vi "TrackingRedDot.vi"() -> ()   [LabVIEW 2024]
uses:
  <userlib>/ImageProcessing/IdentifyBlob_Square_Image.vi
panel:
  out "Array":cluster{"Numeric":dbl, "Numeric 2":dbl}[](array[cluster])=[{"Numeric"=343.3711790393013, "Numeric 2"=267.07423580786025}, {"Numeric"=337.0897435897436, "Numeric 2"=269.14102564102564}, {"Numeric"=335.8137651821862, "Numeric 2"=268.5991902834008}, {"Numeric"=343.1166666666667, "Numeric 2"=267.30833333333334}, {"Numeric"=348.0122448979592, "Numeric 2"=265.46530612244896}, {"Numeric"=344.37130801687766, "Numeric 2"=265.1898734177215}, {"Numeric"=338.55274261603375, "Numeric 2"=267.34599156118145}, {"Numeric"=337.68879668049794, "Numeric 2"=268.78008298755185}, {"Numeric"=340.15744680851066, "Numeric 2"=268.4382978723404}, {"Numeric"=345.2207792207792, "Numeric 2"=267.05627705627705}, {"Numeric"=343.76190476190476, "Numeric 2"=265.09090909090907}, {"Numeric"=340.12345679012344, "Numeric 2"=265.4074074074074}, {"Numeric"=340.2276422764228, "Numeric 2"=267.4349593495935}, {"Numeric"=341.6163793103448, "Numeric 2"=269.10775862068965}, {"Numeric"=341.60084033613447, "Numeric 2"=268.327731092437}, {"Numeric"=340.8185654008439, "Numeric 2"=266.56540084388183}, {"Numeric"=340.336170212766, "Numeric 2"=265.2893617021277}, {"Numeric"=341.6900826446281, "Numeric 2"=265.8636363636364}, {"Numeric"=342.0576131687243, "Numeric 2"=267.6296296296296}, {"Numeric"=340.67932489451476, "Numeric 2"=268.8270042194093}, {"Numeric"=339.1673640167364, "Numeric 2"=267.55648535564853}, {"Numeric"=339.72294372294374, "Numeric 2"=266.15584415584414}, {"Numeric"=341.9240506329114, "Numeric 2"=265.2742616033755}, {"Numeric"=343.8050847457627, "Numeric 2"=266.9364406779661}, {"Numeric"=342.1652892561983, "Numeric 2"=268.5}, {"Numeric"=338.8601694915254, "Numeric 2"=268.23728813559325}, {"Numeric"=338.6923076923077, "Numeric 2"=267.15811965811963}, {"Numeric"=343.2983870967742, "Numeric 2"=265.68951612903226}, {"Numeric"=345.4567901234568, "Numeric 2"=265.86831275720164}, {"Numeric"=343.94142259414224, "Numeric 2"=267.3305439330544}, {"Numeric"=338.93004115226336, "Numeric 2"=268.4320987654321}, {"Numeric"=337.390243902439, "Numeric 2"=267.7032520325203}, {"Numeric"=340.9665271966527, "Numeric 2"=266.7615062761506}, {"Numeric"=345.13675213675214, "Numeric 2"=266.15384615384613}, {"Numeric"=346.1016260162602, "Numeric 2"=265.7967479674797}, {"Numeric"=345.79918032786884, "Numeric 2"=266.2663934426229}, {"Numeric"=342.5042016806723, "Numeric 2"=267.06722689075633}, {"Numeric"=340.68595041322317, "Numeric 2"=267.4297520661157}, {"Numeric"=339.0365853658537, "Numeric 2"=267.760162601626}, {"Numeric"=338.1623931623932, "Numeric 2"=268.1025641025641}, {"Numeric"=338.4458333333333, "Numeric 2"=267.9625}, {"Numeric"=338.8691983122363, "Numeric 2"=267.9831223628692}, {"Numeric"=339.4268292682927, "Numeric 2"=267.5853658536585}, {"Numeric"=340.4530612244898, "Numeric 2"=267.52244897959184}, {"Numeric"=341.6302521008403, "Numeric 2"=267.33193277310926}, {"Numeric"=342.9958158995816, "Numeric 2"=266.74058577405856}, {"Numeric"=342.9958158995816, "Numeric 2"=266.74058577405856}, {"Numeric"=344.2236286919831, "Numeric 2"=266.55274261603375}, {"Numeric"=344.7909836065574, "Numeric 2"=266.4303278688525}, {"Numeric"=345.0468085106383, "Numeric 2"=266.2340425531915}, {"Numeric"=345.1603375527426, "Numeric 2"=266.0337552742616}, {"Numeric"=345.48319327731093, "Numeric 2"=265.99159663865544}, {"Numeric"=345.68200836820085, "Numeric 2"=265.9916317991632}, {"Numeric"=345.50416666666666, "Numeric 2"=266.0708333333333}, {"Numeric"=345.43388429752065, "Numeric 2"=265.91735537190084}, {"Numeric"=345.2307692307692, "Numeric 2"=265.83805668016197}, {"Numeric"=344.9428571428571, "Numeric 2"=265.869387755102}, {"Numeric"=344.5420168067227, "Numeric 2"=266.01680672268907}, {"Numeric"=344.4579831932773, "Numeric 2"=266.07142857142856}, {"Numeric"=344.26808510638296, "Numeric 2"=266.20851063829787}, {"Numeric"=343.61965811965814, "Numeric 2"=266.1880341880342}, {"Numeric"=343.0420168067227, "Numeric 2"=266.2352941176471}, {"Numeric"=342.40677966101697, "Numeric 2"=266.29661016949154}, {"Numeric"=342.1991701244813, "Numeric 2"=266.45228215767634}, {"Numeric"=341.6846473029046, "Numeric 2"=266.5435684647303}, {"Numeric"=341.12133891213387, "Numeric 2"=266.78661087866107}, {"Numeric"=340.73390557939916, "Numeric 2"=266.9785407725322}, {"Numeric"=339.8933333333333, "Numeric 2"=267.05333333333334}, {"Numeric"=339.8933333333333, "Numeric 2"=267.05333333333334}, {"Numeric"=339.60084033613447, "Numeric 2"=267.3067226890756}, {"Numeric"=339.5611814345992, "Numeric 2"=267.295358649789}, {"Numeric"=339.508064516129, "Numeric 2"=267.59274193548384}, {"Numeric"=339.4475806451613, "Numeric 2"=267.5443548387097}, {"Numeric"=339.4475806451613, "Numeric 2"=267.5443548387097}, {"Numeric"=339.16806722689074, "Numeric 2"=267.8151260504202}, {"Numeric"=339.3703703703704, "Numeric 2"=267.9835390946502}, {"Numeric"=339.45147679324896, "Numeric 2"=268.1940928270042}, {"Numeric"=339.63713080168776, "Numeric 2"=268.25738396624473}, {"Numeric"=340.12133891213387, "Numeric 2"=268.10460251046027}, {"Numeric"=339.9324894514768, "Numeric 2"=268.0590717299578}, {"Numeric"=340.11297071129707, "Numeric 2"=267.9623430962343}, {"Numeric"=341.198347107438, "Numeric 2"=268.004132231405}, {"Numeric"=341.6170212765957, "Numeric 2"=267.9404255319149}, {"Numeric"=342.01659751037346, "Numeric 2"=267.76348547717845}, {"Numeric"=342.0082304526749, "Numeric 2"=267.6872427983539}, {"Numeric"=342.5162601626016, "Numeric 2"=267.5609756097561}, {"Numeric"=342.5162601626016, "Numeric 2"=267.5609756097561}, {"Numeric"=342.8512396694215, "Numeric 2"=267.3801652892562}, {"Numeric"=342.8512396694215, "Numeric 2"=267.3801652892562}, {"Numeric"=343.22222222222223, "Numeric 2"=267.2478632478632}, {"Numeric"=343.10526315789474, "Numeric 2"=267.0043859649123}, {"Numeric"=343.0295358649789, "Numeric 2"=266.75949367088606}, {"Numeric"=343.5163934426229, "Numeric 2"=266.5983606557377}, {"Numeric"=343.64406779661016, "Numeric 2"=266.53389830508473}, {"Numeric"=343.6846473029046, "Numeric 2"=266.448132780083}, {"Numeric"=343.40677966101697, "Numeric 2"=266.33474576271186}, {"Numeric"=343.51724137931035, "Numeric 2"=266.2155172413793}, {"Numeric"=343.2436974789916, "Numeric 2"=265.93277310924367}, {"Numeric"=343.23770491803276, "Numeric 2"=265.8032786885246}, {"Numeric"=343.0082304526749, "Numeric 2"=265.8395061728395}, {"Numeric"=342.83613445378154, "Numeric 2"=265.80252100840335}, {"Numeric"=342.38429752066116, "Numeric 2"=265.72314049586777}, {"Numeric"=342.38429752066116, "Numeric 2"=265.72314049586777}, {"Numeric"=341.76050420168065, "Numeric 2"=265.6932773109244}, {"Numeric"=341.9, "Numeric 2"=265.8}, {"Numeric"=341.6848739495798, "Numeric 2"=265.94117647058823}, {"Numeric"=341.0219298245614, "Numeric 2"=266.1798245614035}, {"Numeric"=340.9957081545064, "Numeric 2"=266.2961373390558}, {"Numeric"=340.6864406779661, "Numeric 2"=266.385593220339}, {"Numeric"=340.2340425531915, "Numeric 2"=266.45106382978724}, {"Numeric"=340.4978902953587, "Numeric 2"=266.55274261603375}, {"Numeric"=340.24050632911394, "Numeric 2"=266.8565400843882}, {"Numeric"=340.54741379310343, "Numeric 2"=267.0689655172414}, {"Numeric"=340.53711790393015, "Numeric 2"=267.1528384279476}, {"Numeric"=340.49568965517244, "Numeric 2"=267.25}, {"Numeric"=340.49568965517244, "Numeric 2"=267.25}, {"Numeric"=340.61728395061726, "Numeric 2"=267.4650205761317}, {"Numeric"=340.5983606557377, "Numeric 2"=267.577868852459}, {"Numeric"=340.5983606557377, "Numeric 2"=267.577868852459}, {"Numeric"=341.33613445378154, "Numeric 2"=267.76050420168065}, {"Numeric"=341.44166666666666, "Numeric 2"=267.84166666666664}, {"Numeric"=341.6652719665272, "Numeric 2"=267.8619246861925}, {"Numeric"=341.6313559322034, "Numeric 2"=267.978813559322}, {"Numeric"=341.77292576419217, "Numeric 2"=268.2139737991266}, {"Numeric"=341.965367965368, "Numeric 2"=268.2294372294372}, {"Numeric"=341.93886462882097, "Numeric 2"=268.1877729257642}, {"Numeric"=342.1025641025641, "Numeric 2"=268.0726495726496}, {"Numeric"=342.3151260504202, "Numeric 2"=267.9621848739496}, {"Numeric"=342.0258620689655, "Numeric 2"=267.9439655172414}, {"Numeric"=342.3801652892562, "Numeric 2"=267.8388429752066}, {"Numeric"=342.3801652892562, "Numeric 2"=267.8388429752066}, {"Numeric"=342.2716049382716, "Numeric 2"=267.59670781893004}, {"Numeric"=342.4074074074074, "Numeric 2"=267.4156378600823}, {"Numeric"=342.4074074074074, "Numeric 2"=267.4156378600823}, {"Numeric"=342.10775862068965, "Numeric 2"=267.23706896551727}, {"Numeric"=342.2920353982301, "Numeric 2"=267.1061946902655}, {"Numeric"=342.2324561403509, "Numeric 2"=267.00877192982455}, {"Numeric"=342.14285714285717, "Numeric 2"=266.6344537815126}, {"Numeric"=341.89121338912133, "Numeric 2"=266.4728033472803}, {"Numeric"=341.864406779661, "Numeric 2"=266.34322033898303}, {"Numeric"=341.75536480686696, "Numeric 2"=266.2575107296137}, {"Numeric"=341.8663793103448, "Numeric 2"=266.2198275862069}, {"Numeric"=341.6523605150215, "Numeric 2"=266.15450643776825}, {"Numeric"=341.1965065502183, "Numeric 2"=266.07860262008734}, {"Numeric"=341.24896265560164, "Numeric 2"=265.8381742738589}, {"Numeric"=341.24896265560164, "Numeric 2"=265.8381742738589}, {"Numeric"=341.16170212765957, "Numeric 2"=265.88510638297873}, {"Numeric"=341.1673640167364, "Numeric 2"=265.93305439330544}, {"Numeric"=341.1673640167364, "Numeric 2"=265.93305439330544}, {"Numeric"=341.29957805907173, "Numeric 2"=266.084388185654}, {"Numeric"=341.46610169491527, "Numeric 2"=265.96610169491527}, {"Numeric"=341.4051724137931, "Numeric 2"=266.12931034482756}, {"Numeric"=341.3974358974359, "Numeric 2"=266.2393162393162}, {"Numeric"=341.50847457627117, "Numeric 2"=266.364406779661}, {"Numeric"=341.50622406639, "Numeric 2"=266.50622406639}, {"Numeric"=341.4813278008299, "Numeric 2"=266.53941908713693}, {"Numeric"=341.7375, "Numeric 2"=266.6333333333333}, {"Numeric"=341.7543859649123, "Numeric 2"=266.890350877193}, {"Numeric"=341.93886462882097, "Numeric 2"=267.117903930131}, {"Numeric"=342.10743801652893, "Numeric 2"=267.3223140495868}, {"Numeric"=342.22314049586777, "Numeric 2"=267.41735537190084}, {"Numeric"=342.27755102040817, "Numeric 2"=267.50204081632654}, {"Numeric"=342.27755102040817, "Numeric 2"=267.50204081632654}, {"Numeric"=342.30204081632655, "Numeric 2"=267.60816326530613}, {"Numeric"=342.15833333333336, "Numeric 2"=267.7875}, {"Numeric"=342.15833333333336, "Numeric 2"=267.7875}, {"Numeric"=342.2382978723404, "Numeric 2"=267.86382978723407}, {"Numeric"=342.0625, "Numeric 2"=267.9791666666667}, {"Numeric"=342.1125, "Numeric 2"=267.99583333333334}, {"Numeric"=341.9353448275862, "Numeric 2"=267.96120689655174}, {"Numeric"=341.9353448275862, "Numeric 2"=267.96120689655174}, {"Numeric"=341.78508771929825, "Numeric 2"=267.9342105263158}, {"Numeric"=341.9446808510638, "Numeric 2"=267.8553191489362}, {"Numeric"=341.5762711864407, "Numeric 2"=267.7542372881356}, {"Numeric"=341.422131147541, "Numeric 2"=267.655737704918}, {"Numeric"=341.1885245901639, "Numeric 2"=267.59016393442624}, {"Numeric"=341.3927125506073, "Numeric 2"=267.5344129554656}, {"Numeric"=341.4186991869919, "Numeric 2"=267.4227642276423}, {"Numeric"=341.07053941908714, "Numeric 2"=267.36099585062243}, {"Numeric"=341.07053941908714, "Numeric 2"=267.36099585062243}, {"Numeric"=340.7467248908297, "Numeric 2"=267.12663755458516}, {"Numeric"=340.48908296943233, "Numeric 2"=267.09170305676855}, {"Numeric"=340.85, "Numeric 2"=266.7916666666667}, {"Numeric"=340.98333333333335, "Numeric 2"=266.6}, {"Numeric"=340.8559670781893, "Numeric 2"=266.4691358024691}, {"Numeric"=340.74789915966386, "Numeric 2"=266.3487394957983}, {"Numeric"=341.390756302521, "Numeric 2"=266.23949579831935}, {"Numeric"=341.46351931330474, "Numeric 2"=266.137339055794}, {"Numeric"=341.7038626609442, "Numeric 2"=266.12875536480686}, {"Numeric"=341.868085106383, "Numeric 2"=266.16170212765957}, {"Numeric"=341.9008620689655, "Numeric 2"=265.9784482758621}, {"Numeric"=342.0882352941176, "Numeric 2"=265.8655462184874}, {"Numeric"=342.1589958158996, "Numeric 2"=265.89121338912133}, {"Numeric"=342.1589958158996, "Numeric 2"=265.89121338912133}, {"Numeric"=342.4848484848485, "Numeric 2"=266.13419913419915}, {"Numeric"=342.4848484848485, "Numeric 2"=266.13419913419915}, {"Numeric"=342.5875, "Numeric 2"=266.35833333333335}, {"Numeric"=342.9016393442623, "Numeric 2"=266.4139344262295}, {"Numeric"=343.172131147541, "Numeric 2"=266.4139344262295}, {"Numeric"=343.17083333333335, "Numeric 2"=266.525}, {"Numeric"=343.0548523206751, "Numeric 2"=266.6244725738397}, {"Numeric"=343.0940170940171, "Numeric 2"=266.9017094017094}, {"Numeric"=343.3404255319149, "Numeric 2"=266.92340425531916}, {"Numeric"=343.15384615384613, "Numeric 2"=267.1111111111111}, {"Numeric"=342.6666666666667, "Numeric 2"=267.22222222222223}, {"Numeric"=342.5708333333333, "Numeric 2"=267.3333333333333}, {"Numeric"=342.6138211382114, "Numeric 2"=267.479674796748}, {"Numeric"=342.4669421487603, "Numeric 2"=267.4876033057851}, {"Numeric"=342.16326530612247, "Numeric 2"=267.5795918367347}, {"Numeric"=342.16326530612247, "Numeric 2"=267.5795918367347}, {"Numeric"=341.7570850202429, "Numeric 2"=267.7004048582996}, {"Numeric"=341.4552845528455, "Numeric 2"=267.780487804878}, {"Numeric"=341.0532786885246, "Numeric 2"=267.89344262295083}, {"Numeric"=340.8481012658228, "Numeric 2"=267.9240506329114}, {"Numeric"=340.9504132231405, "Numeric 2"=267.88429752066116}, {"Numeric"=340.28979591836736, "Numeric 2"=267.85714285714283}, {"Numeric"=339.8125, "Numeric 2"=267.81666666666666}, {"Numeric"=339.9311740890688, "Numeric 2"=267.8137651821862}, {"Numeric"=339.796812749004, "Numeric 2"=267.75298804780874}, {"Numeric"=339.84313725490193, "Numeric 2"=267.7294117647059}, {"Numeric"=339.758064516129, "Numeric 2"=267.56048387096774}, {"Numeric"=339.77016129032256, "Numeric 2"=267.4556451612903}, {"Numeric"=339.38683127572017, "Numeric 2"=267.41975308641975}, {"Numeric"=339.6502057613169, "Numeric 2"=267.34567901234567}, {"Numeric"=339.6502057613169, "Numeric 2"=267.34567901234567}, {"Numeric"=340.1991341991342, "Numeric 2"=267.16450216450215}, {"Numeric"=340.0901287553648, "Numeric 2"=266.9442060085837}, {"Numeric"=340.3029045643153, "Numeric 2"=266.7842323651452}, {"Numeric"=340.7745901639344, "Numeric 2"=266.71311475409834}, {"Numeric"=341.4, "Numeric 2"=266.628}, {"Numeric"=341.74380165289256, "Numeric 2"=266.4710743801653}, {"Numeric"=342.14112903225805, "Numeric 2"=266.491935483871}, {"Numeric"=342.3469387755102, "Numeric 2"=266.42448979591836}, {"Numeric"=342.68879668049794, "Numeric 2"=266.3153526970954}, {"Numeric"=342.87916666666666, "Numeric 2"=266.3041666666667}, {"Numeric"=343.3375, "Numeric 2"=266.2416666666667}, {"Numeric"=343.8284518828452, "Numeric 2"=266.2887029288703}, {"Numeric"=344.1518987341772, "Numeric 2"=266.2320675105485}, {"Numeric"=344.1518987341772, "Numeric 2"=266.2320675105485}, {"Numeric"=344.37759336099583, "Numeric 2"=266.26970954356847}, {"Numeric"=344.2716049382716, "Numeric 2"=266.358024691358}, {"Numeric"=344.2716049382716, "Numeric 2"=266.358024691358}, {"Numeric"=344.3374485596708, "Numeric 2"=266.5102880658436}, {"Numeric"=344.55918367346936, "Numeric 2"=266.5265306122449}, {"Numeric"=344.35887096774195, "Numeric 2"=266.625}, {"Numeric"=343.9469387755102, "Numeric 2"=266.68979591836734}, {"Numeric"=343.62857142857143, "Numeric 2"=266.8122448979592}, {"Numeric"=343.8489795918367, "Numeric 2"=266.9673469387755}, {"Numeric"=343.13675213675214, "Numeric 2"=267.13675213675214}, {"Numeric"=342.55918367346936, "Numeric 2"=267.3265306122449}, {"Numeric"=342.37551020408165, "Numeric 2"=267.39591836734695}, {"Numeric"=342.0806451612903, "Numeric 2"=267.4032258064516}, {"Numeric"=341.7217741935484, "Numeric 2"=267.4193548387097}, {"Numeric"=341.7217741935484, "Numeric 2"=267.4193548387097}, {"Numeric"=340.9717741935484, "Numeric 2"=267.5806451612903}, {"Numeric"=340.9717741935484, "Numeric 2"=267.5806451612903}, {"Numeric"=340.09274193548384, "Numeric 2"=267.5766129032258}, {"Numeric"=339.6761133603239, "Numeric 2"=267.6356275303644}, {"Numeric"=339.5748987854251, "Numeric 2"=267.64777327935224}, {"Numeric"=339.28163265306125, "Numeric 2"=267.64897959183673}, {"Numeric"=339.356, "Numeric 2"=267.684}, {"Numeric"=339.352, "Numeric 2"=267.664}, {"Numeric"=339.3690476190476, "Numeric 2"=267.6746031746032}, {"Numeric"=339.425702811245, "Numeric 2"=267.5863453815261}, {"Numeric"=339.4096385542169, "Numeric 2"=267.56224899598396}, {"Numeric"=339.5381526104418, "Numeric 2"=267.52208835341366}, {"Numeric"=339.4837398373984, "Numeric 2"=267.4756097560976}, {"Numeric"=339.49794238683126, "Numeric 2"=267.40329218106996}, {"Numeric"=340.2510288065844, "Numeric 2"=267.3127572016461}, {"Numeric"=340.2510288065844, "Numeric 2"=267.3127572016461}, {"Numeric"=340.2832618025751, "Numeric 2"=267.20600858369096}, {"Numeric"=340.2832618025751, "Numeric 2"=267.20600858369096}, {"Numeric"=341.6163793103448, "Numeric 2"=267.0215517241379}, {"Numeric"=341.9460580912863, "Numeric 2"=266.8713692946058}, {"Numeric"=342.40408163265306, "Numeric 2"=266.7061224489796}, {"Numeric"=342.4238683127572, "Numeric 2"=266.60493827160496}, {"Numeric"=342.9268292682927, "Numeric 2"=266.5487804878049}, {"Numeric"=343.3636363636364, "Numeric 2"=266.4710743801653}, {"Numeric"=343.74074074074076, "Numeric 2"=266.4650205761317}, {"Numeric"=344.07851239669424, "Numeric 2"=266.3636363636364}, {"Numeric"=344.44897959183675, "Numeric 2"=266.3673469387755}, {"Numeric"=344.275, "Numeric 2"=266.32916666666665}, {"Numeric"=344.5514403292181, "Numeric 2"=266.3374485596708}, {"Numeric"=344.7975708502024, "Numeric 2"=266.33603238866397}, {"Numeric"=345.0161943319838, "Numeric 2"=266.4008097165992}, {"Numeric"=345.0161943319838, "Numeric 2"=266.4008097165992}, {"Numeric"=344.5162601626016, "Numeric 2"=266.4268292682927}, {"Numeric"=344.5162601626016, "Numeric 2"=266.4268292682927}, {"Numeric"=343.90909090909093, "Numeric 2"=266.5206611570248}, {"Numeric"=343.71311475409834, "Numeric 2"=266.59016393442624}, {"Numeric"=343.3780487804878, "Numeric 2"=266.6666666666667}, {"Numeric"=343.1166666666667, "Numeric 2"=266.7583333333333}, {"Numeric"=342.61087866108784, "Numeric 2"=266.7949790794979}, {"Numeric"=342.58264462809916, "Numeric 2"=267.0123966942149}, {"Numeric"=341.9230769230769, "Numeric 2"=267.12393162393164}, {"Numeric"=341.5208333333333, "Numeric 2"=267.2625}, {"Numeric"=341.18930041152265, "Numeric 2"=267.3168724279835}, {"Numeric"=340.9105691056911, "Numeric 2"=267.3983739837398}, {"Numeric"=340.4549180327869, "Numeric 2"=267.422131147541}, {"Numeric"=339.96311475409834, "Numeric 2"=267.46311475409834}, {"Numeric"=339.9236947791165, "Numeric 2"=267.4899598393574}, {"Numeric"=339.9236947791165, "Numeric 2"=267.4899598393574}, {"Numeric"=339.39676113360326, "Numeric 2"=267.58704453441294}, {"Numeric"=339.39676113360326, "Numeric 2"=267.58704453441294}, {"Numeric"=339.49402390438246, "Numeric 2"=267.62549800796813}, {"Numeric"=339.42971887550203, "Numeric 2"=267.6265060240964}, {"Numeric"=339.31474103585657, "Numeric 2"=267.6772908366534}, {"Numeric"=339.4016064257028, "Numeric 2"=267.6144578313253}, {"Numeric"=339.72332015810275, "Numeric 2"=267.57707509881425}, {"Numeric"=339.93975903614455, "Numeric 2"=267.5301204819277}, {"Numeric"=340.11290322580646, "Numeric 2"=267.508064516129}, {"Numeric"=340.2741935483871, "Numeric 2"=267.47983870967744}, {"Numeric"=340.72289156626505, "Numeric 2"=267.4497991967871}, {"Numeric"=340.8041666666667, "Numeric 2"=267.3666666666667}, {"Numeric"=341.1470588235294, "Numeric 2"=267.3781512605042}, {"Numeric"=341.60169491525426, "Numeric 2"=267.2542372881356}, {"Numeric"=341.60169491525426, "Numeric 2"=267.2542372881356}, {"Numeric"=342.235807860262, "Numeric 2"=267.08733624454146}, {"Numeric"=342.4173913043478, "Numeric 2"=266.9826086956522}, {"Numeric"=342.85470085470087, "Numeric 2"=266.85042735042737}, {"Numeric"=343.1908713692946, "Numeric 2"=266.76763485477176}, {"Numeric"=343.53909465020575, "Numeric 2"=266.63374485596705}, {"Numeric"=343.53688524590166, "Numeric 2"=266.5655737704918}, {"Numeric"=343.7357723577236, "Numeric 2"=266.4837398373984}, {"Numeric"=344.0569105691057, "Numeric 2"=266.4349593495935}, {"Numeric"=344.1633466135458, "Numeric 2"=266.47011952191235}, {"Numeric"=343.8024691358025, "Numeric 2"=266.46090534979425}, {"Numeric"=344.03688524590166, "Numeric 2"=266.405737704918}, {"Numeric"=343.3430962343096, "Numeric 2"=266.3682008368201}, {"Numeric"=343.5163934426229, "Numeric 2"=266.3688524590164}, {"Numeric"=343.5163934426229, "Numeric 2"=266.3688524590164}, {"Numeric"=343.07053941908714, "Numeric 2"=266.38589211618256}, {"Numeric"=342.7692307692308, "Numeric 2"=266.4412955465587}, {"Numeric"=342.7692307692308, "Numeric 2"=266.4412955465587}, {"Numeric"=342.0663900414938, "Numeric 2"=266.5103734439834}, {"Numeric"=342.0165289256198, "Numeric 2"=266.55371900826447}, {"Numeric"=342.0617283950617, "Numeric 2"=266.56378600823047}, {"Numeric"=341.80497925311204, "Numeric 2"=266.71784232365144}, {"Numeric"=341.56722689075633, "Numeric 2"=266.9159663865546}, {"Numeric"=341.0762711864407, "Numeric 2"=267.02542372881356}, {"Numeric"=341.0769230769231, "Numeric 2"=267.12393162393164}, {"Numeric"=340.864406779661, "Numeric 2"=267.18220338983053}, {"Numeric"=340.7154811715481, "Numeric 2"=267.2426778242678}, {"Numeric"=340.45454545454544, "Numeric 2"=267.3223140495868}, {"Numeric"=340.59591836734694, "Numeric 2"=267.4}, {"Numeric"=340.2107438016529, "Numeric 2"=267.4669421487603}, {"Numeric"=340.2107438016529, "Numeric 2"=267.4669421487603}, {"Numeric"=339.849593495935, "Numeric 2"=267.5487804878049}, {"Numeric"=340.2289156626506, "Numeric 2"=267.5421686746988}, {"Numeric"=340.2289156626506, "Numeric 2"=267.5421686746988}, {"Numeric"=340.544, "Numeric 2"=267.62}, {"Numeric"=340.96078431372547, "Numeric 2"=267.61176470588236}, {"Numeric"=340.788, "Numeric 2"=267.632}, {"Numeric"=341.06299212598424, "Numeric 2"=267.6102362204724}, {"Numeric"=341.4032258064516, "Numeric 2"=267.6209677419355}, {"Numeric"=341.5265306122449, "Numeric 2"=267.59183673469386}, {"Numeric"=341.753036437247, "Numeric 2"=267.55465587044534}, {"Numeric"=342.0688259109312, "Numeric 2"=267.5182186234818}, {"Numeric"=342.1061224489796, "Numeric 2"=267.43265306122447}, {"Numeric"=342.344262295082, "Numeric 2"=267.3811475409836}, {"Numeric"=342.4297520661157, "Numeric 2"=267.3388429752066}, {"Numeric"=342.4297520661157, "Numeric 2"=267.3388429752066}, {"Numeric"=342.53679653679654, "Numeric 2"=267.13852813852816}, {"Numeric"=342.53679653679654, "Numeric 2"=267.13852813852816}, {"Numeric"=342.67248908296943, "Numeric 2"=267.07423580786025}, {"Numeric"=343.0, "Numeric 2"=266.798353909465}, {"Numeric"=342.6487603305785, "Numeric 2"=266.70661157024796}, {"Numeric"=342.8979591836735, "Numeric 2"=266.69795918367345}, {"Numeric"=342.4590163934426, "Numeric 2"=266.6516393442623}, {"Numeric"=342.50205761316874, "Numeric 2"=266.49794238683126}, {"Numeric"=342.39256198347107, "Numeric 2"=266.4504132231405}, {"Numeric"=342.3305785123967, "Numeric 2"=266.4669421487603}, {"Numeric"=342.27385892116183, "Numeric 2"=266.43153526970957}, {"Numeric"=342.4375, "Numeric 2"=266.32916666666665}, {"Numeric"=342.2278481012658, "Numeric 2"=266.27848101265823}, {"Numeric"=342.02928870292885, "Numeric 2"=266.3305439330544}, {"Numeric"=341.70762711864404, "Numeric 2"=266.3050847457627}, {"Numeric"=341.70762711864404, "Numeric 2"=266.3050847457627}, {"Numeric"=341.5546218487395, "Numeric 2"=266.39915966386553}, {"Numeric"=341.5546218487395, "Numeric 2"=266.39915966386553}, {"Numeric"=341.4897119341564, "Numeric 2"=266.52263374485597}, {"Numeric"=341.33870967741933, "Numeric 2"=266.6008064516129}, {"Numeric"=341.2282157676349, "Numeric 2"=266.5850622406639}, {"Numeric"=341.1218487394958, "Numeric 2"=266.7268907563025}, {"Numeric"=341.125, "Numeric 2"=266.89166666666665}, {"Numeric"=340.8484848484849, "Numeric 2"=267.0865800865801}, {"Numeric"=341.0382978723404, "Numeric 2"=267.16170212765957}, {"Numeric"=341.1308016877637, "Numeric 2"=267.17721518987344}, {"Numeric"=340.9382716049383, "Numeric 2"=267.38271604938274}, {"Numeric"=340.9588477366255, "Numeric 2"=267.40329218106996}, {"Numeric"=341.4650205761317, "Numeric 2"=267.4238683127572}, {"Numeric"=341.1769547325103, "Numeric 2"=267.4691358024691}, {"Numeric"=341.1769547325103, "Numeric 2"=267.4691358024691}, {"Numeric"=341.7125506072874, "Numeric 2"=267.6072874493927}, {"Numeric"=341.7125506072874, "Numeric 2"=267.6072874493927}, {"Numeric"=341.8577235772358, "Numeric 2"=267.609756097561}, {"Numeric"=342.00409836065575, "Numeric 2"=267.6106557377049}, {"Numeric"=342.10699588477365, "Numeric 2"=267.6008230452675}, {"Numeric"=342.06611570247935, "Numeric 2"=267.6528925619835}, {"Numeric"=342.2408163265306, "Numeric 2"=267.56326530612245}, {"Numeric"=342.2439024390244, "Numeric 2"=267.6016260162602}, {"Numeric"=342.2995951417004, "Numeric 2"=267.6194331983806}, {"Numeric"=342.5524193548387, "Numeric 2"=267.5524193548387}, {"Numeric"=342.556, "Numeric 2"=267.456}, {"Numeric"=342.2581967213115, "Numeric 2"=267.39344262295083}, {"Numeric"=342.3402489626556, "Numeric 2"=267.344398340249}, {"Numeric"=342.40909090909093, "Numeric 2"=267.3305785123967}, {"Numeric"=342.3539094650206, "Numeric 2"=267.320987654321}, {"Numeric"=342.3539094650206, "Numeric 2"=267.320987654321}, {"Numeric"=342.45922746781116, "Numeric 2"=267.12017167381975}, {"Numeric"=342.45922746781116, "Numeric 2"=267.12017167381975}, {"Numeric"=342.15744680851066, "Numeric 2"=266.86382978723407}, {"Numeric"=342.15744680851066, "Numeric 2"=266.86382978723407}, {"Numeric"=342.15767634854774, "Numeric 2"=266.63900414937757}, {"Numeric"=342.0165289256198, "Numeric 2"=266.55371900826447}, {"Numeric"=341.8897959183673, "Numeric 2"=266.53877551020406}, {"Numeric"=341.82572614107886, "Numeric 2"=266.4190871369295}, {"Numeric"=341.7531380753138, "Numeric 2"=266.4142259414226}, {"Numeric"=341.5966386554622, "Numeric 2"=266.3697478991597}, {"Numeric"=341.6502057613169, "Numeric 2"=266.36625514403295}, {"Numeric"=341.71604938271605, "Numeric 2"=266.3539094650206}, {"Numeric"=341.89669421487605, "Numeric 2"=266.38429752066116}, {"Numeric"=341.8196721311475, "Numeric 2"=266.344262295082}, {"Numeric"=341.6188524590164, "Numeric 2"=266.422131147541}, {"Numeric"=341.760162601626, "Numeric 2"=266.4105691056911}, {"Numeric"=341.760162601626, "Numeric 2"=266.4105691056911}, {"Numeric"=341.72469635627533, "Numeric 2"=266.52226720647775}, {"Numeric"=341.5983606557377, "Numeric 2"=266.5614754098361}, {"Numeric"=342.0, "Numeric 2"=266.6}, {"Numeric"=341.8535564853556, "Numeric 2"=266.69456066945605}, {"Numeric"=341.93333333333334, "Numeric 2"=266.69166666666666}, {"Numeric"=341.97457627118644, "Numeric 2"=267.02542372881356}, {"Numeric"=342.1914893617021, "Numeric 2"=267.1489361702128}, {"Numeric"=342.29957805907173, "Numeric 2"=267.2067510548523}, {"Numeric"=342.12133891213387, "Numeric 2"=267.25941422594144}, {"Numeric"=341.905737704918, "Numeric 2"=267.3483606557377}, {"Numeric"=342.43145161290323, "Numeric 2"=267.43145161290323}, {"Numeric"=342.40725806451616, "Numeric 2"=267.4556451612903}, {"Numeric"=342.4837398373984, "Numeric 2"=267.4715447154472}, {"Numeric"=341.88284518828453, "Numeric 2"=268.4560669456067}, {"Numeric"=340.4, "Numeric 2"=270.60434782608695}, {"Numeric"=338.64761904761906, "Numeric 2"=274.95238095238096}, {"Numeric"=338.64761904761906, "Numeric 2"=274.95238095238096}, {"Numeric"=343.78966789667896, "Numeric 2"=287.4981549815498}, {"Numeric"=348.3813813813814, "Numeric 2"=293.1351351351351}, {"Numeric"=351.86053412462905, "Numeric 2"=297.7566765578635}, {"Numeric"=353.73926380368096, "Numeric 2"=300.70552147239266}, {"Numeric"=354.815625, "Numeric 2"=302.790625}, {"Numeric"=355.31888544891643, "Numeric 2"=304.55108359133123}, {"Numeric"=355.64119601328906, "Numeric 2"=306.3388704318937}, {"Numeric"=357.1266233766234, "Numeric 2"=307.3896103896104}, {"Numeric"=357.73926380368096, "Numeric 2"=307.59202453987734}, {"Numeric"=356.9971098265896, "Numeric 2"=306.21098265895955}, {"Numeric"=354.77971014492755, "Numeric 2"=303.76521739130436}, {"Numeric"=354.77971014492755, "Numeric 2"=303.76521739130436}, {"Numeric"=351.437125748503, "Numeric 2"=296.7365269461078}, {"Numeric"=351.437125748503, "Numeric 2"=296.7365269461078}, {"Numeric"=347.89020771513356, "Numeric 2"=288.85756676557867}, {"Numeric"=346.21965317919074, "Numeric 2"=284.0202312138728}, {"Numeric"=344.2122905027933, "Numeric 2"=278.41340782122904}, {"Numeric"=341.88338192419826, "Numeric 2"=272.20991253644314}, {"Numeric"=340.0221518987342, "Numeric 2"=266.0126582278481}, {"Numeric"=338.58245614035087, "Numeric 2"=260.40701754385964}, {"Numeric"=337.4981549815498, "Numeric 2"=255.31365313653134}, {"Numeric"=336.72243346007605, "Numeric 2"=250.35361216730035}, {"Numeric"=336.53333333333336, "Numeric 2"=245.47843137254904}, {"Numeric"=336.27710843373495, "Numeric 2"=240.75100401606426}, {"Numeric"=336.5022026431718, "Numeric 2"=236.36563876651985}, {"Numeric"=336.180412371134, "Numeric 2"=233.01546391752578}, {"Numeric"=336.180412371134, "Numeric 2"=233.01546391752578}, {"Numeric"=335.7631578947368, "Numeric 2"=229.4736842105263}, {"Numeric"=335.7631578947368, "Numeric 2"=229.4736842105263}, {"Numeric"=336.79411764705884, "Numeric 2"=228.79411764705884}, {"Numeric"=336.98148148148147, "Numeric 2"=229.32098765432102}, {"Numeric"=336.37142857142857, "Numeric 2"=230.6742857142857}, {"Numeric"=335.31176470588235, "Numeric 2"=232.86470588235295}, {"Numeric"=334.5257142857143, "Numeric 2"=236.16000000000003}, {"Numeric"=335.4752475247525, "Numeric 2"=240.09405940594058}, {"Numeric"=336.0219298245614, "Numeric 2"=244.32456140350877}, {"Numeric"=336.4364406779661, "Numeric 2"=248.864406779661}, {"Numeric"=336.6111111111111, "Numeric 2"=253.49603174603175}, {"Numeric"=337.07251908396944, "Numeric 2"=258.60687022900765}, {"Numeric"=338.09285714285716, "Numeric 2"=263.975}, {"Numeric"=340.07142857142856, "Numeric 2"=269.45}, {"Numeric"=341.6666666666667, "Numeric 2"=274.81666666666666}, {"Numeric"=341.6666666666667, "Numeric 2"=274.81666666666666}, {"Numeric"=344.4506578947368, "Numeric 2"=284.06907894736844}, {"Numeric"=344.4506578947368, "Numeric 2"=284.06907894736844}, {"Numeric"=347.9202657807309, "Numeric 2"=291.7707641196013}, {"Numeric"=349.29794520547944, "Numeric 2"=295.11301369863014}, {"Numeric"=350.8211920529801, "Numeric 2"=297.6622516556291}, {"Numeric"=351.8277027027027, "Numeric 2"=299.56418918918916}, {"Numeric"=352.6324503311258, "Numeric 2"=300.6092715231788}, {"Numeric"=352.7573770491803, "Numeric 2"=301.0393442622951}, {"Numeric"=352.9093851132686, "Numeric 2"=300.6472491909385}, {"Numeric"=352.1704918032787, "Numeric 2"=299.7344262295082}, {"Numeric"=351.6026058631922, "Numeric 2"=298.36156351791533}, {"Numeric"=350.7258566978193, "Numeric 2"=295.8753894080997}, {"Numeric"=348.73186119873816, "Numeric 2"=293.0914826498423}, {"Numeric"=347.996875, "Numeric 2"=289.521875}, {"Numeric"=346.4143302180685, "Numeric 2"=285.5669781931464}, {"Numeric"=346.4143302180685, "Numeric 2"=285.5669781931464}, {"Numeric"=343.59554140127386, "Numeric 2"=276.8343949044586}, {"Numeric"=343.59554140127386, "Numeric 2"=276.8343949044586}, {"Numeric"=340.8990228013029, "Numeric 2"=267.12703583061887}, {"Numeric"=339.8020833333333, "Numeric 2"=262.4270833333333}, {"Numeric"=339.0388692579505, "Numeric 2"=257.6219081272085}, {"Numeric"=338.71102661596956, "Numeric 2"=253.1634980988593}, {"Numeric"=338.0, "Numeric 2"=249.01999999999998}, {"Numeric"=337.90909090909093, "Numeric 2"=245.26859504132233}, {"Numeric"=337.58447488584477, "Numeric 2"=241.89497716894977}, {"Numeric"=337.8605769230769, "Numeric 2"=239.125}, {"Numeric"=337.87373737373736, "Numeric 2"=237.02020202020202}, {"Numeric"=337.8729281767956, "Numeric 2"=235.70718232044197}, {"Numeric"=338.2044198895028, "Numeric 2"=234.7292817679558}, {"Numeric"=337.7305389221557, "Numeric 2"=234.5329341317365}, {"Numeric"=337.5906432748538, "Numeric 2"=235.02923976608184}, {"Numeric"=337.6918604651163, "Numeric 2"=235.02325581395348}, {"Numeric"=336.87368421052633, "Numeric 2"=238.2578947368421}, {"Numeric"=336.88613861386136, "Numeric 2"=240.77227722772278}, {"Numeric"=336.8095238095238, "Numeric 2"=243.75714285714287}, {"Numeric"=336.76190476190476, "Numeric 2"=247.31904761904764}, {"Numeric"=336.9, "Numeric 2"=250.9391304347826}, {"Numeric"=337.2317073170732, "Numeric 2"=255.0609756097561}, {"Numeric"=337.90625, "Numeric 2"=259.3671875}, {"Numeric"=338.8703703703704, "Numeric 2"=263.75555555555553}, {"Numeric"=340.45, "Numeric 2"=268.26785714285717}, {"Numeric"=340.97872340425533, "Numeric 2"=272.5425531914894}, {"Numeric"=342.1896551724138, "Numeric 2"=276.6551724137931}, {"Numeric"=343.28373702422147, "Numeric 2"=280.4948096885813}, {"Numeric"=344.27027027027026, "Numeric 2"=284.2972972972973}, {"Numeric"=344.27027027027026, "Numeric 2"=284.2972972972973}, {"Numeric"=347.45733788395904, "Numeric 2"=290.17064846416383}, {"Numeric"=347.45733788395904, "Numeric 2"=290.17064846416383}, {"Numeric"=348.79505300353355, "Numeric 2"=294.0459363957597}, {"Numeric"=349.29655172413794, "Numeric 2"=295.0896551724138}, {"Numeric"=349.92957746478874, "Numeric 2"=295.5281690140845}, {"Numeric"=350.55743243243245, "Numeric 2"=295.46621621621625}, {"Numeric"=349.7337883959044, "Numeric 2"=295.0}, {"Numeric"=348.7630662020906, "Numeric 2"=293.7665505226481}, {"Numeric"=348.28327645051195, "Numeric 2"=291.84982935153585}, {"Numeric"=347.43771043771045, "Numeric 2"=289.3131313131313}, {"Numeric"=346.3478260869565, "Numeric 2"=286.54515050167225}, {"Numeric"=345.1756756756757, "Numeric 2"=283.4155405405405}, {"Numeric"=344.486301369863, "Numeric 2"=279.8150684931507}, {"Numeric"=342.9264214046823, "Numeric 2"=276.13377926421407}, {"Numeric"=342.9264214046823, "Numeric 2"=276.13377926421407}, {"Numeric"=341.2338129496403, "Numeric 2"=268.0143884892086}, {"Numeric"=340.8259259259259, "Numeric 2"=263.85925925925926}, {"Numeric"=339.98837209302326, "Numeric 2"=259.9186046511628}, {"Numeric"=339.42412451361866, "Numeric 2"=256.0856031128405}, {"Numeric"=339.2098765432099, "Numeric 2"=252.6090534979424}, {"Numeric"=338.8114754098361, "Numeric 2"=249.18442622950818}, {"Numeric"=338.5357142857143, "Numeric 2"=246.48214285714283}, {"Numeric"=338.54545454545456, "Numeric 2"=244.0956937799043}, {"Numeric"=338.54545454545456, "Numeric 2"=244.0956937799043}, {"Numeric"=338.6125654450262, "Numeric 2"=240.82722513089004}, {"Numeric"=338.77659574468083, "Numeric 2"=239.8404255319149}, {"Numeric"=338.20652173913044, "Numeric 2"=239.70108695652175}, {"Numeric"=338.3101604278075, "Numeric 2"=239.98930481283423}, {"Numeric"=338.02139037433153, "Numeric 2"=240.97860962566847}, {"Numeric"=337.6842105263158, "Numeric 2"=242.40526315789475}, {"Numeric"=337.6842105263158, "Numeric 2"=242.40526315789475}, {"Numeric"=337.4782608695652, "Numeric 2"=246.8695652173913}, {"Numeric"=337.4782608695652, "Numeric 2"=246.8695652173913}, {"Numeric"=337.49107142857144, "Numeric 2"=252.70535714285717}, {"Numeric"=337.7950819672131, "Numeric 2"=256.17622950819674}, {"Numeric"=338.748031496063, "Numeric 2"=259.8346456692913}, {"Numeric"=338.99619771863115, "Numeric 2"=263.4980988593156}, {"Numeric"=339.6281588447653, "Numeric 2"=267.2671480144404}, {"Numeric"=340.90225563909775, "Numeric 2"=270.906015037594}, {"Numeric"=341.4381625441696, "Numeric 2"=274.48763250883394}, {"Numeric"=342.3076923076923, "Numeric 2"=277.9267399267399}, {"Numeric"=343.5483870967742, "Numeric 2"=280.98924731182797}, {"Numeric"=344.6725352112676, "Numeric 2"=283.75704225352115}, {"Numeric"=345.36462093862815, "Numeric 2"=286.1335740072202}, {"Numeric"=346.3345070422535, "Numeric 2"=288.056338028169}, {"Numeric"=346.9113475177305, "Numeric 2"=289.86170212765956}, {"Numeric"=346.9113475177305, "Numeric 2"=289.86170212765956}, {"Numeric"=347.95588235294116, "Numeric 2"=291.30514705882354}, {"Numeric"=348.5345454545455, "Numeric 2"=291.30545454545455}, {"Numeric"=348.07608695652175, "Numeric 2"=290.90579710144925}, {"Numeric"=347.4892857142857, "Numeric 2"=289.90357142857147}, {"Numeric"=347.33449477351917, "Numeric 2"=288.2334494773519}, {"Numeric"=346.3859649122807, "Numeric 2"=286.5473684210526}, {"Numeric"=345.8315789473684, "Numeric 2"=284.0912280701755}, {"Numeric"=345.08191126279866, "Numeric 2"=281.41638225255974}, {"Numeric"=344.4055944055944, "Numeric 2"=278.3286713286713}, {"Numeric"=343.0613718411552, "Numeric 2"=275.1335740072202}, {"Numeric"=342.5091575091575, "Numeric 2"=271.8864468864469}, {"Numeric"=341.6195652173913, "Numeric 2"=268.3695652173913}, {"Numeric"=341.6195652173913, "Numeric 2"=268.3695652173913}, {"Numeric"=340.3560606060606, "Numeric 2"=261.4318181818182}, {"Numeric"=339.7578125, "Numeric 2"=258.1484375}, {"Numeric"=339.7578125, "Numeric 2"=258.1484375}, {"Numeric"=339.1434782608696, "Numeric 2"=252.46086956521737}, {"Numeric"=339.1434782608696, "Numeric 2"=252.46086956521737}, {"Numeric"=339.0607476635514, "Numeric 2"=247.95327102803736}, {"Numeric"=338.4682926829268, "Numeric 2"=246.14634146341461}, {"Numeric"=338.547263681592, "Numeric 2"=244.90049751243782}, {"Numeric"=338.42929292929296, "Numeric 2"=244.09090909090907}, {"Numeric"=338.5210526315789, "Numeric 2"=243.7263157894737}, {"Numeric"=338.37113402061857, "Numeric 2"=244.02061855670104}, {"Numeric"=338.44102564102565, "Numeric 2"=244.73846153846154}, {"Numeric"=337.95477386934675, "Numeric 2"=245.91959798994975}, {"Numeric"=338.0047846889952, "Numeric 2"=247.36842105263156}, {"Numeric"=337.7844036697248, "Numeric 2"=249.37155963302752}, {"Numeric"=337.6261261261261, "Numeric 2"=251.7117117117117}, {"Numeric"=337.9424778761062, "Numeric 2"=254.41150442477874}, {"Numeric"=337.9424778761062, "Numeric 2"=254.41150442477874}, {"Numeric"=338.93172690763055, "Numeric 2"=260.28915662650604}, {"Numeric"=338.93172690763055, "Numeric 2"=260.28915662650604}, {"Numeric"=339.95238095238096, "Numeric 2"=266.64102564102564}, {"Numeric"=340.87640449438203, "Numeric 2"=269.87265917602997}, {"Numeric"=341.5830258302583, "Numeric 2"=272.93357933579335}, {"Numeric"=342.2319391634981, "Numeric 2"=275.94296577946767}, {"Numeric"=343.2826086956522, "Numeric 2"=278.463768115942}, {"Numeric"=344.43682310469313, "Numeric 2"=280.942238267148}, {"Numeric"=345.14336917562724, "Numeric 2"=283.0358422939068}, {"Numeric"=345.7230215827338, "Numeric 2"=284.9352517985611}, {"Numeric"=346.43560606060606, "Numeric 2"=286.5530303030303}, {"Numeric"=346.956678700361, "Numeric 2"=287.2960288808664}, {"Numeric"=347.1397058823529, "Numeric 2"=287.8639705882353}, {"Numeric"=347.47292418772565, "Numeric 2"=287.913357400722}, {"Numeric"=347.47292418772565, "Numeric 2"=287.913357400722}, {"Numeric"=346.99638989169677, "Numeric 2"=286.8916967509025}, {"Numeric"=346.7918215613383, "Numeric 2"=285.6877323420074}, {"Numeric"=346.7918215613383, "Numeric 2"=285.6877323420074}, {"Numeric"=345.74911660777383, "Numeric 2"=282.0318021201414}, {"Numeric"=344.7335766423358, "Numeric 2"=279.8868613138686}, {"Numeric"=344.29411764705884, "Numeric 2"=277.2095588235294}, {"Numeric"=343.2293233082707, "Numeric 2"=274.80075187969925}, {"Numeric"=342.60074626865674, "Numeric 2"=271.8619402985075}, {"Numeric"=341.70454545454544, "Numeric 2"=268.8712121212121}, {"Numeric"=341.30337078651684, "Numeric 2"=265.82771535580525}, {"Numeric"=340.7011494252874, "Numeric 2"=262.86973180076626}, {"Numeric"=339.7171314741036, "Numeric 2"=259.9243027888446}, {"Numeric"=339.6333333333333, "Numeric 2"=257.4375}, {"Numeric"=339.3125, "Numeric 2"=254.92083333333335}, {"Numeric"=339.3125, "Numeric 2"=254.92083333333335}, {"Numeric"=338.6896551724138, "Numeric 2"=250.75431034482756}, {"Numeric"=338.8675799086758, "Numeric 2"=249.20547945205482}, {"Numeric"=338.8675799086758, "Numeric 2"=249.20547945205482}, {"Numeric"=338.28846153846155, "Numeric 2"=247.31730769230768}, {"Numeric"=338.47417840375584, "Numeric 2"=247.13615023474176}, {"Numeric"=338.32535885167465, "Numeric 2"=247.14832535885165}, {"Numeric"=338.39195979899495, "Numeric 2"=247.70854271356785}, {"Numeric"=338.2047619047619, "Numeric 2"=248.36666666666667}, {"Numeric"=337.96039603960395, "Numeric 2"=249.95049504950492}, {"Numeric"=337.9, "Numeric 2"=251.56363636363636}, {"Numeric"=337.68036529680364, "Numeric 2"=253.52511415525112}, {"Numeric"=338.40851063829786, "Numeric 2"=255.668085106383}, {"Numeric"=338.4765957446809, "Numeric 2"=258.31489361702126}, {"Numeric"=338.96, "Numeric 2"=260.708}, {"Numeric"=338.96, "Numeric 2"=260.708}, {"Numeric"=340.2164179104478, "Numeric 2"=266.14925373134326}, {"Numeric"=340.2164179104478, "Numeric 2"=266.14925373134326}, {"Numeric"=341.6222222222222, "Numeric 2"=271.84444444444443}, {"Numeric"=342.52272727272725, "Numeric 2"=274.17424242424244}, {"Numeric"=343.07547169811323, "Numeric 2"=276.7245283018868}, {"Numeric"=344.0405904059041, "Numeric 2"=278.77859778597787}, {"Numeric"=344.99610894941634, "Numeric 2"=280.57587548638134}, {"Numeric"=345.7028985507246, "Numeric 2"=282.1811594202899}, {"Numeric"=346.24163568773236, "Numeric 2"=283.4423791821562}, {"Numeric"=346.12109375, "Numeric 2"=284.609375}, {"Numeric"=347.03663003663, "Numeric 2"=284.87545787545787}, {"Numeric"=347.13138686131384, "Numeric 2"=285.03284671532845}, {"Numeric"=346.9398496240602, "Numeric 2"=284.77443609022555}, {"Numeric"=346.8533834586466, "Numeric 2"=284.1616541353384}, {"Numeric"=346.4612546125461, "Numeric 2"=283.09594095940963}, {"Numeric"=346.4612546125461, "Numeric 2"=283.09594095940963}, {"Numeric"=345.3071161048689, "Numeric 2"=280.1498127340824}, {"Numeric"=344.60820895522386, "Numeric 2"=278.2276119402985}, {"Numeric"=343.848, "Numeric 2"=276.3}, {"Numeric"=343.2442748091603, "Numeric 2"=273.91603053435114}, {"Numeric"=342.6628787878788, "Numeric 2"=271.38257575757575}, {"Numeric"=341.97014925373134, "Numeric 2"=269.0}, {"Numeric"=341.48828125, "Numeric 2"=266.30859375}, {"Numeric"=340.56224899598396, "Numeric 2"=263.82730923694777}, {"Numeric"=339.9142857142857, "Numeric 2"=261.5469387755102}, {"Numeric"=339.6877637130802, "Numeric 2"=259.28270042194094}, {"Numeric"=339.5940170940171, "Numeric 2"=256.9316239316239}, {"Numeric"=339.6, "Numeric 2"=256.9148936170213}, {"Numeric"=338.7111111111111, "Numeric 2"=253.3822222222222}, {"Numeric"=338.3611111111111, "Numeric 2"=252.06481481481484}, {"Numeric"=338.3611111111111, "Numeric 2"=252.06481481481484}, {"Numeric"=338.6046511627907, "Numeric 2"=250.2046511627907}, {"Numeric"=338.6046511627907, "Numeric 2"=250.2046511627907}, {"Numeric"=338.6, "Numeric 2"=249.93333333333334}, {"Numeric"=338.38425925925924, "Numeric 2"=250.212962962963}, {"Numeric"=338.16901408450707, "Numeric 2"=251.02816901408448}, {"Numeric"=337.9530516431925, "Numeric 2"=252.15492957746477}, {"Numeric"=338.36199095022624, "Numeric 2"=253.48416289592762}, {"Numeric"=338.7787610619469, "Numeric 2"=255.1725663716814}, {"Numeric"=338.91150442477874, "Numeric 2"=257.06637168141594}, {"Numeric"=339.15611814345993, "Numeric 2"=259.09282700421943}, {"Numeric"=339.61507936507934, "Numeric 2"=261.218253968254}, {"Numeric"=339.9714285714286, "Numeric 2"=263.61224489795916}, {"Numeric"=340.70703125, "Numeric 2"=265.859375}, {"Numeric"=341.3968871595331, "Numeric 2"=268.3540856031128}, {"Numeric"=342.0980392156863, "Numeric 2"=270.5764705882353}, {"Numeric"=342.73880597014926, "Numeric 2"=272.82835820895525}, {"Numeric"=342.73880597014926, "Numeric 2"=272.82835820895525}, {"Numeric"=343.98501872659176, "Numeric 2"=276.8426966292135}, {"Numeric"=344.96875, "Numeric 2"=278.5546875}, {"Numeric"=345.37827715355803, "Numeric 2"=279.87265917602997}, {"Numeric"=345.8745247148289, "Numeric 2"=281.0266159695817}, {"Numeric"=346.06439393939394, "Numeric 2"=281.8219696969697}, {"Numeric"=346.0153256704981, "Numeric 2"=282.48659003831415}, {"Numeric"=346.3657587548638, "Numeric 2"=282.5486381322957}, {"Numeric"=346.171875, "Numeric 2"=282.52734375}, {"Numeric"=346.02661596958177, "Numeric 2"=281.88212927756655}, {"Numeric"=345.69083969465646, "Numeric 2"=281.10687022900765}, {"Numeric"=345.3308270676692, "Numeric 2"=279.9135338345865}, {"Numeric"=345.0380228136882, "Numeric 2"=278.6425855513308}, {"Numeric"=345.0380228136882, "Numeric 2"=278.6425855513308}, {"Numeric"=343.29615384615386, "Numeric 2"=275.30384615384617}, {"Numeric"=343.29615384615386, "Numeric 2"=275.30384615384617}, {"Numeric"=341.8452830188679, "Numeric 2"=271.1622641509434}, {"Numeric"=341.4826254826255, "Numeric 2"=269.03861003861005}, {"Numeric"=340.59375, "Numeric 2"=266.85546875}, {"Numeric"=340.2642276422764, "Numeric 2"=264.6260162601626}, {"Numeric"=339.79423868312756, "Numeric 2"=262.50205761316874}, {"Numeric"=339.41632653061225, "Numeric 2"=260.50612244897957}, {"Numeric"=338.71120689655174, "Numeric 2"=258.61206896551727}, {"Numeric"=338.69545454545454, "Numeric 2"=257.0}, {"Numeric"=338.6336206896552, "Numeric 2"=255.36637931034483}, {"Numeric"=338.80269058295966, "Numeric 2"=254.1659192825112}, {"Numeric"=338.61971830985914, "Numeric 2"=253.19248826291079}, {"Numeric"=338.88584474885846, "Numeric 2"=252.4931506849315}, {"Numeric"=338.77314814814815, "Numeric 2"=252.18981481481484}, {"Numeric"=338.77314814814815, "Numeric 2"=252.18981481481484}, {"Numeric"=338.8493150684931, "Numeric 2"=252.37899543378995}, {"Numeric"=338.8867924528302, "Numeric 2"=253.07547169811323}, {"Numeric"=338.98617511520735, "Numeric 2"=253.9953917050691}, {"Numeric"=339.09417040358744, "Numeric 2"=255.11659192825113}, {"Numeric"=339.47435897435895, "Numeric 2"=256.44444444444446}, {"Numeric"=339.47435897435895, "Numeric 2"=256.44444444444446}, {"Numeric"=340.22633744855966, "Numeric 2"=259.7818930041152}, {"Numeric"=340.75206611570246, "Numeric 2"=261.64462809917353}, {"Numeric"=340.9504132231405, "Numeric 2"=263.6322314049587}, {"Numeric"=341.7051792828685, "Numeric 2"=265.59760956175296}, {"Numeric"=341.8828125, "Numeric 2"=267.75}, {"Numeric"=342.7837837837838, "Numeric 2"=269.6911196911197}, {"Numeric"=343.25096525096524, "Numeric 2"=271.73359073359075}, {"Numeric"=343.82745098039214, "Numeric 2"=273.5686274509804}, {"Numeric"=344.132, "Numeric 2"=275.208}, {"Numeric"=345.0627450980392, "Numeric 2"=276.6}, {"Numeric"=345.0627450980392, "Numeric 2"=276.6}, {"Numeric"=345.39080459770116, "Numeric 2"=278.911877394636}, {"Numeric"=345.58365758754866, "Numeric 2"=279.6809338521401}, {"Numeric"=345.4653846153846, "Numeric 2"=280.20384615384614}, {"Numeric"=345.8178294573643, "Numeric 2"=280.52713178294573}, {"Numeric"=345.8030303030303, "Numeric 2"=280.31060606060606}, {"Numeric"=345.4465648854962, "Numeric 2"=279.82824427480915}, {"Numeric"=345.1547619047619, "Numeric 2"=279.37698412698415}, {"Numeric"=344.3190661478599, "Numeric 2"=278.5136186770428}, {"Numeric"=343.73046875, "Numeric 2"=277.46875}, {"Numeric"=343.18918918918916, "Numeric 2"=276.023166023166}, {"Numeric"=342.515625, "Numeric 2"=274.55859375}, {"Numeric"=342.15234375, "Numeric 2"=272.6953125}, {"Numeric"=342.15234375, "Numeric 2"=272.6953125}, {"Numeric"=341.04938271604937, "Numeric 2"=269.3127572016461}, {"Numeric"=341.04938271604937, "Numeric 2"=269.3127572016461}, {"Numeric"=339.7883817427386, "Numeric 2"=265.3900414937759}, {"Numeric"=339.7883817427386, "Numeric 2"=265.3900414937759}, {"Numeric"=338.8091286307054, "Numeric 2"=261.71784232365144}, {"Numeric"=338.9475982532751, "Numeric 2"=260.1484716157205}, {"Numeric"=338.88646288209605, "Numeric 2"=258.5720524017467}, {"Numeric"=338.9869565217391, "Numeric 2"=257.2217391304348}, {"Numeric"=338.7085201793722, "Numeric 2"=256.15246636771303}, {"Numeric"=339.0488888888889, "Numeric 2"=255.21777777777777}, {"Numeric"=338.868778280543, "Numeric 2"=254.710407239819}, {"Numeric"=338.6792452830189, "Numeric 2"=254.19339622641508}, {"Numeric"=339.13615023474176, "Numeric 2"=254.1032863849765}, {"Numeric"=339.5315315315315, "Numeric 2"=254.30630630630628}, {"Numeric"=339.3796296296296, "Numeric 2"=254.95833333333331}, {"Numeric"=339.6140350877193, "Numeric 2"=255.42543859649123}, {"Numeric"=339.52863436123346, "Numeric 2"=255.43171806167402}, {"Numeric"=340.0720338983051, "Numeric 2"=257.6271186440678}, {"Numeric"=340.35135135135135, "Numeric 2"=259.06306306306305}, {"Numeric"=341.24590163934425, "Numeric 2"=260.4467213114754}, {"Numeric"=341.7081545064378, "Numeric 2"=262.16309012875536}, {"Numeric"=341.89112903225805, "Numeric 2"=263.7096774193548}, {"Numeric"=342.1847389558233, "Numeric 2"=265.46586345381525}, {"Numeric"=342.33067729083666, "Numeric 2"=267.52589641434264}, {"Numeric"=342.68163265306123, "Numeric 2"=269.1795918367347}, {"Numeric"=343.61867704280155, "Numeric 2"=270.6420233463035}, {"Numeric"=343.798418972332, "Numeric 2"=272.4782608695652}, {"Numeric"=344.44787644787647, "Numeric 2"=273.7799227799228}, {"Numeric"=344.6756756756757, "Numeric 2"=275.0733590733591}, {"Numeric"=344.5925925925926, "Numeric 2"=276.358024691358}, {"Numeric"=344.5925925925926, "Numeric 2"=276.358024691358}, {"Numeric"=345.54135338345867, "Numeric 2"=277.8233082706767}, {"Numeric"=345.54135338345867, "Numeric 2"=277.8233082706767}, {"Numeric"=345.41984732824426, "Numeric 2"=278.6412213740458}, {"Numeric"=345.30651340996167, "Numeric 2"=278.6130268199234}, {"Numeric"=344.292, "Numeric 2"=278.432}, {"Numeric"=344.35769230769233, "Numeric 2"=277.75384615384615}, {"Numeric"=344.00763358778624, "Numeric 2"=277.1145038167939}, {"Numeric"=343.54545454545456, "Numeric 2"=276.3320158102767}, {"Numeric"=342.85114503816794, "Numeric 2"=274.9580152671756}, {"Numeric"=342.36821705426354, "Numeric 2"=273.7248062015504}, {"Numeric"=341.77016129032256, "Numeric 2"=272.43548387096774}, {"Numeric"=341.1333333333333, "Numeric 2"=270.7294117647059}, {"Numeric"=340.87044534412956, "Numeric 2"=269.2995951417004}, {"Numeric"=340.26693227091636, "Numeric 2"=267.56972111553785}, {"Numeric"=339.46153846153845, "Numeric 2"=265.7570850202429}, {"Numeric"=339.46153846153845, "Numeric 2"=265.7570850202429}, {"Numeric"=339.344262295082, "Numeric 2"=262.6311475409836}, {"Numeric"=338.94827586206895, "Numeric 2"=261.30172413793105}, {"Numeric"=338.94827586206895, "Numeric 2"=261.30172413793105}, {"Numeric"=338.96, "Numeric 2"=258.72}, {"Numeric"=338.81974248927037, "Numeric 2"=257.6137339055794}, {"Numeric"=339.4052863436123, "Numeric 2"=257.00881057268725}, {"Numeric"=339.08597285067873, "Numeric 2"=256.2533936651584}, {"Numeric"=339.09722222222223, "Numeric 2"=255.99537037037038}, {"Numeric"=339.33488372093024, "Numeric 2"=255.89767441860465}, {"Numeric"=339.6606334841629, "Numeric 2"=256.0316742081448}, {"Numeric"=339.95535714285717, "Numeric 2"=256.24107142857144}, {"Numeric"=340.14932126696834, "Numeric 2"=256.9683257918552}, {"Numeric"=340.61206896551727, "Numeric 2"=257.54741379310343}, {"Numeric"=340.79574468085104, "Numeric 2"=258.58297872340427}, {"Numeric"=341.2067510548523, "Numeric 2"=259.60759493670884}, {"Numeric"=341.57201646090533, "Numeric 2"=260.81481481481484}, {"Numeric"=341.57201646090533, "Numeric 2"=260.81481481481484}, {"Numeric"=341.7717842323651, "Numeric 2"=263.78008298755185}, {"Numeric"=342.18145161290323, "Numeric 2"=265.46370967741933}, {"Numeric"=342.17622950819674, "Numeric 2"=267.08196721311475}, {"Numeric"=343.0398406374502, "Numeric 2"=268.56175298804783}, {"Numeric"=343.0398406374502, "Numeric 2"=268.56175298804783}, {"Numeric"=343.8, "Numeric 2"=271.436}, {"Numeric"=343.98837209302326, "Numeric 2"=272.72093023255815}, {"Numeric"=344.62745098039215, "Numeric 2"=273.9450980392157}, {"Numeric"=344.5984555984556, "Numeric 2"=274.976833976834}, {"Numeric"=344.69260700389106, "Numeric 2"=275.8599221789883}, {"Numeric"=344.7707509881423, "Numeric 2"=276.4624505928854}, {"Numeric"=344.46946564885496, "Numeric 2"=277.0}, {"Numeric"=344.47011952191235, "Numeric 2"=277.3227091633466}, {"Numeric"=344.47011952191235, "Numeric 2"=277.3227091633466}, {"Numeric"=344.0038314176245, "Numeric 2"=277.0498084291188}, {"Numeric"=343.78846153846155, "Numeric 2"=276.61538461538464}, {"Numeric"=343.2655601659751, "Numeric 2"=276.2240663900415}, {"Numeric"=342.6144578313253, "Numeric 2"=275.45381526104416}, {"Numeric"=342.82608695652175, "Numeric 2"=274.39130434782606}, {"Numeric"=342.1843137254902, "Numeric 2"=273.32941176470587}, {"Numeric"=341.632, "Numeric 2"=271.896}, {"Numeric"=341.33858267716533, "Numeric 2"=270.5472440944882}, {"Numeric"=341.0987654320988, "Numeric 2"=269.2921810699589}, {"Numeric"=340.7578125, "Numeric 2"=267.7265625}, {"Numeric"=340.53061224489795, "Numeric 2"=266.38775510204084}, {"Numeric"=340.1781376518219, "Numeric 2"=264.7287449392713}, {"Numeric"=340.1781376518219, "Numeric 2"=264.7287449392713}, {"Numeric"=339.48458149779736, "Numeric 2"=262.15859030837004}, {"Numeric"=339.48458149779736, "Numeric 2"=262.15859030837004}, {"Numeric"=339.54741379310343, "Numeric 2"=259.87931034482756}, {"Numeric"=339.50228310502285, "Numeric 2"=258.986301369863}, {"Numeric"=339.51785714285717, "Numeric 2"=258.1875}, {"Numeric"=339.82758620689657, "Numeric 2"=257.5301724137931}, {"Numeric"=340.1030042918455, "Numeric 2"=257.24463519313304}, {"Numeric"=340.00881057268725, "Numeric 2"=257.13656387665196}, {"Numeric"=340.2246696035242, "Numeric 2"=257.1541850220264}, {"Numeric"=340.3083700440529, "Numeric 2"=257.40088105726875}, {"Numeric"=340.46875, "Numeric 2"=258.0357142857143}, {"Numeric"=340.4035087719298, "Numeric 2"=258.5438596491228}, {"Numeric"=340.55364806866953, "Numeric 2"=259.3648068669528}, {"Numeric"=341.25847457627117, "Numeric 2"=260.3262711864407}, {"Numeric"=340.982905982906, "Numeric 2"=261.5042735042735}, {"Numeric"=341.66390041493776, "Numeric 2"=262.6929460580913}, {"Numeric"=341.66390041493776, "Numeric 2"=262.6929460580913}, {"Numeric"=342.134693877551, "Numeric 2"=265.35510204081635}, {"Numeric"=342.134693877551, "Numeric 2"=265.35510204081635}, {"Numeric"=342.5529411764706, "Numeric 2"=268.1294117647059}, {"Numeric"=342.9442231075697, "Numeric 2"=269.52988047808765}, {"Numeric"=343.1699604743083, "Numeric 2"=270.62450592885375}, {"Numeric"=343.4921875, "Numeric 2"=271.81640625}, {"Numeric"=343.6692913385827, "Numeric 2"=272.76771653543307}, {"Numeric"=343.86821705426354, "Numeric 2"=273.9031007751938}, {"Numeric"=343.79457364341084, "Numeric 2"=274.6666666666667}, {"Numeric"=343.77911646586347, "Numeric 2"=275.4096385542169}, {"Numeric"=343.9140625, "Numeric 2"=275.68359375}, {"Numeric"=343.9268292682927, "Numeric 2"=276.0121951219512}, {"Numeric"=344.0241935483871, "Numeric 2"=276.10887096774195}, {"Numeric"=343.5863453815261, "Numeric 2"=275.83935742971886}, {"Numeric"=343.472, "Numeric 2"=275.56}, {"Numeric"=343.472, "Numeric 2"=275.56}, {"Numeric"=342.7991967871486, "Numeric 2"=274.4457831325301}, {"Numeric"=342.7991967871486, "Numeric 2"=274.4457831325301}, {"Numeric"=342.0438247011952, "Numeric 2"=272.55378486055776}, {"Numeric"=342.14112903225805, "Numeric 2"=271.47983870967744}, {"Numeric"=341.80971659919027, "Numeric 2"=270.3886639676113}, {"Numeric"=341.80971659919027, "Numeric 2"=270.3886639676113}, {"Numeric"=341.3050193050193, "Numeric 2"=267.7760617760618}, {"Numeric"=340.4959677419355, "Numeric 2"=266.5282258064516}, {"Numeric"=340.58995815899584, "Numeric 2"=265.2970711297071}, {"Numeric"=340.3636363636364, "Numeric 2"=264.04329004329}, {"Numeric"=340.2572614107884, "Numeric 2"=262.68879668049794}, {"Numeric"=339.831223628692, "Numeric 2"=261.70042194092827}, {"Numeric"=339.97095435684645, "Numeric 2"=260.597510373444}, {"Numeric"=339.52941176470586, "Numeric 2"=259.99547511312215}, {"Numeric"=339.8086956521739, "Numeric 2"=259.18260869565216}, {"Numeric"=339.84090909090907, "Numeric 2"=258.8727272727273}, {"Numeric"=339.84090909090907, "Numeric 2"=258.8727272727273}, {"Numeric"=339.96875, "Numeric 2"=258.23214285714283}, {"Numeric"=339.98230088495575, "Numeric 2"=258.24778761061947}, {"Numeric"=340.3348017621145, "Numeric 2"=258.43612334801765}, {"Numeric"=340.16818181818184, "Numeric 2"=258.9409090909091}, {"Numeric"=340.4069264069264, "Numeric 2"=259.3982683982684}, {"Numeric"=340.75, "Numeric 2"=260.11842105263156}, {"Numeric"=340.57456140350877, "Numeric 2"=261.140350877193}, {"Numeric"=340.7284482758621, "Numeric 2"=262.16379310344826}, {"Numeric"=341.02608695652174, "Numeric 2"=263.12608695652176}, {"Numeric"=341.13304721030045, "Numeric 2"=264.2360515021459}, {"Numeric"=341.5406504065041, "Numeric 2"=265.4065040650407}, {"Numeric"=341.551867219917, "Numeric 2"=266.6182572614108}, {"Numeric"=341.551867219917, "Numeric 2"=266.6182572614108}, {"Numeric"=342.2090163934426, "Numeric 2"=269.094262295082}, {"Numeric"=342.27755102040817, "Numeric 2"=270.2857142857143}, {"Numeric"=342.37301587301585, "Numeric 2"=271.24603174603175}, {"Numeric"=342.4756097560976, "Numeric 2"=272.3617886178862}, {"Numeric"=342.76771653543307, "Numeric 2"=273.0196850393701}, {"Numeric"=343.51171875, "Numeric 2"=273.7734375}, {"Numeric"=343.7716535433071, "Numeric 2"=274.4488188976378}, {"Numeric"=343.6860465116279, "Numeric 2"=274.7248062015504}, {"Numeric"=343.7003891050584, "Numeric 2"=274.8365758754864}, {"Numeric"=343.7265625, "Numeric 2"=275.046875}, {"Numeric"=343.712, "Numeric 2"=275.148}, {"Numeric"=343.8473282442748, "Numeric 2"=274.58015267175574}, {"Numeric"=342.984, "Numeric 2"=274.084}, {"Numeric"=342.984, "Numeric 2"=274.084}, {"Numeric"=342.92578125, "Numeric 2"=272.7265625}, {"Numeric"=342.92578125, "Numeric 2"=272.7265625}, {"Numeric"=342.14741035856576, "Numeric 2"=270.70916334661354}, {"Numeric"=342.46963562753035, "Numeric 2"=269.7611336032389}, {"Numeric"=342.281124497992, "Numeric 2"=268.76305220883535}, {"Numeric"=341.31983805668017, "Numeric 2"=267.44534412955466}, {"Numeric"=340.54811715481173, "Numeric 2"=266.38912133891216}, {"Numeric"=341.0386266094421, "Numeric 2"=265.2961373390558}, {"Numeric"=341.20425531914896, "Numeric 2"=264.16595744680853}, {"Numeric"=340.04366812227073, "Numeric 2"=263.10480349344977}, {"Numeric"=339.9059829059829, "Numeric 2"=262.1923076923077}, {"Numeric"=340.2928870292887, "Numeric 2"=261.4225941422594}, {"Numeric"=339.6735537190083, "Numeric 2"=260.54545454545456}, {"Numeric"=339.2938596491228, "Numeric 2"=260.0833333333333}, {"Numeric"=339.0468085106383, "Numeric 2"=259.6808510638298}, {"Numeric"=339.0468085106383, "Numeric 2"=259.6808510638298}, {"Numeric"=338.7354260089686, "Numeric 2"=259.21973094170403}, {"Numeric"=338.7354260089686, "Numeric 2"=259.21973094170403}, {"Numeric"=339.1484716157205, "Numeric 2"=259.4192139737991}, {"Numeric"=339.2914798206278, "Numeric 2"=260.0134529147982}, {"Numeric"=339.08898305084745, "Numeric 2"=260.3686440677966}, {"Numeric"=339.27659574468083, "Numeric 2"=260.9191489361702}, {"Numeric"=339.2274678111588, "Numeric 2"=261.725321888412}, {"Numeric"=339.55648535564853, "Numeric 2"=262.5230125523013}, {"Numeric"=339.4177215189873, "Numeric 2"=263.5021097046413}, {"Numeric"=340.1975308641975, "Numeric 2"=264.4320987654321}, {"Numeric"=340.7642276422764, "Numeric 2"=265.479674796748}, {"Numeric"=340.48163265306124, "Numeric 2"=266.56326530612245}, {"Numeric"=340.3625498007968, "Numeric 2"=267.6772908366534}, {"Numeric"=341.4448818897638, "Numeric 2"=268.81102362204723}, {"Numeric"=341.8192771084337, "Numeric 2"=269.82329317269074}, {"Numeric"=341.8192771084337, "Numeric 2"=269.82329317269074}, {"Numeric"=342.19444444444446, "Numeric 2"=271.6507936507937}, {"Numeric"=342.19444444444446, "Numeric 2"=271.6507936507937}, {"Numeric"=342.0409836065574, "Numeric 2"=273.4139344262295}, {"Numeric"=342.64478764478764, "Numeric 2"=273.7142857142857}, {"Numeric"=342.45, "Numeric 2"=274.2125}, {"Numeric"=342.47755102040816, "Numeric 2"=274.40816326530614}, {"Numeric"=342.18145161290323, "Numeric 2"=274.43951612903226}, {"Numeric"=342.3319502074689, "Numeric 2"=274.2655601659751}, {"Numeric"=342.2520325203252, "Numeric 2"=273.9186991869919}, {"Numeric"=342.19354838709677, "Numeric 2"=273.52016129032256}, {"Numeric"=342.3607843137255, "Numeric 2"=272.71372549019605}, {"Numeric"=341.8360655737705, "Numeric 2"=272.34016393442624}, {"Numeric"=341.9392712550607, "Numeric 2"=271.4574898785425}, {"Numeric"=341.3790322580645, "Numeric 2"=270.5443548387097}, {"Numeric"=341.3174603174603, "Numeric 2"=269.5674603174603}, {"Numeric"=341.3174603174603, "Numeric 2"=269.5674603174603}, {"Numeric"=340.3333333333333, "Numeric 2"=267.5284552845528}, {"Numeric"=340.3333333333333, "Numeric 2"=267.5284552845528}, {"Numeric"=339.6761133603239, "Numeric 2"=265.54655870445345}, {"Numeric"=339.23651452282155, "Numeric 2"=264.53941908713693}, {"Numeric"=339.0169491525424, "Numeric 2"=263.66525423728814}, {"Numeric"=339.30125523012555, "Numeric 2"=262.765690376569}, {"Numeric"=338.9734513274336, "Numeric 2"=262.07964601769913}, {"Numeric"=338.72340425531917, "Numeric 2"=261.4340425531915}, {"Numeric"=338.83700440528634, "Numeric 2"=261.05286343612335}, {"Numeric"=338.7763713080169, "Numeric 2"=260.45147679324896}, {"Numeric"=338.929203539823, "Numeric 2"=260.13274336283183}, {"Numeric"=339.0, "Numeric 2"=260.10480349344977}, {"Numeric"=339.18502202643174, "Numeric 2"=260.07929515418505}, {"Numeric"=339.2703862660944, "Numeric 2"=260.15879828326183}, {"Numeric"=339.2703862660944, "Numeric 2"=260.15879828326183}, {"Numeric"=339.1806167400881, "Numeric 2"=261.0748898678414}, {"Numeric"=339.1181434599156, "Numeric 2"=261.60759493670884}, {"Numeric"=339.1181434599156, "Numeric 2"=261.60759493670884}, {"Numeric"=339.5652173913044, "Numeric 2"=263.1695652173913}, {"Numeric"=339.647577092511, "Numeric 2"=264.1101321585903}, {"Numeric"=340.53846153846155, "Numeric 2"=265.0683760683761}, {"Numeric"=340.34156378600824, "Numeric 2"=265.89300411522635}, {"Numeric"=340.44303797468353, "Numeric 2"=266.9282700421941}, {"Numeric"=340.6348547717842, "Numeric 2"=267.86721991701245}, {"Numeric"=341.3168724279835, "Numeric 2"=268.8847736625514}, {"Numeric"=341.7470355731225, "Numeric 2"=269.6324110671937}, {"Numeric"=341.96385542168673, "Numeric 2"=270.57028112449797}, {"Numeric"=342.1604938271605, "Numeric 2"=271.38271604938274}, {"Numeric"=342.292, "Numeric 2"=271.992}, {"Numeric"=342.4347826086956, "Numeric 2"=272.5375494071146}, {"Numeric"=342.7421875, "Numeric 2"=272.7734375}, {"Numeric"=342.7421875, "Numeric 2"=272.7734375}, {"Numeric"=342.7269076305221, "Numeric 2"=273.49397590361446}, {"Numeric"=342.8366533864542, "Numeric 2"=273.45816733067727}, {"Numeric"=342.60956175298804, "Numeric 2"=273.44621513944224}, {"Numeric"=342.4212598425197, "Numeric 2"=273.12992125984255}, {"Numeric"=342.4745098039216, "Numeric 2"=272.6941176470588}, {"Numeric"=342.21311475409834, "Numeric 2"=272.36475409836066}, {"Numeric"=342.1566265060241, "Numeric 2"=271.6305220883534}, {"Numeric"=341.594262295082, "Numeric 2"=270.922131147541}, {"Numeric"=341.14574898785423, "Numeric 2"=270.42914979757086}, {"Numeric"=341.12598425196853, "Numeric 2"=269.49212598425197}, {"Numeric"=340.70472440944883, "Numeric 2"=268.6692913385827}, {"Numeric"=340.70472440944883, "Numeric 2"=268.6692913385827}, {"Numeric"=339.72244897959183, "Numeric 2"=266.80408163265304}, {"Numeric"=339.3673469387755, "Numeric 2"=265.7551020408163}, {"Numeric"=339.3673469387755, "Numeric 2"=265.7551020408163}, {"Numeric"=338.7763157894737, "Numeric 2"=264.11842105263156}, {"Numeric"=339.03478260869565, "Numeric 2"=263.24347826086955}, {"Numeric"=338.9163179916318, "Numeric 2"=262.56485355648533}, {"Numeric"=338.6666666666667, "Numeric 2"=262.109649122807}, {"Numeric"=338.5378151260504, "Numeric 2"=261.53361344537814}, {"Numeric"=338.6434782608696, "Numeric 2"=261.1565217391304}, {"Numeric"=338.7345132743363, "Numeric 2"=261.01769911504425}, {"Numeric"=338.85833333333335, "Numeric 2"=260.89166666666665}, {"Numeric"=338.7621145374449, "Numeric 2"=260.8810572687225}, {"Numeric"=338.6222222222222, "Numeric 2"=261.08444444444444}, {"Numeric"=338.74122807017545, "Numeric 2"=261.31140350877195}, {"Numeric"=338.6519823788546, "Numeric 2"=261.77973568281936}, {"Numeric"=338.6519823788546, "Numeric 2"=261.77973568281936}, {"Numeric"=339.1911111111111, "Numeric 2"=263.0177777777778}, {"Numeric"=339.24463519313304, "Numeric 2"=263.75536480686696}, {"Numeric"=339.24463519313304, "Numeric 2"=263.75536480686696}, {"Numeric"=339.7991631799163, "Numeric 2"=265.26359832635984}, {"Numeric"=340.33613445378154, "Numeric 2"=266.20168067226894}, {"Numeric"=340.6595744680851, "Numeric 2"=267.13617021276593}, {"Numeric"=341.0403225806452, "Numeric 2"=267.7782258064516}, {"Numeric"=341.369918699187, "Numeric 2"=268.7317073170732}, {"Numeric"=342.0557768924303, "Numeric 2"=269.50597609561754}, {"Numeric"=341.90983606557376, "Numeric 2"=270.344262295082}, {"Numeric"=342.5, "Numeric 2"=270.81496062992125}, {"Numeric"=342.34939759036143, "Numeric 2"=271.5502008032129}, {"Numeric"=342.80392156862746, "Numeric 2"=272.00392156862745}, {"Numeric"=342.84705882352944, "Numeric 2"=272.47843137254904}, {"Numeric"=342.7857142857143, "Numeric 2"=272.6111111111111}, {"Numeric"=342.7857142857143, "Numeric 2"=272.6111111111111}, {"Numeric"=342.8346153846154, "Numeric 2"=272.85769230769233}, {"Numeric"=342.8346153846154, "Numeric 2"=272.85769230769233}, {"Numeric"=342.6235294117647, "Numeric 2"=272.6078431372549}, {"Numeric"=342.24380165289256, "Numeric 2"=272.3512396694215}, {"Numeric"=342.204, "Numeric 2"=271.78}, {"Numeric"=341.90983606557376, "Numeric 2"=271.1844262295082}, {"Numeric"=341.9372549019608, "Numeric 2"=270.5882352941176}, {"Numeric"=341.74285714285713, "Numeric 2"=270.0122448979592}, {"Numeric"=341.10460251046027, "Numeric 2"=269.2384937238494}, {"Numeric"=340.18672199170123, "Numeric 2"=268.28215767634856}, {"Numeric"=340.1551020408163, "Numeric 2"=267.48163265306124}, {"Numeric"=340.0983606557377, "Numeric 2"=266.7745901639344}, {"Numeric"=339.6194331983806, "Numeric 2"=265.64777327935224}, {"Numeric"=339.11538461538464, "Numeric 2"=264.6923076923077}, {"Numeric"=339.11538461538464, "Numeric 2"=264.6923076923077}, {"Numeric"=338.82832618025753, "Numeric 2"=263.656652360515}, {"Numeric"=338.8109243697479, "Numeric 2"=262.6302521008403}, {"Numeric"=338.8109243697479, "Numeric 2"=262.6302521008403}, {"Numeric"=338.90909090909093, "Numeric 2"=262.17316017316017}, {"Numeric"=339.11607142857144, "Numeric 2"=261.9107142857143}, {"Numeric"=337.85897435897436, "Numeric 2"=261.3931623931624}, {"Numeric"=337.85897435897436, "Numeric 2"=261.3931623931624}, {"Numeric"=338.83613445378154, "Numeric 2"=261.70168067226894}, {"Numeric"=338.8914027149321, "Numeric 2"=261.95927601809956}, {"Numeric"=337.991341991342, "Numeric 2"=262.0779220779221}, {"Numeric"=339.11344537815125, "Numeric 2"=262.26050420168065}, {"Numeric"=339.46491228070175, "Numeric 2"=263.030701754386}, {"Numeric"=339.1814345991561, "Numeric 2"=263.55274261603375}, {"Numeric"=338.7136563876652, "Numeric 2"=264.07929515418505}, {"Numeric"=339.43153526970957, "Numeric 2"=264.6970954356847}, {"Numeric"=340.5528455284553, "Numeric 2"=265.520325203252}, {"Numeric"=340.4225941422594, "Numeric 2"=266.38912133891216}, {"Numeric"=340.30212765957447, "Numeric 2"=267.1446808510638}, {"Numeric"=341.64940239043824, "Numeric 2"=267.7250996015936}, {"Numeric"=342.09716599190284, "Numeric 2"=268.63157894736844}, {"Numeric"=341.7336065573771, "Numeric 2"=269.3688524590164}, {"Numeric"=342.4497991967871, "Numeric 2"=269.7670682730924}, {"Numeric"=343.2142857142857, "Numeric 2"=270.531746031746}, {"Numeric"=343.2142857142857, "Numeric 2"=270.531746031746}, {"Numeric"=342.7193675889328, "Numeric 2"=271.50592885375494}, {"Numeric"=343.3897637795276, "Numeric 2"=271.7204724409449}, {"Numeric"=343.9268292682927, "Numeric 2"=272.1747967479675}, {"Numeric"=343.2540322580645, "Numeric 2"=272.3709677419355}, {"Numeric"=342.844, "Numeric 2"=272.296}, {"Numeric"=343.4724409448819, "Numeric 2"=272.13385826771656}, {"Numeric"=343.4724409448819, "Numeric 2"=272.13385826771656}, {"Numeric"=342.9484126984127, "Numeric 2"=271.55555555555554}, {"Numeric"=342.7628458498024, "Numeric 2"=270.9288537549407}, {"Numeric"=342.7628458498024, "Numeric 2"=270.9288537549407}, {"Numeric"=342.4979919678715, "Numeric 2"=270.0281124497992}, {"Numeric"=341.82, "Numeric 2"=269.384}, {"Numeric"=341.69444444444446, "Numeric 2"=268.55555555555554}, {"Numeric"=341.88582677165357, "Numeric 2"=267.6771653543307}, {"Numeric"=340.9710743801653, "Numeric 2"=267.25619834710744}, {"Numeric"=340.56485355648533, "Numeric 2"=266.32217573221754}, {"Numeric"=340.5469387755102, "Numeric 2"=265.43673469387755}, {"Numeric"=340.35, "Numeric 2"=264.90416666666664}, {"Numeric"=339.88702928870293, "Numeric 2"=264.2845188284519}, {"Numeric"=339.38818565400845, "Numeric 2"=263.58649789029533}, {"Numeric"=339.5064935064935, "Numeric 2"=263.16017316017314}, {"Numeric"=339.5064935064935, "Numeric 2"=263.16017316017314}, {"Numeric"=339.3948497854077, "Numeric 2"=262.3175965665236}, {"Numeric"=339.10869565217394, "Numeric 2"=262.10869565217394}, {"Numeric"=339.10869565217394, "Numeric 2"=262.10869565217394}, {"Numeric"=339.1409691629956, "Numeric 2"=262.0616740088106}, {"Numeric"=339.2586206896552, "Numeric 2"=262.14224137931035}, {"Numeric"=339.3608695652174, "Numeric 2"=262.16521739130434}, {"Numeric"=339.3974358974359, "Numeric 2"=262.4273504273504}, {"Numeric"=339.83690987124464, "Numeric 2"=262.7510729613734}, {"Numeric"=339.44635193133047, "Numeric 2"=263.2961373390558}, {"Numeric"=339.5594713656388, "Numeric 2"=263.9162995594714}, {"Numeric"=340.698347107438, "Numeric 2"=264.3801652892562}, {"Numeric"=341.0, "Numeric 2"=265.12068965517244}, {"Numeric"=340.61632653061224, "Numeric 2"=265.6326530612245}, {"Numeric"=340.679012345679, "Numeric 2"=266.46090534979425}, {"Numeric"=340.679012345679, "Numeric 2"=266.46090534979425}, {"Numeric"=341.9510204081633, "Numeric 2"=267.9387755102041}, {"Numeric"=341.79423868312756, "Numeric 2"=268.61728395061726}, {"Numeric"=341.79423868312756, "Numeric 2"=268.61728395061726}, {"Numeric"=342.65714285714284, "Numeric 2"=269.8285714285714}, {"Numeric"=342.7211155378486, "Numeric 2"=270.39043824701196}, {"Numeric"=342.8359375, "Numeric 2"=270.734375}, {"Numeric"=343.116, "Numeric 2"=271.344}, {"Numeric"=343.3807692307692, "Numeric 2"=271.55384615384617}, {"Numeric"=343.08984375, "Numeric 2"=271.65625}, {"Numeric"=343.07003891050584, "Numeric 2"=271.6653696498054}, {"Numeric"=343.0194552529183, "Numeric 2"=271.6692607003891}, {"Numeric"=342.984126984127, "Numeric 2"=271.5595238095238}, {"Numeric"=342.6008064516129, "Numeric 2"=271.40725806451616}, {"Numeric"=342.6008064516129, "Numeric 2"=271.40725806451616}, {"Numeric"=342.65354330708664, "Numeric 2"=270.54330708661416}, {"Numeric"=342.43673469387755, "Numeric 2"=269.9877551020408}, {"Numeric"=342.43673469387755, "Numeric 2"=269.9877551020408}, {"Numeric"=342.0408163265306, "Numeric 2"=268.8326530612245}, {"Numeric"=342.0408163265306, "Numeric 2"=268.8326530612245}, {"Numeric"=341.31020408163266, "Numeric 2"=267.46530612244896}, {"Numeric"=340.797520661157, "Numeric 2"=266.8181818181818}, {"Numeric"=341.0381355932203, "Numeric 2"=266.20338983050846}, {"Numeric"=340.4227642276423, "Numeric 2"=265.4674796747967}, {"Numeric"=340.40416666666664, "Numeric 2"=264.8833333333333}, {"Numeric"=339.836820083682, "Numeric 2"=264.34728033472805}, {"Numeric"=339.79295154185024, "Numeric 2"=263.8458149779736}, {"Numeric"=340.34599156118145, "Numeric 2"=263.2742616033755}, {"Numeric"=339.59656652360513, "Numeric 2"=262.79828326180257}, {"Numeric"=339.9917355371901, "Numeric 2"=262.44628099173553}, {"Numeric"=340.30801687763716, "Numeric 2"=262.30801687763716}, {"Numeric"=340.30801687763716, "Numeric 2"=262.30801687763716}, {"Numeric"=339.97446808510637, "Numeric 2"=262.22978723404253}, {"Numeric"=340.21940928270044, "Numeric 2"=262.28270042194094}, {"Numeric"=340.21940928270044, "Numeric 2"=262.28270042194094}, {"Numeric"=339.987012987013, "Numeric 2"=262.8225108225108}, {"Numeric"=340.364406779661, "Numeric 2"=263.22457627118644}, {"Numeric"=340.2139737991266, "Numeric 2"=263.7903930131004}, {"Numeric"=340.73221757322176, "Numeric 2"=264.2928870292887}, {"Numeric"=340.5, "Numeric 2"=265.0394736842105}, {"Numeric"=340.7489711934156, "Numeric 2"=265.3991769547325}, {"Numeric"=340.65800865800867, "Numeric 2"=266.2164502164502}, {"Numeric"=341.1398305084746, "Numeric 2"=266.8262711864407}, {"Numeric"=341.43673469387755, "Numeric 2"=267.4530612244898}, {"Numeric"=341.41224489795917, "Numeric 2"=268.3265306122449}, {"Numeric"=341.7551867219917, "Numeric 2"=268.8215767634855}, {"Numeric"=342.0242914979757, "Numeric 2"=269.4089068825911}, {"Numeric"=342.0242914979757, "Numeric 2"=269.4089068825911}, {"Numeric"=342.10887096774195, "Numeric 2"=270.383064516129}, {"Numeric"=342.10887096774195, "Numeric 2"=270.383064516129}, {"Numeric"=342.8804780876494, "Numeric 2"=271.0478087649402}, {"Numeric"=342.8857142857143, "Numeric 2"=271.2326530612245}, {"Numeric"=342.64426877470356, "Numeric 2"=271.4387351778656}, {"Numeric"=342.66932270916334, "Numeric 2"=271.48605577689244}, {"Numeric"=342.864, "Numeric 2"=271.404}, {"Numeric"=342.6324110671937, "Numeric 2"=271.2332015810277}, {"Numeric"=342.59362549800795, "Numeric 2"=270.7848605577689}, {"Numeric"=342.31075697211156, "Numeric 2"=270.53386454183266}, {"Numeric"=342.31075697211156, "Numeric 2"=270.53386454183266}, {"Numeric"=342.1475409836066, "Numeric 2"=270.28688524590166}, {"Numeric"=341.991935483871, "Numeric 2"=269.5967741935484}, {"Numeric"=342.0123966942149, "Numeric 2"=269.22314049586777}, {"Numeric"=341.91269841269843, "Numeric 2"=268.6468253968254}, {"Numeric"=341.91269841269843, "Numeric 2"=268.6468253968254}, {"Numeric"=340.9504132231405, "Numeric 2"=267.3429752066116}, {"Numeric"=340.8137651821862, "Numeric 2"=266.5910931174089}, {"Numeric"=340.8137651821862, "Numeric 2"=266.5910931174089}, {"Numeric"=340.86345381526104, "Numeric 2"=265.3574297188755}, {"Numeric"=340.559670781893, "Numeric 2"=264.7695473251029}, {"Numeric"=340.55982905982904, "Numeric 2"=264.1923076923077}, {"Numeric"=340.1794871794872, "Numeric 2"=263.7991452991453}, {"Numeric"=340.23809523809524, "Numeric 2"=263.23376623376623}, {"Numeric"=340.3491379310345, "Numeric 2"=262.91379310344826}, {"Numeric"=340.0464135021097, "Numeric 2"=262.6455696202532}, {"Numeric"=339.8242677824268, "Numeric 2"=262.5732217573222}, {"Numeric"=340.156378600823, "Numeric 2"=262.4691358024691}, {"Numeric"=340.1410788381743, "Numeric 2"=262.49792531120335}, {"Numeric"=340.0775510204082, "Numeric 2"=262.6204081632653}, {"Numeric"=340.17391304347825, "Numeric 2"=263.0}, {"Numeric"=340.17391304347825, "Numeric 2"=263.0}, {"Numeric"=340.3813559322034, "Numeric 2"=263.6228813559322}, {"Numeric"=340.5215517241379, "Numeric 2"=264.1336206896552}, {"Numeric"=340.4375, "Numeric 2"=264.5083333333333}, {"Numeric"=340.5807860262009, "Numeric 2"=265.117903930131}, {"Numeric"=340.67330677290835, "Numeric 2"=265.66932270916334}, {"Numeric"=340.7615062761506, "Numeric 2"=266.40585774058576}, {"Numeric"=341.2931034482759, "Numeric 2"=267.08620689655174}, {"Numeric"=341.43775100401604, "Numeric 2"=267.61044176706827}, {"Numeric"=341.36213991769546, "Numeric 2"=268.3333333333333}, {"Numeric"=341.8204081632653, "Numeric 2"=268.8530612244898}, {"Numeric"=341.72469635627533, "Numeric 2"=269.3724696356275}, {"Numeric"=342.4859437751004, "Numeric 2"=269.718875502008}, {"Numeric"=341.9756097560976, "Numeric 2"=270.3780487804878}, {"Numeric"=341.9756097560976, "Numeric 2"=270.3780487804878}, {"Numeric"=342.65098039215684, "Numeric 2"=270.7843137254902}, {"Numeric"=342.65098039215684, "Numeric 2"=270.7843137254902}, {"Numeric"=342.3467741935484, "Numeric 2"=271.39516129032256}, {"Numeric"=342.43621399176953, "Numeric 2"=271.30452674897117}, {"Numeric"=342.2217741935484, "Numeric 2"=271.1774193548387}, {"Numeric"=342.6023622047244, "Numeric 2"=270.88188976377955}, {"Numeric"=342.546875, "Numeric 2"=270.62109375}, {"Numeric"=342.546875, "Numeric 2"=270.62109375}, {"Numeric"=342.21311475409834, "Numeric 2"=269.905737704918}, {"Numeric"=342.2008032128514, "Numeric 2"=269.4899598393574}, {"Numeric"=342.2572614107884, "Numeric 2"=269.00829875518673}, {"Numeric"=341.9681274900398, "Numeric 2"=268.46613545816734}, {"Numeric"=341.7193675889328, "Numeric 2"=267.69565217391306}, {"Numeric"=341.4586776859504, "Numeric 2"=267.2685950413223}, {"Numeric"=341.5487804878049, "Numeric 2"=266.479674796748}, {"Numeric"=341.268, "Numeric 2"=265.844}, {"Numeric"=341.268, "Numeric 2"=265.844}, {"Numeric"=341.02834008097165, "Numeric 2"=264.69635627530363}, {"Numeric"=340.8143459915612, "Numeric 2"=264.21940928270044}, {"Numeric"=340.6523605150215, "Numeric 2"=263.75536480686696}, {"Numeric"=341.0163934426229, "Numeric 2"=263.3524590163934}, {"Numeric"=340.73799126637556, "Numeric 2"=263.08733624454146}, {"Numeric"=340.1694915254237, "Numeric 2"=262.78389830508473}, {"Numeric"=340.2025316455696, "Numeric 2"=262.6413502109705}, {"Numeric"=340.36213991769546, "Numeric 2"=262.57201646090533}, {"Numeric"=340.55510204081634, "Numeric 2"=262.59183673469386}, {"Numeric"=340.55230125523013, "Numeric 2"=262.78242677824267}, {"Numeric"=340.24675324675326, "Numeric 2"=263.14285714285717}, {"Numeric"=340.54468085106384, "Numeric 2"=263.2808510638298}, {"Numeric"=340.54468085106384, "Numeric 2"=263.2808510638298}, {"Numeric"=340.3776824034335, "Numeric 2"=264.14163090128756}, {"Numeric"=340.3776824034335, "Numeric 2"=264.14163090128756}, {"Numeric"=340.80252100840335, "Numeric 2"=265.1890756302521}, {"Numeric"=340.80252100840335, "Numeric 2"=265.1890756302521}, {"Numeric"=340.53688524590166, "Numeric 2"=266.4303278688525}, {"Numeric"=340.89495798319325, "Numeric 2"=267.109243697479}, {"Numeric"=340.90725806451616, "Numeric 2"=267.53225806451616}, {"Numeric"=340.9387755102041, "Numeric 2"=268.38367346938776}, {"Numeric"=341.25099601593627, "Numeric 2"=268.8486055776892}, {"Numeric"=341.48192771084337, "Numeric 2"=269.3815261044177}, {"Numeric"=342.0436507936508, "Numeric 2"=269.6825396825397}, {"Numeric"=341.9362549800797, "Numeric 2"=270.33466135458167}, {"Numeric"=341.90551181102364, "Numeric 2"=270.50787401574803}, {"Numeric"=342.4824902723735, "Numeric 2"=270.67315175097275}, {"Numeric"=342.16, "Numeric 2"=270.936}, {"Numeric"=342.55335968379444, "Numeric 2"=270.9683794466403}, {"Numeric"=342.55335968379444, "Numeric 2"=270.9683794466403}, {"Numeric"=342.6521739130435, "Numeric 2"=270.8893280632411}, {"Numeric"=342.6521739130435, "Numeric 2"=270.8893280632411}, {"Numeric"=342.5546875, "Numeric 2"=270.55859375}, {"Numeric"=342.4331983805668, "Numeric 2"=270.3157894736842}, {"Numeric"=342.76209677419354, "Numeric 2"=269.7983870967742}, {"Numeric"=342.085020242915, "Numeric 2"=269.32793522267207}, {"Numeric"=342.10843373493975, "Numeric 2"=268.7550200803213}, {"Numeric"=342.316, "Numeric 2"=268.496}, {"Numeric"=342.28629032258067, "Numeric 2"=267.90725806451616}, {"Numeric"=341.6694214876033, "Numeric 2"=267.0330578512397}, {"Numeric"=341.0, "Numeric 2"=266.22033898305085}, {"Numeric"=341.5101214574899, "Numeric 2"=265.914979757085}, {"Numeric"=342.4008097165992, "Numeric 2"=265.39676113360326}, {"Numeric"=341.22131147540983, "Numeric 2"=264.6803278688525}, {"Numeric"=340.7617021276596, "Numeric 2"=264.18297872340423}, {"Numeric"=340.7617021276596, "Numeric 2"=264.18297872340423}, {"Numeric"=341.390756302521, "Numeric 2"=263.4621848739496}, {"Numeric"=340.3491379310345, "Numeric 2"=263.08620689655174}, {"Numeric"=340.1386554621849, "Numeric 2"=262.8487394957983}, {"Numeric"=341.1101694915254, "Numeric 2"=262.9364406779661}, {"Numeric"=340.9710743801653, "Numeric 2"=262.8099173553719}, {"Numeric"=339.49159663865544, "Numeric 2"=262.62605042016804}, {"Numeric"=339.5042016806723, "Numeric 2"=262.827731092437}, {"Numeric"=340.2173913043478, "Numeric 2"=263.11739130434785}, {"Numeric"=339.6455696202532, "Numeric 2"=263.44725738396625}, {"Numeric"=338.99555555555554, "Numeric 2"=264.0}, {"Numeric"=339.8728813559322, "Numeric 2"=264.25}, {"Numeric"=340.1124497991968, "Numeric 2"=264.6425702811245}, {"Numeric"=339.15677966101697, "Numeric 2"=265.20338983050846}, {"Numeric"=339.15677966101697, "Numeric 2"=265.20338983050846}, {"Numeric"=340.1422764227642, "Numeric 2"=266.4024390243902}, {"Numeric"=340.38396624472574, "Numeric 2"=267.2320675105485}, {"Numeric"=339.8809523809524, "Numeric 2"=267.531746031746}, {"Numeric"=339.61087866108784, "Numeric 2"=268.2050209205021}, {"Numeric"=340.56972111553785, "Numeric 2"=268.75298804780874}, {"Numeric"=340.7654320987654, "Numeric 2"=269.36625514403295}, {"Numeric"=340.7470355731225, "Numeric 2"=269.6837944664032}, {"Numeric"=341.07287449392715, "Numeric 2"=270.31174089068827}, {"Numeric"=341.45, "Numeric 2"=270.65384615384613}, {"Numeric"=341.16279069767444, "Numeric 2"=270.68992248062017}, {"Numeric"=341.35849056603774, "Numeric 2"=270.76981132075474}, {"Numeric"=341.82213438735175, "Numeric 2"=270.99209486166006}, {"Numeric"=342.0282258064516, "Numeric 2"=271.31048387096774}, {"Numeric"=342.06477732793525, "Numeric 2"=271.2914979757085}, {"Numeric"=341.9571984435798, "Numeric 2"=270.7003891050584}, {"Numeric"=341.9571984435798, "Numeric 2"=270.7003891050584}, {"Numeric"=342.0443548387097, "Numeric 2"=270.383064516129}, {"Numeric"=341.94262295081967, "Numeric 2"=269.8196721311475}, {"Numeric"=342.140562248996, "Numeric 2"=269.48192771084337}, {"Numeric"=342.11914893617023, "Numeric 2"=269.15744680851066}, {"Numeric"=342.01612903225805, "Numeric 2"=268.55645161290323}, {"Numeric"=341.34387351778656, "Numeric 2"=267.7707509881423}, {"Numeric"=341.2857142857143, "Numeric 2"=267.33061224489796}, {"Numeric"=341.9186991869919, "Numeric 2"=266.739837398374}, {"Numeric"=341.35833333333335, "Numeric 2"=266.3125}, {"Numeric"=341.0517928286853, "Numeric 2"=265.54980079681275}, {"Numeric"=341.31120331950206, "Numeric 2"=265.20746887966806}, {"Numeric"=341.1260162601626, "Numeric 2"=264.6178861788618}, {"Numeric"=340.96638655462186, "Numeric 2"=264.1806722689076}, {"Numeric"=340.96638655462186, "Numeric 2"=264.1806722689076}, {"Numeric"=340.6144578313253, "Numeric 2"=263.6144578313253}, {"Numeric"=340.6144578313253, "Numeric 2"=263.6144578313253}, {"Numeric"=340.0300429184549, "Numeric 2"=263.20600858369096}, {"Numeric"=339.38260869565215, "Numeric 2"=263.11304347826086}, {"Numeric"=339.6794871794872, "Numeric 2"=263.15811965811963}, {"Numeric"=339.9113924050633, "Numeric 2"=263.28691983122366}, {"Numeric"=339.36401673640165, "Numeric 2"=263.4560669456067}, {"Numeric"=339.3648068669528, "Numeric 2"=263.7639484978541}, {"Numeric"=339.3434782608696, "Numeric 2"=264.1565217391304}, {"Numeric"=339.69456066945605, "Numeric 2"=264.35983263598325}, {"Numeric"=339.28691983122366, "Numeric 2"=264.8270042194093}, {"Numeric"=339.2459677419355, "Numeric 2"=265.3991935483871}, {"Numeric"=339.55510204081634, "Numeric 2"=265.9428571428571}, {"Numeric"=339.7967479674797, "Numeric 2"=266.630081300813}, {"Numeric"=339.4, "Numeric 2"=267.1531914893617}, {"Numeric"=339.4, "Numeric 2"=267.1531914893617}, {"Numeric"=340.14344262295083, "Numeric 2"=268.30737704918033}, {"Numeric"=340.14344262295083, "Numeric 2"=268.30737704918033}, {"Numeric"=340.10330578512395, "Numeric 2"=269.301652892562}, {"Numeric"=340.8339920948617, "Numeric 2"=269.6482213438735}, {"Numeric"=341.0080971659919, "Numeric 2"=270.2591093117409}, {"Numeric"=340.7890625, "Numeric 2"=270.421875}, {"Numeric"=340.7015503875969, "Numeric 2"=270.55426356589146}, {"Numeric"=341.4, "Numeric 2"=270.7372549019608}, {"Numeric"=341.6640316205534, "Numeric 2"=270.8656126482214}, {"Numeric"=341.5595238095238, "Numeric 2"=270.8809523809524}, {"Numeric"=341.7290076335878, "Numeric 2"=270.73664122137404}, {"Numeric"=341.99609375, "Numeric 2"=270.625}, {"Numeric"=341.60557768924303, "Numeric 2"=270.43824701195217}, {"Numeric"=341.59274193548384, "Numeric 2"=270.3306451612903}, {"Numeric"=342.0281124497992, "Numeric 2"=269.7670682730924}, {"Numeric"=342.0281124497992, "Numeric 2"=269.7670682730924}, {"Numeric"=341.4979079497908, "Numeric 2"=269.1255230125523}, {"Numeric"=341.12048192771084, "Numeric 2"=268.44176706827307}, {"Numeric"=341.32530120481925, "Numeric 2"=267.82730923694777}, {"Numeric"=341.4763779527559, "Numeric 2"=267.4409448818898}, {"Numeric"=341.2113821138211, "Numeric 2"=266.9593495934959}, {"Numeric"=341.2113821138211, "Numeric 2"=266.9593495934959}, {"Numeric"=340.7609561752988, "Numeric 2"=265.62948207171314}, {"Numeric"=340.761316872428, "Numeric 2"=265.2510288065844}, {"Numeric"=340.5528455284553, "Numeric 2"=264.6382113821138}, {"Numeric"=340.7457627118644, "Numeric 2"=264.1991525423729}, {"Numeric"=340.46153846153845, "Numeric 2"=264.0854700854701}, {"Numeric"=340.43933054393307, "Numeric 2"=263.7531380753138}, {"Numeric"=339.93305439330544, "Numeric 2"=263.418410041841}, {"Numeric"=340.0331950207469, "Numeric 2"=263.27385892116183}, {"Numeric"=339.9670781893004, "Numeric 2"=263.3333333333333}, {"Numeric"=339.7296137339056, "Numeric 2"=264.0214592274678}, {"Numeric"=339.68220338983053, "Numeric 2"=265.0762711864407}, {"Numeric"=339.8835341365462, "Numeric 2"=266.49397590361446}, {"Numeric"=340.74583333333334, "Numeric 2"=268.24583333333334}, {"Numeric"=341.25581395348837, "Numeric 2"=269.8255813953488}, {"Numeric"=341.6640625, "Numeric 2"=270.6328125}, {"Numeric"=341.3413654618474, "Numeric 2"=267.8072289156627}, {"Numeric"=340.52542372881356, "Numeric 2"=264.1525423728813}, {"Numeric"=340.12295081967216, "Numeric 2"=263.75409836065575}, {"Numeric"=341.1607843137255, "Numeric 2"=267.5372549019608}, {"Numeric"=341.77510040160644, "Numeric 2"=270.4096385542169}, {"Numeric"=341.7560975609756, "Numeric 2"=269.2845528455285}, {"Numeric"=340.796875, "Numeric 2"=265.765625}, {"Numeric"=340.655601659751, "Numeric 2"=263.5560165975104}, {"Numeric"=340.92712550607285, "Numeric 2"=265.4412955465587}, {"Numeric"=342.255905511811, "Numeric 2"=269.5}, {"Numeric"=341.78823529411767, "Numeric 2"=269.8627450980392}, {"Numeric"=340.559670781893, "Numeric 2"=266.8230452674897}, {"Numeric"=340.62978723404257, "Numeric 2"=264.11914893617023}, {"Numeric"=340.8833333333333, "Numeric 2"=264.7875}, {"Numeric"=341.64166666666665, "Numeric 2"=268.23333333333335}, {"Numeric"=341.68595041322317, "Numeric 2"=270.1404958677686}, {"Numeric"=341.05737704918033, "Numeric 2"=268.2295081967213}, {"Numeric"=340.82278481012656, "Numeric 2"=265.084388185654}, {"Numeric"=341.4599156118143, "Numeric 2"=264.2025316455696}, {"Numeric"=341.2764227642276, "Numeric 2"=266.3780487804878}, {"Numeric"=341.5136186770428, "Numeric 2"=269.52140077821014}, {"Numeric"=340.9596774193548, "Numeric 2"=269.4153225806452}, {"Numeric"=340.4181034482759, "Numeric 2"=266.23275862068965}, {"Numeric"=340.9237288135593, "Numeric 2"=264.21610169491527}, {"Numeric"=341.336, "Numeric 2"=265.568}, {"Numeric"=340.99196787148594, "Numeric 2"=268.65060240963857}, {"Numeric"=341.49612403100775, "Numeric 2"=269.52713178294573}, {"Numeric"=340.59055118110234, "Numeric 2"=267.7716535433071}, {"Numeric"=340.7731092436975, "Numeric 2"=264.92857142857144}, {"Numeric"=341.25, "Numeric 2"=264.72131147540983}, {"Numeric"=341.428, "Numeric 2"=267.428}, {"Numeric"=341.2510288065844, "Numeric 2"=269.3292181069959}, {"Numeric"=341.077868852459, "Numeric 2"=268.45081967213116}, {"Numeric"=341.0590717299578, "Numeric 2"=266.17721518987344}, {"Numeric"=340.5514403292181, "Numeric 2"=264.7448559670782}, {"Numeric"=340.780487804878, "Numeric 2"=266.4308943089431}, {"Numeric"=341.828, "Numeric 2"=268.808}, {"Numeric"=342.18039215686275, "Numeric 2"=269.61960784313726}, {"Numeric"=342.5263157894737, "Numeric 2"=269.4331983805668}, {"Numeric"=339.4475806451613, "Numeric 2"=263.76209677419354}, {"Numeric"=340.01702127659576, "Numeric 2"=259.0468085106383}]
  out "XY Graph":cluster{"X":dbl, "Y":dbl}[](graph)=[{"X"=0.0, "Y"=343.3711790393013}, {"X"=0.008333333333333333, "Y"=337.0897435897436}, {"X"=0.016666666666666666, "Y"=335.8137651821862}, {"X"=0.025, "Y"=343.1166666666667}, {"X"=0.03333333333333333, "Y"=348.0122448979592}, {"X"=0.041666666666666664, "Y"=344.37130801687766}, {"X"=0.05, "Y"=338.55274261603375}, {"X"=0.058333333333333334, "Y"=337.68879668049794}, {"X"=0.06666666666666667, "Y"=340.15744680851066}, {"X"=0.075, "Y"=345.2207792207792}, {"X"=0.08333333333333333, "Y"=343.76190476190476}, {"X"=0.09166666666666666, "Y"=340.12345679012344}, {"X"=0.1, "Y"=340.2276422764228}, {"X"=0.10833333333333334, "Y"=341.6163793103448}, {"X"=0.11666666666666667, "Y"=341.60084033613447}, {"X"=0.125, "Y"=340.8185654008439}, {"X"=0.13333333333333333, "Y"=340.336170212766}, {"X"=0.14166666666666666, "Y"=341.6900826446281}, {"X"=0.15, "Y"=342.0576131687243}, {"X"=0.15833333333333333, "Y"=340.67932489451476}, {"X"=0.16666666666666666, "Y"=339.1673640167364}, {"X"=0.175, "Y"=339.72294372294374}, {"X"=0.18333333333333332, "Y"=341.9240506329114}, {"X"=0.19166666666666668, "Y"=343.8050847457627}, {"X"=0.2, "Y"=342.1652892561983}, {"X"=0.20833333333333334, "Y"=338.8601694915254}, {"X"=0.21666666666666667, "Y"=338.6923076923077}, {"X"=0.225, "Y"=343.2983870967742}, {"X"=0.23333333333333334, "Y"=345.4567901234568}, {"X"=0.24166666666666667, "Y"=343.94142259414224}, {"X"=0.25, "Y"=338.93004115226336}, {"X"=0.25833333333333336, "Y"=337.390243902439}, {"X"=0.26666666666666666, "Y"=340.9665271966527}, {"X"=0.275, "Y"=345.13675213675214}, {"X"=0.2833333333333333, "Y"=346.1016260162602}, {"X"=0.2916666666666667, "Y"=345.79918032786884}, {"X"=0.3, "Y"=342.5042016806723}, {"X"=0.30833333333333335, "Y"=340.68595041322317}, {"X"=0.31666666666666665, "Y"=339.0365853658537}, {"X"=0.325, "Y"=338.1623931623932}, {"X"=0.3333333333333333, "Y"=338.4458333333333}, {"X"=0.3416666666666667, "Y"=338.8691983122363}, {"X"=0.35, "Y"=339.4268292682927}, {"X"=0.35833333333333334, "Y"=340.4530612244898}, {"X"=0.36666666666666664, "Y"=341.6302521008403}, {"X"=0.375, "Y"=342.9958158995816}, {"X"=0.38333333333333336, "Y"=342.9958158995816}, {"X"=0.39166666666666666, "Y"=344.2236286919831}, {"X"=0.4, "Y"=344.7909836065574}, {"X"=0.4083333333333333, "Y"=345.0468085106383}, {"X"=0.4166666666666667, "Y"=345.1603375527426}, {"X"=0.425, "Y"=345.48319327731093}, {"X"=0.43333333333333335, "Y"=345.68200836820085}, {"X"=0.44166666666666665, "Y"=345.50416666666666}, {"X"=0.45, "Y"=345.43388429752065}, {"X"=0.4583333333333333, "Y"=345.2307692307692}, {"X"=0.4666666666666667, "Y"=344.9428571428571}, {"X"=0.475, "Y"=344.5420168067227}, {"X"=0.48333333333333334, "Y"=344.4579831932773}, {"X"=0.49166666666666664, "Y"=344.26808510638296}, {"X"=0.5, "Y"=343.61965811965814}, {"X"=0.5083333333333333, "Y"=343.0420168067227}, {"X"=0.5166666666666667, "Y"=342.40677966101697}, {"X"=0.525, "Y"=342.1991701244813}, {"X"=0.5333333333333333, "Y"=341.6846473029046}, {"X"=0.5416666666666666, "Y"=341.12133891213387}, {"X"=0.55, "Y"=340.73390557939916}, {"X"=0.5583333333333333, "Y"=339.8933333333333}, {"X"=0.5666666666666667, "Y"=339.8933333333333}, {"X"=0.575, "Y"=339.60084033613447}, {"X"=0.5833333333333334, "Y"=339.5611814345992}, {"X"=0.5916666666666667, "Y"=339.508064516129}, {"X"=0.6, "Y"=339.4475806451613}, {"X"=0.6083333333333333, "Y"=339.4475806451613}, {"X"=0.6166666666666667, "Y"=339.16806722689074}, {"X"=0.625, "Y"=339.3703703703704}, {"X"=0.6333333333333333, "Y"=339.45147679324896}, {"X"=0.6416666666666667, "Y"=339.63713080168776}, {"X"=0.65, "Y"=340.12133891213387}, {"X"=0.6583333333333333, "Y"=339.9324894514768}, {"X"=0.6666666666666666, "Y"=340.11297071129707}, {"X"=0.675, "Y"=341.198347107438}, {"X"=0.6833333333333333, "Y"=341.6170212765957}, {"X"=0.6916666666666667, "Y"=342.01659751037346}, {"X"=0.7, "Y"=342.0082304526749}, {"X"=0.7083333333333334, "Y"=342.5162601626016}, {"X"=0.7166666666666667, "Y"=342.5162601626016}, {"X"=0.725, "Y"=342.8512396694215}, {"X"=0.7333333333333333, "Y"=342.8512396694215}, {"X"=0.7416666666666667, "Y"=343.22222222222223}, {"X"=0.75, "Y"=343.10526315789474}, {"X"=0.7583333333333333, "Y"=343.0295358649789}, {"X"=0.7666666666666667, "Y"=343.5163934426229}, {"X"=0.775, "Y"=343.64406779661016}, {"X"=0.7833333333333333, "Y"=343.6846473029046}, {"X"=0.7916666666666666, "Y"=343.40677966101697}, {"X"=0.8, "Y"=343.51724137931035}, {"X"=0.8083333333333333, "Y"=343.2436974789916}, {"X"=0.8166666666666667, "Y"=343.23770491803276}, {"X"=0.825, "Y"=343.0082304526749}, {"X"=0.8333333333333334, "Y"=342.83613445378154}, {"X"=0.8416666666666667, "Y"=342.38429752066116}, {"X"=0.85, "Y"=342.38429752066116}, {"X"=0.8583333333333333, "Y"=341.76050420168065}, {"X"=0.8666666666666667, "Y"=341.9}, {"X"=0.875, "Y"=341.6848739495798}, {"X"=0.8833333333333333, "Y"=341.0219298245614}, {"X"=0.8916666666666667, "Y"=340.9957081545064}, {"X"=0.9, "Y"=340.6864406779661}, {"X"=0.9083333333333333, "Y"=340.2340425531915}, {"X"=0.9166666666666666, "Y"=340.4978902953587}, {"X"=0.925, "Y"=340.24050632911394}, {"X"=0.9333333333333333, "Y"=340.54741379310343}, {"X"=0.9416666666666667, "Y"=340.53711790393015}, {"X"=0.95, "Y"=340.49568965517244}, {"X"=0.9583333333333334, "Y"=340.49568965517244}, {"X"=0.9666666666666667, "Y"=340.61728395061726}, {"X"=0.975, "Y"=340.5983606557377}, {"X"=0.9833333333333333, "Y"=340.5983606557377}, {"X"=0.9916666666666667, "Y"=341.33613445378154}, {"X"=1.0, "Y"=341.44166666666666}, {"X"=1.0083333333333333, "Y"=341.6652719665272}, {"X"=1.0166666666666666, "Y"=341.6313559322034}, {"X"=1.025, "Y"=341.77292576419217}, {"X"=1.0333333333333334, "Y"=341.965367965368}, {"X"=1.0416666666666667, "Y"=341.93886462882097}, {"X"=1.05, "Y"=342.1025641025641}, {"X"=1.0583333333333333, "Y"=342.3151260504202}, {"X"=1.0666666666666667, "Y"=342.0258620689655}, {"X"=1.075, "Y"=342.3801652892562}, {"X"=1.0833333333333333, "Y"=342.3801652892562}, {"X"=1.0916666666666666, "Y"=342.2716049382716}, {"X"=1.1, "Y"=342.4074074074074}, {"X"=1.1083333333333334, "Y"=342.4074074074074}, {"X"=1.1166666666666667, "Y"=342.10775862068965}, {"X"=1.125, "Y"=342.2920353982301}, {"X"=1.1333333333333333, "Y"=342.2324561403509}, {"X"=1.1416666666666666, "Y"=342.14285714285717}, {"X"=1.15, "Y"=341.89121338912133}, {"X"=1.1583333333333334, "Y"=341.864406779661}, {"X"=1.1666666666666667, "Y"=341.75536480686696}, {"X"=1.175, "Y"=341.8663793103448}, {"X"=1.1833333333333333, "Y"=341.6523605150215}, {"X"=1.1916666666666667, "Y"=341.1965065502183}, {"X"=1.2, "Y"=341.24896265560164}, {"X"=1.2083333333333333, "Y"=341.24896265560164}, {"X"=1.2166666666666666, "Y"=341.16170212765957}, {"X"=1.225, "Y"=341.1673640167364}, {"X"=1.2333333333333334, "Y"=341.1673640167364}, {"X"=1.2416666666666667, "Y"=341.29957805907173}, {"X"=1.25, "Y"=341.46610169491527}, {"X"=1.2583333333333333, "Y"=341.4051724137931}, {"X"=1.2666666666666666, "Y"=341.3974358974359}, {"X"=1.275, "Y"=341.50847457627117}, {"X"=1.2833333333333334, "Y"=341.50622406639}, {"X"=1.2916666666666667, "Y"=341.4813278008299}, {"X"=1.3, "Y"=341.7375}, {"X"=1.3083333333333333, "Y"=341.7543859649123}, {"X"=1.3166666666666667, "Y"=341.93886462882097}, {"X"=1.325, "Y"=342.10743801652893}, {"X"=1.3333333333333333, "Y"=342.22314049586777}, {"X"=1.3416666666666666, "Y"=342.27755102040817}, {"X"=1.35, "Y"=342.27755102040817}, {"X"=1.3583333333333334, "Y"=342.30204081632655}, {"X"=1.3666666666666667, "Y"=342.15833333333336}, {"X"=1.375, "Y"=342.15833333333336}, {"X"=1.3833333333333333, "Y"=342.2382978723404}, {"X"=1.3916666666666666, "Y"=342.0625}, {"X"=1.4, "Y"=342.1125}, {"X"=1.4083333333333334, "Y"=341.9353448275862}, {"X"=1.4166666666666667, "Y"=341.9353448275862}, {"X"=1.425, "Y"=341.78508771929825}, {"X"=1.4333333333333333, "Y"=341.9446808510638}, {"X"=1.4416666666666667, "Y"=341.5762711864407}, {"X"=1.45, "Y"=341.422131147541}, {"X"=1.4583333333333333, "Y"=341.1885245901639}, {"X"=1.4666666666666666, "Y"=341.3927125506073}, {"X"=1.475, "Y"=341.4186991869919}, {"X"=1.4833333333333334, "Y"=341.07053941908714}, {"X"=1.4916666666666667, "Y"=341.07053941908714}, {"X"=1.5, "Y"=340.7467248908297}, {"X"=1.5083333333333333, "Y"=340.48908296943233}, {"X"=1.5166666666666666, "Y"=340.85}, {"X"=1.525, "Y"=340.98333333333335}, {"X"=1.5333333333333334, "Y"=340.8559670781893}, {"X"=1.5416666666666667, "Y"=340.74789915966386}, {"X"=1.55, "Y"=341.390756302521}, {"X"=1.5583333333333333, "Y"=341.46351931330474}, {"X"=1.5666666666666667, "Y"=341.7038626609442}, {"X"=1.575, "Y"=341.868085106383}, {"X"=1.5833333333333333, "Y"=341.9008620689655}, {"X"=1.5916666666666666, "Y"=342.0882352941176}, {"X"=1.6, "Y"=342.1589958158996}, {"X"=1.6083333333333334, "Y"=342.1589958158996}, {"X"=1.6166666666666667, "Y"=342.4848484848485}, {"X"=1.625, "Y"=342.4848484848485}, {"X"=1.6333333333333333, "Y"=342.5875}, {"X"=1.6416666666666666, "Y"=342.9016393442623}, {"X"=1.65, "Y"=343.172131147541}, {"X"=1.6583333333333334, "Y"=343.17083333333335}, {"X"=1.6666666666666667, "Y"=343.0548523206751}, {"X"=1.675, "Y"=343.0940170940171}, {"X"=1.6833333333333333, "Y"=343.3404255319149}, {"X"=1.6916666666666667, "Y"=343.15384615384613}, {"X"=1.7, "Y"=342.6666666666667}, {"X"=1.7083333333333333, "Y"=342.5708333333333}, {"X"=1.7166666666666666, "Y"=342.6138211382114}, {"X"=1.725, "Y"=342.4669421487603}, {"X"=1.7333333333333334, "Y"=342.16326530612247}, {"X"=1.7416666666666667, "Y"=342.16326530612247}, {"X"=1.75, "Y"=341.7570850202429}, {"X"=1.7583333333333333, "Y"=341.4552845528455}, {"X"=1.7666666666666666, "Y"=341.0532786885246}, {"X"=1.775, "Y"=340.8481012658228}, {"X"=1.7833333333333334, "Y"=340.9504132231405}, {"X"=1.7916666666666667, "Y"=340.28979591836736}, {"X"=1.8, "Y"=339.8125}, {"X"=1.8083333333333333, "Y"=339.9311740890688}, {"X"=1.8166666666666667, "Y"=339.796812749004}, {"X"=1.825, "Y"=339.84313725490193}, {"X"=1.8333333333333333, "Y"=339.758064516129}, {"X"=1.8416666666666666, "Y"=339.77016129032256}, {"X"=1.85, "Y"=339.38683127572017}, {"X"=1.8583333333333334, "Y"=339.6502057613169}, {"X"=1.8666666666666667, "Y"=339.6502057613169}, {"X"=1.875, "Y"=340.1991341991342}, {"X"=1.8833333333333333, "Y"=340.0901287553648}, {"X"=1.8916666666666666, "Y"=340.3029045643153}, {"X"=1.9, "Y"=340.7745901639344}, {"X"=1.9083333333333334, "Y"=341.4}, {"X"=1.9166666666666667, "Y"=341.74380165289256}, {"X"=1.925, "Y"=342.14112903225805}, {"X"=1.9333333333333333, "Y"=342.3469387755102}, {"X"=1.9416666666666667, "Y"=342.68879668049794}, {"X"=1.95, "Y"=342.87916666666666}, {"X"=1.9583333333333333, "Y"=343.3375}, {"X"=1.9666666666666666, "Y"=343.8284518828452}, {"X"=1.975, "Y"=344.1518987341772}, {"X"=1.9833333333333334, "Y"=344.1518987341772}, {"X"=1.9916666666666667, "Y"=344.37759336099583}, {"X"=2.0, "Y"=344.2716049382716}, {"X"=2.0083333333333333, "Y"=344.2716049382716}, {"X"=2.0166666666666666, "Y"=344.3374485596708}, {"X"=2.025, "Y"=344.55918367346936}, {"X"=2.033333333333333, "Y"=344.35887096774195}, {"X"=2.0416666666666665, "Y"=343.9469387755102}, {"X"=2.05, "Y"=343.62857142857143}, {"X"=2.058333333333333, "Y"=343.8489795918367}, {"X"=2.066666666666667, "Y"=343.13675213675214}, {"X"=2.075, "Y"=342.55918367346936}, {"X"=2.0833333333333335, "Y"=342.37551020408165}, {"X"=2.091666666666667, "Y"=342.0806451612903}, {"X"=2.1, "Y"=341.7217741935484}, {"X"=2.1083333333333334, "Y"=341.7217741935484}, {"X"=2.1166666666666667, "Y"=340.9717741935484}, {"X"=2.125, "Y"=340.9717741935484}, {"X"=2.1333333333333333, "Y"=340.09274193548384}, {"X"=2.1416666666666666, "Y"=339.6761133603239}, {"X"=2.15, "Y"=339.5748987854251}, {"X"=2.158333333333333, "Y"=339.28163265306125}, {"X"=2.1666666666666665, "Y"=339.356}, {"X"=2.175, "Y"=339.352}, {"X"=2.183333333333333, "Y"=339.3690476190476}, {"X"=2.191666666666667, "Y"=339.425702811245}, {"X"=2.2, "Y"=339.4096385542169}, {"X"=2.2083333333333335, "Y"=339.5381526104418}, {"X"=2.216666666666667, "Y"=339.4837398373984}, {"X"=2.225, "Y"=339.49794238683126}, {"X"=2.2333333333333334, "Y"=340.2510288065844}, {"X"=2.2416666666666667, "Y"=340.2510288065844}, {"X"=2.25, "Y"=340.2832618025751}, {"X"=2.2583333333333333, "Y"=340.2832618025751}, {"X"=2.2666666666666666, "Y"=341.6163793103448}, {"X"=2.275, "Y"=341.9460580912863}, {"X"=2.283333333333333, "Y"=342.40408163265306}, {"X"=2.2916666666666665, "Y"=342.4238683127572}, {"X"=2.3, "Y"=342.9268292682927}, {"X"=2.308333333333333, "Y"=343.3636363636364}, {"X"=2.316666666666667, "Y"=343.74074074074076}, {"X"=2.325, "Y"=344.07851239669424}, {"X"=2.3333333333333335, "Y"=344.44897959183675}, {"X"=2.341666666666667, "Y"=344.275}, {"X"=2.35, "Y"=344.5514403292181}, {"X"=2.3583333333333334, "Y"=344.7975708502024}, {"X"=2.3666666666666667, "Y"=345.0161943319838}, {"X"=2.375, "Y"=345.0161943319838}, {"X"=2.3833333333333333, "Y"=344.5162601626016}, {"X"=2.3916666666666666, "Y"=344.5162601626016}, {"X"=2.4, "Y"=343.90909090909093}, {"X"=2.408333333333333, "Y"=343.71311475409834}, {"X"=2.4166666666666665, "Y"=343.3780487804878}, {"X"=2.425, "Y"=343.1166666666667}, {"X"=2.433333333333333, "Y"=342.61087866108784}, {"X"=2.441666666666667, "Y"=342.58264462809916}, {"X"=2.45, "Y"=341.9230769230769}, {"X"=2.4583333333333335, "Y"=341.5208333333333}, {"X"=2.466666666666667, "Y"=341.18930041152265}, {"X"=2.475, "Y"=340.9105691056911}, {"X"=2.4833333333333334, "Y"=340.4549180327869}, {"X"=2.4916666666666667, "Y"=339.96311475409834}, {"X"=2.5, "Y"=339.9236947791165}, {"X"=2.5083333333333333, "Y"=339.9236947791165}, {"X"=2.5166666666666666, "Y"=339.39676113360326}, {"X"=2.525, "Y"=339.39676113360326}, {"X"=2.533333333333333, "Y"=339.49402390438246}, {"X"=2.5416666666666665, "Y"=339.42971887550203}, {"X"=2.55, "Y"=339.31474103585657}, {"X"=2.558333333333333, "Y"=339.4016064257028}, {"X"=2.566666666666667, "Y"=339.72332015810275}, {"X"=2.575, "Y"=339.93975903614455}, {"X"=2.5833333333333335, "Y"=340.11290322580646}, {"X"=2.591666666666667, "Y"=340.2741935483871}, {"X"=2.6, "Y"=340.72289156626505}, {"X"=2.6083333333333334, "Y"=340.8041666666667}, {"X"=2.6166666666666667, "Y"=341.1470588235294}, {"X"=2.625, "Y"=341.60169491525426}, {"X"=2.6333333333333333, "Y"=341.60169491525426}, {"X"=2.6416666666666666, "Y"=342.235807860262}, {"X"=2.65, "Y"=342.4173913043478}, {"X"=2.658333333333333, "Y"=342.85470085470087}, {"X"=2.6666666666666665, "Y"=343.1908713692946}, {"X"=2.675, "Y"=343.53909465020575}, {"X"=2.683333333333333, "Y"=343.53688524590166}, {"X"=2.691666666666667, "Y"=343.7357723577236}, {"X"=2.7, "Y"=344.0569105691057}, {"X"=2.7083333333333335, "Y"=344.1633466135458}, {"X"=2.716666666666667, "Y"=343.8024691358025}, {"X"=2.725, "Y"=344.03688524590166}, {"X"=2.7333333333333334, "Y"=343.3430962343096}, {"X"=2.7416666666666667, "Y"=343.5163934426229}, {"X"=2.75, "Y"=343.5163934426229}, {"X"=2.7583333333333333, "Y"=343.07053941908714}, {"X"=2.7666666666666666, "Y"=342.7692307692308}, {"X"=2.775, "Y"=342.7692307692308}, {"X"=2.783333333333333, "Y"=342.0663900414938}, {"X"=2.7916666666666665, "Y"=342.0165289256198}, {"X"=2.8, "Y"=342.0617283950617}, {"X"=2.808333333333333, "Y"=341.80497925311204}, {"X"=2.816666666666667, "Y"=341.56722689075633}, {"X"=2.825, "Y"=341.0762711864407}, {"X"=2.8333333333333335, "Y"=341.0769230769231}, {"X"=2.841666666666667, "Y"=340.864406779661}, {"X"=2.85, "Y"=340.7154811715481}, {"X"=2.8583333333333334, "Y"=340.45454545454544}, {"X"=2.8666666666666667, "Y"=340.59591836734694}, {"X"=2.875, "Y"=340.2107438016529}, {"X"=2.8833333333333333, "Y"=340.2107438016529}, {"X"=2.8916666666666666, "Y"=339.849593495935}, {"X"=2.9, "Y"=340.2289156626506}, {"X"=2.908333333333333, "Y"=340.2289156626506}, {"X"=2.9166666666666665, "Y"=340.544}, {"X"=2.925, "Y"=340.96078431372547}, {"X"=2.933333333333333, "Y"=340.788}, {"X"=2.941666666666667, "Y"=341.06299212598424}, {"X"=2.95, "Y"=341.4032258064516}, {"X"=2.9583333333333335, "Y"=341.5265306122449}, {"X"=2.966666666666667, "Y"=341.753036437247}, {"X"=2.975, "Y"=342.0688259109312}, {"X"=2.9833333333333334, "Y"=342.1061224489796}, {"X"=2.9916666666666667, "Y"=342.344262295082}, {"X"=3.0, "Y"=342.4297520661157}, {"X"=3.0083333333333333, "Y"=342.4297520661157}, {"X"=3.0166666666666666, "Y"=342.53679653679654}, {"X"=3.025, "Y"=342.53679653679654}, {"X"=3.033333333333333, "Y"=342.67248908296943}, {"X"=3.0416666666666665, "Y"=343.0}, {"X"=3.05, "Y"=342.6487603305785}, {"X"=3.058333333333333, "Y"=342.8979591836735}, {"X"=3.066666666666667, "Y"=342.4590163934426}, {"X"=3.075, "Y"=342.50205761316874}, {"X"=3.0833333333333335, "Y"=342.39256198347107}, {"X"=3.091666666666667, "Y"=342.3305785123967}, {"X"=3.1, "Y"=342.27385892116183}, {"X"=3.1083333333333334, "Y"=342.4375}, {"X"=3.1166666666666667, "Y"=342.2278481012658}, {"X"=3.125, "Y"=342.02928870292885}, {"X"=3.1333333333333333, "Y"=341.70762711864404}, {"X"=3.1416666666666666, "Y"=341.70762711864404}, {"X"=3.15, "Y"=341.5546218487395}, {"X"=3.158333333333333, "Y"=341.5546218487395}, {"X"=3.1666666666666665, "Y"=341.4897119341564}, {"X"=3.175, "Y"=341.33870967741933}, {"X"=3.183333333333333, "Y"=341.2282157676349}, {"X"=3.191666666666667, "Y"=341.1218487394958}, {"X"=3.2, "Y"=341.125}, {"X"=3.2083333333333335, "Y"=340.8484848484849}, {"X"=3.216666666666667, "Y"=341.0382978723404}, {"X"=3.225, "Y"=341.1308016877637}, {"X"=3.2333333333333334, "Y"=340.9382716049383}, {"X"=3.2416666666666667, "Y"=340.9588477366255}, {"X"=3.25, "Y"=341.4650205761317}, {"X"=3.2583333333333333, "Y"=341.1769547325103}, {"X"=3.2666666666666666, "Y"=341.1769547325103}, {"X"=3.275, "Y"=341.7125506072874}, {"X"=3.283333333333333, "Y"=341.7125506072874}, {"X"=3.2916666666666665, "Y"=341.8577235772358}, {"X"=3.3, "Y"=342.00409836065575}, {"X"=3.308333333333333, "Y"=342.10699588477365}, {"X"=3.316666666666667, "Y"=342.06611570247935}, {"X"=3.325, "Y"=342.2408163265306}, {"X"=3.3333333333333335, "Y"=342.2439024390244}, {"X"=3.341666666666667, "Y"=342.2995951417004}, {"X"=3.35, "Y"=342.5524193548387}, {"X"=3.3583333333333334, "Y"=342.556}, {"X"=3.3666666666666667, "Y"=342.2581967213115}, {"X"=3.375, "Y"=342.3402489626556}, {"X"=3.3833333333333333, "Y"=342.40909090909093}, {"X"=3.3916666666666666, "Y"=342.3539094650206}, {"X"=3.4, "Y"=342.3539094650206}, {"X"=3.408333333333333, "Y"=342.45922746781116}, {"X"=3.4166666666666665, "Y"=342.45922746781116}, {"X"=3.425, "Y"=342.15744680851066}, {"X"=3.433333333333333, "Y"=342.15744680851066}, {"X"=3.441666666666667, "Y"=342.15767634854774}, {"X"=3.45, "Y"=342.0165289256198}, {"X"=3.4583333333333335, "Y"=341.8897959183673}, {"X"=3.466666666666667, "Y"=341.82572614107886}, {"X"=3.475, "Y"=341.7531380753138}, {"X"=3.4833333333333334, "Y"=341.5966386554622}, {"X"=3.4916666666666667, "Y"=341.6502057613169}, {"X"=3.5, "Y"=341.71604938271605}, {"X"=3.5083333333333333, "Y"=341.89669421487605}, {"X"=3.5166666666666666, "Y"=341.8196721311475}, {"X"=3.525, "Y"=341.6188524590164}, {"X"=3.533333333333333, "Y"=341.760162601626}, {"X"=3.5416666666666665, "Y"=341.760162601626}, {"X"=3.55, "Y"=341.72469635627533}, {"X"=3.558333333333333, "Y"=341.5983606557377}, {"X"=3.566666666666667, "Y"=342.0}, {"X"=3.575, "Y"=341.8535564853556}, {"X"=3.5833333333333335, "Y"=341.93333333333334}, {"X"=3.591666666666667, "Y"=341.97457627118644}, {"X"=3.6, "Y"=342.1914893617021}, {"X"=3.6083333333333334, "Y"=342.29957805907173}, {"X"=3.6166666666666667, "Y"=342.12133891213387}, {"X"=3.625, "Y"=341.905737704918}, {"X"=3.6333333333333333, "Y"=342.43145161290323}, {"X"=3.6416666666666666, "Y"=342.40725806451616}, {"X"=3.65, "Y"=342.4837398373984}, {"X"=3.658333333333333, "Y"=341.88284518828453}, {"X"=3.6666666666666665, "Y"=340.4}, {"X"=3.675, "Y"=338.64761904761906}, {"X"=3.683333333333333, "Y"=338.64761904761906}, {"X"=3.691666666666667, "Y"=343.78966789667896}, {"X"=3.7, "Y"=348.3813813813814}, {"X"=3.7083333333333335, "Y"=351.86053412462905}, {"X"=3.716666666666667, "Y"=353.73926380368096}, {"X"=3.725, "Y"=354.815625}, {"X"=3.7333333333333334, "Y"=355.31888544891643}, {"X"=3.7416666666666667, "Y"=355.64119601328906}, {"X"=3.75, "Y"=357.1266233766234}, {"X"=3.7583333333333333, "Y"=357.73926380368096}, {"X"=3.7666666666666666, "Y"=356.9971098265896}, {"X"=3.775, "Y"=354.77971014492755}, {"X"=3.783333333333333, "Y"=354.77971014492755}, {"X"=3.7916666666666665, "Y"=351.437125748503}, {"X"=3.8, "Y"=351.437125748503}, {"X"=3.808333333333333, "Y"=347.89020771513356}, {"X"=3.816666666666667, "Y"=346.21965317919074}, {"X"=3.825, "Y"=344.2122905027933}, {"X"=3.8333333333333335, "Y"=341.88338192419826}, {"X"=3.841666666666667, "Y"=340.0221518987342}, {"X"=3.85, "Y"=338.58245614035087}, {"X"=3.8583333333333334, "Y"=337.4981549815498}, {"X"=3.8666666666666667, "Y"=336.72243346007605}, {"X"=3.875, "Y"=336.53333333333336}, {"X"=3.8833333333333333, "Y"=336.27710843373495}, {"X"=3.8916666666666666, "Y"=336.5022026431718}, {"X"=3.9, "Y"=336.180412371134}, {"X"=3.908333333333333, "Y"=336.180412371134}, {"X"=3.9166666666666665, "Y"=335.7631578947368}, {"X"=3.925, "Y"=335.7631578947368}, {"X"=3.933333333333333, "Y"=336.79411764705884}, {"X"=3.941666666666667, "Y"=336.98148148148147}, {"X"=3.95, "Y"=336.37142857142857}, {"X"=3.9583333333333335, "Y"=335.31176470588235}, {"X"=3.966666666666667, "Y"=334.5257142857143}, {"X"=3.975, "Y"=335.4752475247525}, {"X"=3.9833333333333334, "Y"=336.0219298245614}, {"X"=3.9916666666666667, "Y"=336.4364406779661}, {"X"=4.0, "Y"=336.6111111111111}, {"X"=4.008333333333334, "Y"=337.07251908396944}, {"X"=4.016666666666667, "Y"=338.09285714285716}, {"X"=4.025, "Y"=340.07142857142856}, {"X"=4.033333333333333, "Y"=341.6666666666667}, {"X"=4.041666666666667, "Y"=341.6666666666667}, {"X"=4.05, "Y"=344.4506578947368}, {"X"=4.058333333333334, "Y"=344.4506578947368}, {"X"=4.066666666666666, "Y"=347.9202657807309}, {"X"=4.075, "Y"=349.29794520547944}, {"X"=4.083333333333333, "Y"=350.8211920529801}, {"X"=4.091666666666667, "Y"=351.8277027027027}, {"X"=4.1, "Y"=352.6324503311258}, {"X"=4.108333333333333, "Y"=352.7573770491803}, {"X"=4.116666666666666, "Y"=352.9093851132686}, {"X"=4.125, "Y"=352.1704918032787}, {"X"=4.133333333333334, "Y"=351.6026058631922}, {"X"=4.141666666666667, "Y"=350.7258566978193}, {"X"=4.15, "Y"=348.73186119873816}, {"X"=4.158333333333333, "Y"=347.996875}, {"X"=4.166666666666667, "Y"=346.4143302180685}, {"X"=4.175, "Y"=346.4143302180685}, {"X"=4.183333333333334, "Y"=343.59554140127386}, {"X"=4.191666666666666, "Y"=343.59554140127386}, {"X"=4.2, "Y"=340.8990228013029}, {"X"=4.208333333333333, "Y"=339.8020833333333}, {"X"=4.216666666666667, "Y"=339.0388692579505}, {"X"=4.225, "Y"=338.71102661596956}, {"X"=4.233333333333333, "Y"=338.0}, {"X"=4.241666666666666, "Y"=337.90909090909093}, {"X"=4.25, "Y"=337.58447488584477}, {"X"=4.258333333333334, "Y"=337.8605769230769}, {"X"=4.266666666666667, "Y"=337.87373737373736}, {"X"=4.275, "Y"=337.8729281767956}, {"X"=4.283333333333333, "Y"=338.2044198895028}, {"X"=4.291666666666667, "Y"=337.7305389221557}, {"X"=4.3, "Y"=337.5906432748538}, {"X"=4.308333333333334, "Y"=337.6918604651163}, {"X"=4.316666666666666, "Y"=336.87368421052633}, {"X"=4.325, "Y"=336.88613861386136}, {"X"=4.333333333333333, "Y"=336.8095238095238}, {"X"=4.341666666666667, "Y"=336.76190476190476}, {"X"=4.35, "Y"=336.9}, {"X"=4.358333333333333, "Y"=337.2317073170732}, {"X"=4.366666666666666, "Y"=337.90625}, {"X"=4.375, "Y"=338.8703703703704}, {"X"=4.383333333333334, "Y"=340.45}, {"X"=4.391666666666667, "Y"=340.97872340425533}, {"X"=4.4, "Y"=342.1896551724138}, {"X"=4.408333333333333, "Y"=343.28373702422147}, {"X"=4.416666666666667, "Y"=344.27027027027026}, {"X"=4.425, "Y"=344.27027027027026}, {"X"=4.433333333333334, "Y"=347.45733788395904}, {"X"=4.441666666666666, "Y"=347.45733788395904}, {"X"=4.45, "Y"=348.79505300353355}, {"X"=4.458333333333333, "Y"=349.29655172413794}, {"X"=4.466666666666667, "Y"=349.92957746478874}, {"X"=4.475, "Y"=350.55743243243245}, {"X"=4.483333333333333, "Y"=349.7337883959044}, {"X"=4.491666666666666, "Y"=348.7630662020906}, {"X"=4.5, "Y"=348.28327645051195}, {"X"=4.508333333333334, "Y"=347.43771043771045}, {"X"=4.516666666666667, "Y"=346.3478260869565}, {"X"=4.525, "Y"=345.1756756756757}, {"X"=4.533333333333333, "Y"=344.486301369863}, {"X"=4.541666666666667, "Y"=342.9264214046823}, {"X"=4.55, "Y"=342.9264214046823}, {"X"=4.558333333333334, "Y"=341.2338129496403}, {"X"=4.566666666666666, "Y"=340.8259259259259}, {"X"=4.575, "Y"=339.98837209302326}, {"X"=4.583333333333333, "Y"=339.42412451361866}, {"X"=4.591666666666667, "Y"=339.2098765432099}, {"X"=4.6, "Y"=338.8114754098361}, {"X"=4.608333333333333, "Y"=338.5357142857143}, {"X"=4.616666666666666, "Y"=338.54545454545456}, {"X"=4.625, "Y"=338.54545454545456}, {"X"=4.633333333333334, "Y"=338.6125654450262}, {"X"=4.641666666666667, "Y"=338.77659574468083}, {"X"=4.65, "Y"=338.20652173913044}, {"X"=4.658333333333333, "Y"=338.3101604278075}, {"X"=4.666666666666667, "Y"=338.02139037433153}, {"X"=4.675, "Y"=337.6842105263158}, {"X"=4.683333333333334, "Y"=337.6842105263158}, {"X"=4.691666666666666, "Y"=337.4782608695652}, {"X"=4.7, "Y"=337.4782608695652}, {"X"=4.708333333333333, "Y"=337.49107142857144}, {"X"=4.716666666666667, "Y"=337.7950819672131}, {"X"=4.725, "Y"=338.748031496063}, {"X"=4.733333333333333, "Y"=338.99619771863115}, {"X"=4.741666666666666, "Y"=339.6281588447653}, {"X"=4.75, "Y"=340.90225563909775}, {"X"=4.758333333333334, "Y"=341.4381625441696}, {"X"=4.766666666666667, "Y"=342.3076923076923}, {"X"=4.775, "Y"=343.5483870967742}, {"X"=4.783333333333333, "Y"=344.6725352112676}, {"X"=4.791666666666667, "Y"=345.36462093862815}, {"X"=4.8, "Y"=346.3345070422535}, {"X"=4.808333333333334, "Y"=346.9113475177305}, {"X"=4.816666666666666, "Y"=346.9113475177305}, {"X"=4.825, "Y"=347.95588235294116}, {"X"=4.833333333333333, "Y"=348.5345454545455}, {"X"=4.841666666666667, "Y"=348.07608695652175}, {"X"=4.85, "Y"=347.4892857142857}, {"X"=4.858333333333333, "Y"=347.33449477351917}, {"X"=4.866666666666666, "Y"=346.3859649122807}, {"X"=4.875, "Y"=345.8315789473684}, {"X"=4.883333333333334, "Y"=345.08191126279866}, {"X"=4.891666666666667, "Y"=344.4055944055944}, {"X"=4.9, "Y"=343.0613718411552}, {"X"=4.908333333333333, "Y"=342.5091575091575}, {"X"=4.916666666666667, "Y"=341.6195652173913}, {"X"=4.925, "Y"=341.6195652173913}, {"X"=4.933333333333334, "Y"=340.3560606060606}, {"X"=4.941666666666666, "Y"=339.7578125}, {"X"=4.95, "Y"=339.7578125}, {"X"=4.958333333333333, "Y"=339.1434782608696}, {"X"=4.966666666666667, "Y"=339.1434782608696}, {"X"=4.975, "Y"=339.0607476635514}, {"X"=4.983333333333333, "Y"=338.4682926829268}, {"X"=4.991666666666666, "Y"=338.547263681592}, {"X"=5.0, "Y"=338.42929292929296}, {"X"=5.008333333333334, "Y"=338.5210526315789}, {"X"=5.016666666666667, "Y"=338.37113402061857}, {"X"=5.025, "Y"=338.44102564102565}, {"X"=5.033333333333333, "Y"=337.95477386934675}, {"X"=5.041666666666667, "Y"=338.0047846889952}, {"X"=5.05, "Y"=337.7844036697248}, {"X"=5.058333333333334, "Y"=337.6261261261261}, {"X"=5.066666666666666, "Y"=337.9424778761062}, {"X"=5.075, "Y"=337.9424778761062}, {"X"=5.083333333333333, "Y"=338.93172690763055}, {"X"=5.091666666666667, "Y"=338.93172690763055}, {"X"=5.1, "Y"=339.95238095238096}, {"X"=5.108333333333333, "Y"=340.87640449438203}, {"X"=5.116666666666666, "Y"=341.5830258302583}, {"X"=5.125, "Y"=342.2319391634981}, {"X"=5.133333333333334, "Y"=343.2826086956522}, {"X"=5.141666666666667, "Y"=344.43682310469313}, {"X"=5.15, "Y"=345.14336917562724}, {"X"=5.158333333333333, "Y"=345.7230215827338}, {"X"=5.166666666666667, "Y"=346.43560606060606}, {"X"=5.175, "Y"=346.956678700361}, {"X"=5.183333333333334, "Y"=347.1397058823529}, {"X"=5.191666666666666, "Y"=347.47292418772565}, {"X"=5.2, "Y"=347.47292418772565}, {"X"=5.208333333333333, "Y"=346.99638989169677}, {"X"=5.216666666666667, "Y"=346.7918215613383}, {"X"=5.225, "Y"=346.7918215613383}, {"X"=5.233333333333333, "Y"=345.74911660777383}, {"X"=5.241666666666666, "Y"=344.7335766423358}, {"X"=5.25, "Y"=344.29411764705884}, {"X"=5.258333333333334, "Y"=343.2293233082707}, {"X"=5.266666666666667, "Y"=342.60074626865674}, {"X"=5.275, "Y"=341.70454545454544}, {"X"=5.283333333333333, "Y"=341.30337078651684}, {"X"=5.291666666666667, "Y"=340.7011494252874}, {"X"=5.3, "Y"=339.7171314741036}, {"X"=5.308333333333334, "Y"=339.6333333333333}, {"X"=5.316666666666666, "Y"=339.3125}, {"X"=5.325, "Y"=339.3125}, {"X"=5.333333333333333, "Y"=338.6896551724138}, {"X"=5.341666666666667, "Y"=338.8675799086758}, {"X"=5.35, "Y"=338.8675799086758}, {"X"=5.358333333333333, "Y"=338.28846153846155}, {"X"=5.366666666666666, "Y"=338.47417840375584}, {"X"=5.375, "Y"=338.32535885167465}, {"X"=5.383333333333334, "Y"=338.39195979899495}, {"X"=5.391666666666667, "Y"=338.2047619047619}, {"X"=5.4, "Y"=337.96039603960395}, {"X"=5.408333333333333, "Y"=337.9}, {"X"=5.416666666666667, "Y"=337.68036529680364}, {"X"=5.425, "Y"=338.40851063829786}, {"X"=5.433333333333334, "Y"=338.4765957446809}, {"X"=5.441666666666666, "Y"=338.96}, {"X"=5.45, "Y"=338.96}, {"X"=5.458333333333333, "Y"=340.2164179104478}, {"X"=5.466666666666667, "Y"=340.2164179104478}, {"X"=5.475, "Y"=341.6222222222222}, {"X"=5.483333333333333, "Y"=342.52272727272725}, {"X"=5.491666666666666, "Y"=343.07547169811323}, {"X"=5.5, "Y"=344.0405904059041}, {"X"=5.508333333333334, "Y"=344.99610894941634}, {"X"=5.516666666666667, "Y"=345.7028985507246}, {"X"=5.525, "Y"=346.24163568773236}, {"X"=5.533333333333333, "Y"=346.12109375}, {"X"=5.541666666666667, "Y"=347.03663003663}, {"X"=5.55, "Y"=347.13138686131384}, {"X"=5.558333333333334, "Y"=346.9398496240602}, {"X"=5.566666666666666, "Y"=346.8533834586466}, {"X"=5.575, "Y"=346.4612546125461}, {"X"=5.583333333333333, "Y"=346.4612546125461}, {"X"=5.591666666666667, "Y"=345.3071161048689}, {"X"=5.6, "Y"=344.60820895522386}, {"X"=5.608333333333333, "Y"=343.848}, {"X"=5.616666666666666, "Y"=343.2442748091603}, {"X"=5.625, "Y"=342.6628787878788}, {"X"=5.633333333333334, "Y"=341.97014925373134}, {"X"=5.641666666666667, "Y"=341.48828125}, {"X"=5.65, "Y"=340.56224899598396}, {"X"=5.658333333333333, "Y"=339.9142857142857}, {"X"=5.666666666666667, "Y"=339.6877637130802}, {"X"=5.675, "Y"=339.5940170940171}, {"X"=5.683333333333334, "Y"=339.6}, {"X"=5.691666666666666, "Y"=338.7111111111111}, {"X"=5.7, "Y"=338.3611111111111}, {"X"=5.708333333333333, "Y"=338.3611111111111}, {"X"=5.716666666666667, "Y"=338.6046511627907}, {"X"=5.725, "Y"=338.6046511627907}, {"X"=5.733333333333333, "Y"=338.6}, {"X"=5.741666666666666, "Y"=338.38425925925924}, {"X"=5.75, "Y"=338.16901408450707}, {"X"=5.758333333333334, "Y"=337.9530516431925}, {"X"=5.766666666666667, "Y"=338.36199095022624}, {"X"=5.775, "Y"=338.7787610619469}, {"X"=5.783333333333333, "Y"=338.91150442477874}, {"X"=5.791666666666667, "Y"=339.15611814345993}, {"X"=5.8, "Y"=339.61507936507934}, {"X"=5.808333333333334, "Y"=339.9714285714286}, {"X"=5.816666666666666, "Y"=340.70703125}, {"X"=5.825, "Y"=341.3968871595331}, {"X"=5.833333333333333, "Y"=342.0980392156863}, {"X"=5.841666666666667, "Y"=342.73880597014926}, {"X"=5.85, "Y"=342.73880597014926}, {"X"=5.858333333333333, "Y"=343.98501872659176}, {"X"=5.866666666666666, "Y"=344.96875}, {"X"=5.875, "Y"=345.37827715355803}, {"X"=5.883333333333334, "Y"=345.8745247148289}, {"X"=5.891666666666667, "Y"=346.06439393939394}, {"X"=5.9, "Y"=346.0153256704981}, {"X"=5.908333333333333, "Y"=346.3657587548638}, {"X"=5.916666666666667, "Y"=346.171875}, {"X"=5.925, "Y"=346.02661596958177}, {"X"=5.933333333333334, "Y"=345.69083969465646}, {"X"=5.941666666666666, "Y"=345.3308270676692}, {"X"=5.95, "Y"=345.0380228136882}, {"X"=5.958333333333333, "Y"=345.0380228136882}, {"X"=5.966666666666667, "Y"=343.29615384615386}, {"X"=5.975, "Y"=343.29615384615386}, {"X"=5.983333333333333, "Y"=341.8452830188679}, {"X"=5.991666666666666, "Y"=341.4826254826255}, {"X"=6.0, "Y"=340.59375}, {"X"=6.008333333333334, "Y"=340.2642276422764}, {"X"=6.016666666666667, "Y"=339.79423868312756}, {"X"=6.025, "Y"=339.41632653061225}, {"X"=6.033333333333333, "Y"=338.71120689655174}, {"X"=6.041666666666667, "Y"=338.69545454545454}, {"X"=6.05, "Y"=338.6336206896552}, {"X"=6.058333333333334, "Y"=338.80269058295966}, {"X"=6.066666666666666, "Y"=338.61971830985914}, {"X"=6.075, "Y"=338.88584474885846}, {"X"=6.083333333333333, "Y"=338.77314814814815}, {"X"=6.091666666666667, "Y"=338.77314814814815}, {"X"=6.1, "Y"=338.8493150684931}, {"X"=6.108333333333333, "Y"=338.8867924528302}, {"X"=6.116666666666666, "Y"=338.98617511520735}, {"X"=6.125, "Y"=339.09417040358744}, {"X"=6.133333333333334, "Y"=339.47435897435895}, {"X"=6.141666666666667, "Y"=339.47435897435895}, {"X"=6.15, "Y"=340.22633744855966}, {"X"=6.158333333333333, "Y"=340.75206611570246}, {"X"=6.166666666666667, "Y"=340.9504132231405}, {"X"=6.175, "Y"=341.7051792828685}, {"X"=6.183333333333334, "Y"=341.8828125}, {"X"=6.191666666666666, "Y"=342.7837837837838}, {"X"=6.2, "Y"=343.25096525096524}, {"X"=6.208333333333333, "Y"=343.82745098039214}, {"X"=6.216666666666667, "Y"=344.132}, {"X"=6.225, "Y"=345.0627450980392}, {"X"=6.233333333333333, "Y"=345.0627450980392}, {"X"=6.241666666666666, "Y"=345.39080459770116}, {"X"=6.25, "Y"=345.58365758754866}, {"X"=6.258333333333334, "Y"=345.4653846153846}, {"X"=6.266666666666667, "Y"=345.8178294573643}, {"X"=6.275, "Y"=345.8030303030303}, {"X"=6.283333333333333, "Y"=345.4465648854962}, {"X"=6.291666666666667, "Y"=345.1547619047619}, {"X"=6.3, "Y"=344.3190661478599}, {"X"=6.308333333333334, "Y"=343.73046875}, {"X"=6.316666666666666, "Y"=343.18918918918916}, {"X"=6.325, "Y"=342.515625}, {"X"=6.333333333333333, "Y"=342.15234375}, {"X"=6.341666666666667, "Y"=342.15234375}, {"X"=6.35, "Y"=341.04938271604937}, {"X"=6.358333333333333, "Y"=341.04938271604937}, {"X"=6.366666666666666, "Y"=339.7883817427386}, {"X"=6.375, "Y"=339.7883817427386}, {"X"=6.383333333333334, "Y"=338.8091286307054}, {"X"=6.391666666666667, "Y"=338.9475982532751}, {"X"=6.4, "Y"=338.88646288209605}, {"X"=6.408333333333333, "Y"=338.9869565217391}, {"X"=6.416666666666667, "Y"=338.7085201793722}, {"X"=6.425, "Y"=339.0488888888889}, {"X"=6.433333333333334, "Y"=338.868778280543}, {"X"=6.441666666666666, "Y"=338.6792452830189}, {"X"=6.45, "Y"=339.13615023474176}, {"X"=6.458333333333333, "Y"=339.5315315315315}, {"X"=6.466666666666667, "Y"=339.3796296296296}, {"X"=6.475, "Y"=339.6140350877193}, {"X"=6.483333333333333, "Y"=339.52863436123346}, {"X"=6.491666666666666, "Y"=340.0720338983051}, {"X"=6.5, "Y"=340.35135135135135}, {"X"=6.508333333333334, "Y"=341.24590163934425}, {"X"=6.516666666666667, "Y"=341.7081545064378}, {"X"=6.525, "Y"=341.89112903225805}, {"X"=6.533333333333333, "Y"=342.1847389558233}, {"X"=6.541666666666667, "Y"=342.33067729083666}, {"X"=6.55, "Y"=342.68163265306123}, {"X"=6.558333333333334, "Y"=343.61867704280155}, {"X"=6.566666666666666, "Y"=343.798418972332}, {"X"=6.575, "Y"=344.44787644787647}, {"X"=6.583333333333333, "Y"=344.6756756756757}, {"X"=6.591666666666667, "Y"=344.5925925925926}, {"X"=6.6, "Y"=344.5925925925926}, {"X"=6.608333333333333, "Y"=345.54135338345867}, {"X"=6.616666666666666, "Y"=345.54135338345867}, {"X"=6.625, "Y"=345.41984732824426}, {"X"=6.633333333333334, "Y"=345.30651340996167}, {"X"=6.641666666666667, "Y"=344.292}, {"X"=6.65, "Y"=344.35769230769233}, {"X"=6.658333333333333, "Y"=344.00763358778624}, {"X"=6.666666666666667, "Y"=343.54545454545456}, {"X"=6.675, "Y"=342.85114503816794}, {"X"=6.683333333333334, "Y"=342.36821705426354}, {"X"=6.691666666666666, "Y"=341.77016129032256}, {"X"=6.7, "Y"=341.1333333333333}, {"X"=6.708333333333333, "Y"=340.87044534412956}, {"X"=6.716666666666667, "Y"=340.26693227091636}, {"X"=6.725, "Y"=339.46153846153845}, {"X"=6.733333333333333, "Y"=339.46153846153845}, {"X"=6.741666666666666, "Y"=339.344262295082}, {"X"=6.75, "Y"=338.94827586206895}, {"X"=6.758333333333334, "Y"=338.94827586206895}, {"X"=6.766666666666667, "Y"=338.96}, {"X"=6.775, "Y"=338.81974248927037}, {"X"=6.783333333333333, "Y"=339.4052863436123}, {"X"=6.791666666666667, "Y"=339.08597285067873}, {"X"=6.8, "Y"=339.09722222222223}, {"X"=6.808333333333334, "Y"=339.33488372093024}, {"X"=6.816666666666666, "Y"=339.6606334841629}, {"X"=6.825, "Y"=339.95535714285717}, {"X"=6.833333333333333, "Y"=340.14932126696834}, {"X"=6.841666666666667, "Y"=340.61206896551727}, {"X"=6.85, "Y"=340.79574468085104}, {"X"=6.858333333333333, "Y"=341.2067510548523}, {"X"=6.866666666666666, "Y"=341.57201646090533}, {"X"=6.875, "Y"=341.57201646090533}, {"X"=6.883333333333334, "Y"=341.7717842323651}, {"X"=6.891666666666667, "Y"=342.18145161290323}, {"X"=6.9, "Y"=342.17622950819674}, {"X"=6.908333333333333, "Y"=343.0398406374502}, {"X"=6.916666666666667, "Y"=343.0398406374502}, {"X"=6.925, "Y"=343.8}, {"X"=6.933333333333334, "Y"=343.98837209302326}, {"X"=6.941666666666666, "Y"=344.62745098039215}, {"X"=6.95, "Y"=344.5984555984556}, {"X"=6.958333333333333, "Y"=344.69260700389106}, {"X"=6.966666666666667, "Y"=344.7707509881423}, {"X"=6.975, "Y"=344.46946564885496}, {"X"=6.983333333333333, "Y"=344.47011952191235}, {"X"=6.991666666666666, "Y"=344.47011952191235}, {"X"=7.0, "Y"=344.0038314176245}, {"X"=7.008333333333334, "Y"=343.78846153846155}, {"X"=7.016666666666667, "Y"=343.2655601659751}, {"X"=7.025, "Y"=342.6144578313253}, {"X"=7.033333333333333, "Y"=342.82608695652175}, {"X"=7.041666666666667, "Y"=342.1843137254902}, {"X"=7.05, "Y"=341.632}, {"X"=7.058333333333334, "Y"=341.33858267716533}, {"X"=7.066666666666666, "Y"=341.0987654320988}, {"X"=7.075, "Y"=340.7578125}, {"X"=7.083333333333333, "Y"=340.53061224489795}, {"X"=7.091666666666667, "Y"=340.1781376518219}, {"X"=7.1, "Y"=340.1781376518219}, {"X"=7.108333333333333, "Y"=339.48458149779736}, {"X"=7.116666666666666, "Y"=339.48458149779736}, {"X"=7.125, "Y"=339.54741379310343}, {"X"=7.133333333333334, "Y"=339.50228310502285}, {"X"=7.141666666666667, "Y"=339.51785714285717}, {"X"=7.15, "Y"=339.82758620689657}, {"X"=7.158333333333333, "Y"=340.1030042918455}, {"X"=7.166666666666667, "Y"=340.00881057268725}, {"X"=7.175, "Y"=340.2246696035242}, {"X"=7.183333333333334, "Y"=340.3083700440529}, {"X"=7.191666666666666, "Y"=340.46875}, {"X"=7.2, "Y"=340.4035087719298}, {"X"=7.208333333333333, "Y"=340.55364806866953}, {"X"=7.216666666666667, "Y"=341.25847457627117}, {"X"=7.225, "Y"=340.982905982906}, {"X"=7.233333333333333, "Y"=341.66390041493776}, {"X"=7.241666666666666, "Y"=341.66390041493776}, {"X"=7.25, "Y"=342.134693877551}, {"X"=7.258333333333334, "Y"=342.134693877551}, {"X"=7.266666666666667, "Y"=342.5529411764706}, {"X"=7.275, "Y"=342.9442231075697}, {"X"=7.283333333333333, "Y"=343.1699604743083}, {"X"=7.291666666666667, "Y"=343.4921875}, {"X"=7.3, "Y"=343.6692913385827}, {"X"=7.308333333333334, "Y"=343.86821705426354}, {"X"=7.316666666666666, "Y"=343.79457364341084}, {"X"=7.325, "Y"=343.77911646586347}, {"X"=7.333333333333333, "Y"=343.9140625}, {"X"=7.341666666666667, "Y"=343.9268292682927}, {"X"=7.35, "Y"=344.0241935483871}, {"X"=7.358333333333333, "Y"=343.5863453815261}, {"X"=7.366666666666666, "Y"=343.472}, {"X"=7.375, "Y"=343.472}, {"X"=7.383333333333334, "Y"=342.7991967871486}, {"X"=7.391666666666667, "Y"=342.7991967871486}, {"X"=7.4, "Y"=342.0438247011952}, {"X"=7.408333333333333, "Y"=342.14112903225805}, {"X"=7.416666666666667, "Y"=341.80971659919027}, {"X"=7.425, "Y"=341.80971659919027}, {"X"=7.433333333333334, "Y"=341.3050193050193}, {"X"=7.441666666666666, "Y"=340.4959677419355}, {"X"=7.45, "Y"=340.58995815899584}, {"X"=7.458333333333333, "Y"=340.3636363636364}, {"X"=7.466666666666667, "Y"=340.2572614107884}, {"X"=7.475, "Y"=339.831223628692}, {"X"=7.483333333333333, "Y"=339.97095435684645}, {"X"=7.491666666666666, "Y"=339.52941176470586}, {"X"=7.5, "Y"=339.8086956521739}, {"X"=7.508333333333334, "Y"=339.84090909090907}, {"X"=7.516666666666667, "Y"=339.84090909090907}, {"X"=7.525, "Y"=339.96875}, {"X"=7.533333333333333, "Y"=339.98230088495575}, {"X"=7.541666666666667, "Y"=340.3348017621145}, {"X"=7.55, "Y"=340.16818181818184}, {"X"=7.558333333333334, "Y"=340.4069264069264}, {"X"=7.566666666666666, "Y"=340.75}, {"X"=7.575, "Y"=340.57456140350877}, {"X"=7.583333333333333, "Y"=340.7284482758621}, {"X"=7.591666666666667, "Y"=341.02608695652174}, {"X"=7.6, "Y"=341.13304721030045}, {"X"=7.608333333333333, "Y"=341.5406504065041}, {"X"=7.616666666666666, "Y"=341.551867219917}, {"X"=7.625, "Y"=341.551867219917}, {"X"=7.633333333333334, "Y"=342.2090163934426}, {"X"=7.641666666666667, "Y"=342.27755102040817}, {"X"=7.65, "Y"=342.37301587301585}, {"X"=7.658333333333333, "Y"=342.4756097560976}, {"X"=7.666666666666667, "Y"=342.76771653543307}, {"X"=7.675, "Y"=343.51171875}, {"X"=7.683333333333334, "Y"=343.7716535433071}, {"X"=7.691666666666666, "Y"=343.6860465116279}, {"X"=7.7, "Y"=343.7003891050584}, {"X"=7.708333333333333, "Y"=343.7265625}, {"X"=7.716666666666667, "Y"=343.712}, {"X"=7.725, "Y"=343.8473282442748}, {"X"=7.733333333333333, "Y"=342.984}, {"X"=7.741666666666666, "Y"=342.984}, {"X"=7.75, "Y"=342.92578125}, {"X"=7.758333333333334, "Y"=342.92578125}, {"X"=7.766666666666667, "Y"=342.14741035856576}, {"X"=7.775, "Y"=342.46963562753035}, {"X"=7.783333333333333, "Y"=342.281124497992}, {"X"=7.791666666666667, "Y"=341.31983805668017}, {"X"=7.8, "Y"=340.54811715481173}, {"X"=7.808333333333334, "Y"=341.0386266094421}, {"X"=7.816666666666666, "Y"=341.20425531914896}, {"X"=7.825, "Y"=340.04366812227073}, {"X"=7.833333333333333, "Y"=339.9059829059829}, {"X"=7.841666666666667, "Y"=340.2928870292887}, {"X"=7.85, "Y"=339.6735537190083}, {"X"=7.858333333333333, "Y"=339.2938596491228}, {"X"=7.866666666666666, "Y"=339.0468085106383}, {"X"=7.875, "Y"=339.0468085106383}, {"X"=7.883333333333334, "Y"=338.7354260089686}, {"X"=7.891666666666667, "Y"=338.7354260089686}, {"X"=7.9, "Y"=339.1484716157205}, {"X"=7.908333333333333, "Y"=339.2914798206278}, {"X"=7.916666666666667, "Y"=339.08898305084745}, {"X"=7.925, "Y"=339.27659574468083}, {"X"=7.933333333333334, "Y"=339.2274678111588}, {"X"=7.941666666666666, "Y"=339.55648535564853}, {"X"=7.95, "Y"=339.4177215189873}, {"X"=7.958333333333333, "Y"=340.1975308641975}, {"X"=7.966666666666667, "Y"=340.7642276422764}, {"X"=7.975, "Y"=340.48163265306124}, {"X"=7.983333333333333, "Y"=340.3625498007968}, {"X"=7.991666666666666, "Y"=341.4448818897638}, {"X"=8.0, "Y"=341.8192771084337}, {"X"=8.008333333333333, "Y"=341.8192771084337}, {"X"=8.016666666666667, "Y"=342.19444444444446}, {"X"=8.025, "Y"=342.19444444444446}, {"X"=8.033333333333333, "Y"=342.0409836065574}, {"X"=8.041666666666666, "Y"=342.64478764478764}, {"X"=8.05, "Y"=342.45}, {"X"=8.058333333333334, "Y"=342.47755102040816}, {"X"=8.066666666666666, "Y"=342.18145161290323}, {"X"=8.075, "Y"=342.3319502074689}, {"X"=8.083333333333334, "Y"=342.2520325203252}, {"X"=8.091666666666667, "Y"=342.19354838709677}, {"X"=8.1, "Y"=342.3607843137255}, {"X"=8.108333333333333, "Y"=341.8360655737705}, {"X"=8.116666666666667, "Y"=341.9392712550607}, {"X"=8.125, "Y"=341.3790322580645}, {"X"=8.133333333333333, "Y"=341.3174603174603}, {"X"=8.141666666666667, "Y"=341.3174603174603}, {"X"=8.15, "Y"=340.3333333333333}, {"X"=8.158333333333333, "Y"=340.3333333333333}, {"X"=8.166666666666666, "Y"=339.6761133603239}, {"X"=8.175, "Y"=339.23651452282155}, {"X"=8.183333333333334, "Y"=339.0169491525424}, {"X"=8.191666666666666, "Y"=339.30125523012555}, {"X"=8.2, "Y"=338.9734513274336}, {"X"=8.208333333333334, "Y"=338.72340425531917}, {"X"=8.216666666666667, "Y"=338.83700440528634}, {"X"=8.225, "Y"=338.7763713080169}, {"X"=8.233333333333333, "Y"=338.929203539823}, {"X"=8.241666666666667, "Y"=339.0}, {"X"=8.25, "Y"=339.18502202643174}, {"X"=8.258333333333333, "Y"=339.2703862660944}, {"X"=8.266666666666667, "Y"=339.2703862660944}, {"X"=8.275, "Y"=339.1806167400881}, {"X"=8.283333333333333, "Y"=339.1181434599156}, {"X"=8.291666666666666, "Y"=339.1181434599156}, {"X"=8.3, "Y"=339.5652173913044}, {"X"=8.308333333333334, "Y"=339.647577092511}, {"X"=8.316666666666666, "Y"=340.53846153846155}, {"X"=8.325, "Y"=340.34156378600824}, {"X"=8.333333333333334, "Y"=340.44303797468353}, {"X"=8.341666666666667, "Y"=340.6348547717842}, {"X"=8.35, "Y"=341.3168724279835}, {"X"=8.358333333333333, "Y"=341.7470355731225}, {"X"=8.366666666666667, "Y"=341.96385542168673}, {"X"=8.375, "Y"=342.1604938271605}, {"X"=8.383333333333333, "Y"=342.292}, {"X"=8.391666666666667, "Y"=342.4347826086956}, {"X"=8.4, "Y"=342.7421875}, {"X"=8.408333333333333, "Y"=342.7421875}, {"X"=8.416666666666666, "Y"=342.7269076305221}, {"X"=8.425, "Y"=342.8366533864542}, {"X"=8.433333333333334, "Y"=342.60956175298804}, {"X"=8.441666666666666, "Y"=342.4212598425197}, {"X"=8.45, "Y"=342.4745098039216}, {"X"=8.458333333333334, "Y"=342.21311475409834}, {"X"=8.466666666666667, "Y"=342.1566265060241}, {"X"=8.475, "Y"=341.594262295082}, {"X"=8.483333333333333, "Y"=341.14574898785423}, {"X"=8.491666666666667, "Y"=341.12598425196853}, {"X"=8.5, "Y"=340.70472440944883}, {"X"=8.508333333333333, "Y"=340.70472440944883}, {"X"=8.516666666666667, "Y"=339.72244897959183}, {"X"=8.525, "Y"=339.3673469387755}, {"X"=8.533333333333333, "Y"=339.3673469387755}, {"X"=8.541666666666666, "Y"=338.7763157894737}, {"X"=8.55, "Y"=339.03478260869565}, {"X"=8.558333333333334, "Y"=338.9163179916318}, {"X"=8.566666666666666, "Y"=338.6666666666667}, {"X"=8.575, "Y"=338.5378151260504}, {"X"=8.583333333333334, "Y"=338.6434782608696}, {"X"=8.591666666666667, "Y"=338.7345132743363}, {"X"=8.6, "Y"=338.85833333333335}, {"X"=8.608333333333333, "Y"=338.7621145374449}, {"X"=8.616666666666667, "Y"=338.6222222222222}, {"X"=8.625, "Y"=338.74122807017545}, {"X"=8.633333333333333, "Y"=338.6519823788546}, {"X"=8.641666666666667, "Y"=338.6519823788546}, {"X"=8.65, "Y"=339.1911111111111}, {"X"=8.658333333333333, "Y"=339.24463519313304}, {"X"=8.666666666666666, "Y"=339.24463519313304}, {"X"=8.675, "Y"=339.7991631799163}, {"X"=8.683333333333334, "Y"=340.33613445378154}, {"X"=8.691666666666666, "Y"=340.6595744680851}, {"X"=8.7, "Y"=341.0403225806452}, {"X"=8.708333333333334, "Y"=341.369918699187}, {"X"=8.716666666666667, "Y"=342.0557768924303}, {"X"=8.725, "Y"=341.90983606557376}, {"X"=8.733333333333333, "Y"=342.5}, {"X"=8.741666666666667, "Y"=342.34939759036143}, {"X"=8.75, "Y"=342.80392156862746}, {"X"=8.758333333333333, "Y"=342.84705882352944}, {"X"=8.766666666666667, "Y"=342.7857142857143}, {"X"=8.775, "Y"=342.7857142857143}, {"X"=8.783333333333333, "Y"=342.8346153846154}, {"X"=8.791666666666666, "Y"=342.8346153846154}, {"X"=8.8, "Y"=342.6235294117647}, {"X"=8.808333333333334, "Y"=342.24380165289256}, {"X"=8.816666666666666, "Y"=342.204}, {"X"=8.825, "Y"=341.90983606557376}, {"X"=8.833333333333334, "Y"=341.9372549019608}, {"X"=8.841666666666667, "Y"=341.74285714285713}, {"X"=8.85, "Y"=341.10460251046027}, {"X"=8.858333333333333, "Y"=340.18672199170123}, {"X"=8.866666666666667, "Y"=340.1551020408163}, {"X"=8.875, "Y"=340.0983606557377}, {"X"=8.883333333333333, "Y"=339.6194331983806}, {"X"=8.891666666666667, "Y"=339.11538461538464}, {"X"=8.9, "Y"=339.11538461538464}, {"X"=8.908333333333333, "Y"=338.82832618025753}, {"X"=8.916666666666666, "Y"=338.8109243697479}, {"X"=8.925, "Y"=338.8109243697479}, {"X"=8.933333333333334, "Y"=338.90909090909093}, {"X"=8.941666666666666, "Y"=339.11607142857144}, {"X"=8.95, "Y"=337.85897435897436}, {"X"=8.958333333333334, "Y"=337.85897435897436}, {"X"=8.966666666666667, "Y"=338.83613445378154}, {"X"=8.975, "Y"=338.8914027149321}, {"X"=8.983333333333333, "Y"=337.991341991342}, {"X"=8.991666666666667, "Y"=339.11344537815125}, {"X"=9.0, "Y"=339.46491228070175}, {"X"=9.008333333333333, "Y"=339.1814345991561}, {"X"=9.016666666666667, "Y"=338.7136563876652}, {"X"=9.025, "Y"=339.43153526970957}, {"X"=9.033333333333333, "Y"=340.5528455284553}, {"X"=9.041666666666666, "Y"=340.4225941422594}, {"X"=9.05, "Y"=340.30212765957447}, {"X"=9.058333333333334, "Y"=341.64940239043824}, {"X"=9.066666666666666, "Y"=342.09716599190284}, {"X"=9.075, "Y"=341.7336065573771}, {"X"=9.083333333333334, "Y"=342.4497991967871}, {"X"=9.091666666666667, "Y"=343.2142857142857}, {"X"=9.1, "Y"=343.2142857142857}, {"X"=9.108333333333333, "Y"=342.7193675889328}, {"X"=9.116666666666667, "Y"=343.3897637795276}, {"X"=9.125, "Y"=343.9268292682927}, {"X"=9.133333333333333, "Y"=343.2540322580645}, {"X"=9.141666666666667, "Y"=342.844}, {"X"=9.15, "Y"=343.4724409448819}, {"X"=9.158333333333333, "Y"=343.4724409448819}, {"X"=9.166666666666666, "Y"=342.9484126984127}, {"X"=9.175, "Y"=342.7628458498024}, {"X"=9.183333333333334, "Y"=342.7628458498024}, {"X"=9.191666666666666, "Y"=342.4979919678715}, {"X"=9.2, "Y"=341.82}, {"X"=9.208333333333334, "Y"=341.69444444444446}, {"X"=9.216666666666667, "Y"=341.88582677165357}, {"X"=9.225, "Y"=340.9710743801653}, {"X"=9.233333333333333, "Y"=340.56485355648533}, {"X"=9.241666666666667, "Y"=340.5469387755102}, {"X"=9.25, "Y"=340.35}, {"X"=9.258333333333333, "Y"=339.88702928870293}, {"X"=9.266666666666667, "Y"=339.38818565400845}, {"X"=9.275, "Y"=339.5064935064935}, {"X"=9.283333333333333, "Y"=339.5064935064935}, {"X"=9.291666666666666, "Y"=339.3948497854077}, {"X"=9.3, "Y"=339.10869565217394}, {"X"=9.308333333333334, "Y"=339.10869565217394}, {"X"=9.316666666666666, "Y"=339.1409691629956}, {"X"=9.325, "Y"=339.2586206896552}, {"X"=9.333333333333334, "Y"=339.3608695652174}, {"X"=9.341666666666667, "Y"=339.3974358974359}, {"X"=9.35, "Y"=339.83690987124464}, {"X"=9.358333333333333, "Y"=339.44635193133047}, {"X"=9.366666666666667, "Y"=339.5594713656388}, {"X"=9.375, "Y"=340.698347107438}, {"X"=9.383333333333333, "Y"=341.0}, {"X"=9.391666666666667, "Y"=340.61632653061224}, {"X"=9.4, "Y"=340.679012345679}, {"X"=9.408333333333333, "Y"=340.679012345679}, {"X"=9.416666666666666, "Y"=341.9510204081633}, {"X"=9.425, "Y"=341.79423868312756}, {"X"=9.433333333333334, "Y"=341.79423868312756}, {"X"=9.441666666666666, "Y"=342.65714285714284}, {"X"=9.45, "Y"=342.7211155378486}, {"X"=9.458333333333334, "Y"=342.8359375}, {"X"=9.466666666666667, "Y"=343.116}, {"X"=9.475, "Y"=343.3807692307692}, {"X"=9.483333333333333, "Y"=343.08984375}, {"X"=9.491666666666667, "Y"=343.07003891050584}, {"X"=9.5, "Y"=343.0194552529183}, {"X"=9.508333333333333, "Y"=342.984126984127}, {"X"=9.516666666666667, "Y"=342.6008064516129}, {"X"=9.525, "Y"=342.6008064516129}, {"X"=9.533333333333333, "Y"=342.65354330708664}, {"X"=9.541666666666666, "Y"=342.43673469387755}, {"X"=9.55, "Y"=342.43673469387755}, {"X"=9.558333333333334, "Y"=342.0408163265306}, {"X"=9.566666666666666, "Y"=342.0408163265306}, {"X"=9.575, "Y"=341.31020408163266}, {"X"=9.583333333333334, "Y"=340.797520661157}, {"X"=9.591666666666667, "Y"=341.0381355932203}, {"X"=9.6, "Y"=340.4227642276423}, {"X"=9.608333333333333, "Y"=340.40416666666664}, {"X"=9.616666666666667, "Y"=339.836820083682}, {"X"=9.625, "Y"=339.79295154185024}, {"X"=9.633333333333333, "Y"=340.34599156118145}, {"X"=9.641666666666667, "Y"=339.59656652360513}, {"X"=9.65, "Y"=339.9917355371901}, {"X"=9.658333333333333, "Y"=340.30801687763716}, {"X"=9.666666666666666, "Y"=340.30801687763716}, {"X"=9.675, "Y"=339.97446808510637}, {"X"=9.683333333333334, "Y"=340.21940928270044}, {"X"=9.691666666666666, "Y"=340.21940928270044}, {"X"=9.7, "Y"=339.987012987013}, {"X"=9.708333333333334, "Y"=340.364406779661}, {"X"=9.716666666666667, "Y"=340.2139737991266}, {"X"=9.725, "Y"=340.73221757322176}, {"X"=9.733333333333333, "Y"=340.5}, {"X"=9.741666666666667, "Y"=340.7489711934156}, {"X"=9.75, "Y"=340.65800865800867}, {"X"=9.758333333333333, "Y"=341.1398305084746}, {"X"=9.766666666666667, "Y"=341.43673469387755}, {"X"=9.775, "Y"=341.41224489795917}, {"X"=9.783333333333333, "Y"=341.7551867219917}, {"X"=9.791666666666666, "Y"=342.0242914979757}, {"X"=9.8, "Y"=342.0242914979757}, {"X"=9.808333333333334, "Y"=342.10887096774195}, {"X"=9.816666666666666, "Y"=342.10887096774195}, {"X"=9.825, "Y"=342.8804780876494}, {"X"=9.833333333333334, "Y"=342.8857142857143}, {"X"=9.841666666666667, "Y"=342.64426877470356}, {"X"=9.85, "Y"=342.66932270916334}, {"X"=9.858333333333333, "Y"=342.864}, {"X"=9.866666666666667, "Y"=342.6324110671937}, {"X"=9.875, "Y"=342.59362549800795}, {"X"=9.883333333333333, "Y"=342.31075697211156}, {"X"=9.891666666666667, "Y"=342.31075697211156}, {"X"=9.9, "Y"=342.1475409836066}, {"X"=9.908333333333333, "Y"=341.991935483871}, {"X"=9.916666666666666, "Y"=342.0123966942149}, {"X"=9.925, "Y"=341.91269841269843}, {"X"=9.933333333333334, "Y"=341.91269841269843}, {"X"=9.941666666666666, "Y"=340.9504132231405}, {"X"=9.95, "Y"=340.8137651821862}, {"X"=9.958333333333334, "Y"=340.8137651821862}, {"X"=9.966666666666667, "Y"=340.86345381526104}, {"X"=9.975, "Y"=340.559670781893}, {"X"=9.983333333333333, "Y"=340.55982905982904}, {"X"=9.991666666666667, "Y"=340.1794871794872}, {"X"=10.0, "Y"=340.23809523809524}, {"X"=10.008333333333333, "Y"=340.3491379310345}, {"X"=10.016666666666667, "Y"=340.0464135021097}, {"X"=10.025, "Y"=339.8242677824268}, {"X"=10.033333333333333, "Y"=340.156378600823}, {"X"=10.041666666666666, "Y"=340.1410788381743}, {"X"=10.05, "Y"=340.0775510204082}, {"X"=10.058333333333334, "Y"=340.17391304347825}, {"X"=10.066666666666666, "Y"=340.17391304347825}, {"X"=10.075, "Y"=340.3813559322034}, {"X"=10.083333333333334, "Y"=340.5215517241379}, {"X"=10.091666666666667, "Y"=340.4375}, {"X"=10.1, "Y"=340.5807860262009}, {"X"=10.108333333333333, "Y"=340.67330677290835}, {"X"=10.116666666666667, "Y"=340.7615062761506}, {"X"=10.125, "Y"=341.2931034482759}, {"X"=10.133333333333333, "Y"=341.43775100401604}, {"X"=10.141666666666667, "Y"=341.36213991769546}, {"X"=10.15, "Y"=341.8204081632653}, {"X"=10.158333333333333, "Y"=341.72469635627533}, {"X"=10.166666666666666, "Y"=342.4859437751004}, {"X"=10.175, "Y"=341.9756097560976}, {"X"=10.183333333333334, "Y"=341.9756097560976}, {"X"=10.191666666666666, "Y"=342.65098039215684}, {"X"=10.2, "Y"=342.65098039215684}, {"X"=10.208333333333334, "Y"=342.3467741935484}, {"X"=10.216666666666667, "Y"=342.43621399176953}, {"X"=10.225, "Y"=342.2217741935484}, {"X"=10.233333333333333, "Y"=342.6023622047244}, {"X"=10.241666666666667, "Y"=342.546875}, {"X"=10.25, "Y"=342.546875}, {"X"=10.258333333333333, "Y"=342.21311475409834}, {"X"=10.266666666666667, "Y"=342.2008032128514}, {"X"=10.275, "Y"=342.2572614107884}, {"X"=10.283333333333333, "Y"=341.9681274900398}, {"X"=10.291666666666666, "Y"=341.7193675889328}, {"X"=10.3, "Y"=341.4586776859504}, {"X"=10.308333333333334, "Y"=341.5487804878049}, {"X"=10.316666666666666, "Y"=341.268}, {"X"=10.325, "Y"=341.268}, {"X"=10.333333333333334, "Y"=341.02834008097165}, {"X"=10.341666666666667, "Y"=340.8143459915612}, {"X"=10.35, "Y"=340.6523605150215}, {"X"=10.358333333333333, "Y"=341.0163934426229}, {"X"=10.366666666666667, "Y"=340.73799126637556}, {"X"=10.375, "Y"=340.1694915254237}, {"X"=10.383333333333333, "Y"=340.2025316455696}, {"X"=10.391666666666667, "Y"=340.36213991769546}, {"X"=10.4, "Y"=340.55510204081634}, {"X"=10.408333333333333, "Y"=340.55230125523013}, {"X"=10.416666666666666, "Y"=340.24675324675326}, {"X"=10.425, "Y"=340.54468085106384}, {"X"=10.433333333333334, "Y"=340.54468085106384}, {"X"=10.441666666666666, "Y"=340.3776824034335}, {"X"=10.45, "Y"=340.3776824034335}, {"X"=10.458333333333334, "Y"=340.80252100840335}, {"X"=10.466666666666667, "Y"=340.80252100840335}, {"X"=10.475, "Y"=340.53688524590166}, {"X"=10.483333333333333, "Y"=340.89495798319325}, {"X"=10.491666666666667, "Y"=340.90725806451616}, {"X"=10.5, "Y"=340.9387755102041}, {"X"=10.508333333333333, "Y"=341.25099601593627}, {"X"=10.516666666666667, "Y"=341.48192771084337}, {"X"=10.525, "Y"=342.0436507936508}, {"X"=10.533333333333333, "Y"=341.9362549800797}, {"X"=10.541666666666666, "Y"=341.90551181102364}, {"X"=10.55, "Y"=342.4824902723735}, {"X"=10.558333333333334, "Y"=342.16}, {"X"=10.566666666666666, "Y"=342.55335968379444}, {"X"=10.575, "Y"=342.55335968379444}, {"X"=10.583333333333334, "Y"=342.6521739130435}, {"X"=10.591666666666667, "Y"=342.6521739130435}, {"X"=10.6, "Y"=342.5546875}, {"X"=10.608333333333333, "Y"=342.4331983805668}, {"X"=10.616666666666667, "Y"=342.76209677419354}, {"X"=10.625, "Y"=342.085020242915}, {"X"=10.633333333333333, "Y"=342.10843373493975}, {"X"=10.641666666666667, "Y"=342.316}, {"X"=10.65, "Y"=342.28629032258067}, {"X"=10.658333333333333, "Y"=341.6694214876033}, {"X"=10.666666666666666, "Y"=341.0}, {"X"=10.675, "Y"=341.5101214574899}, {"X"=10.683333333333334, "Y"=342.4008097165992}, {"X"=10.691666666666666, "Y"=341.22131147540983}, {"X"=10.7, "Y"=340.7617021276596}, {"X"=10.708333333333334, "Y"=340.7617021276596}, {"X"=10.716666666666667, "Y"=341.390756302521}, {"X"=10.725, "Y"=340.3491379310345}, {"X"=10.733333333333333, "Y"=340.1386554621849}, {"X"=10.741666666666667, "Y"=341.1101694915254}, {"X"=10.75, "Y"=340.9710743801653}, {"X"=10.758333333333333, "Y"=339.49159663865544}, {"X"=10.766666666666667, "Y"=339.5042016806723}, {"X"=10.775, "Y"=340.2173913043478}, {"X"=10.783333333333333, "Y"=339.6455696202532}, {"X"=10.791666666666666, "Y"=338.99555555555554}, {"X"=10.8, "Y"=339.8728813559322}, {"X"=10.808333333333334, "Y"=340.1124497991968}, {"X"=10.816666666666666, "Y"=339.15677966101697}, {"X"=10.825, "Y"=339.15677966101697}, {"X"=10.833333333333334, "Y"=340.1422764227642}, {"X"=10.841666666666667, "Y"=340.38396624472574}, {"X"=10.85, "Y"=339.8809523809524}, {"X"=10.858333333333333, "Y"=339.61087866108784}, {"X"=10.866666666666667, "Y"=340.56972111553785}, {"X"=10.875, "Y"=340.7654320987654}, {"X"=10.883333333333333, "Y"=340.7470355731225}, {"X"=10.891666666666667, "Y"=341.07287449392715}, {"X"=10.9, "Y"=341.45}, {"X"=10.908333333333333, "Y"=341.16279069767444}, {"X"=10.916666666666666, "Y"=341.35849056603774}, {"X"=10.925, "Y"=341.82213438735175}, {"X"=10.933333333333334, "Y"=342.0282258064516}, {"X"=10.941666666666666, "Y"=342.06477732793525}, {"X"=10.95, "Y"=341.9571984435798}, {"X"=10.958333333333334, "Y"=341.9571984435798}, {"X"=10.966666666666667, "Y"=342.0443548387097}, {"X"=10.975, "Y"=341.94262295081967}, {"X"=10.983333333333333, "Y"=342.140562248996}, {"X"=10.991666666666667, "Y"=342.11914893617023}, {"X"=11.0, "Y"=342.01612903225805}, {"X"=11.008333333333333, "Y"=341.34387351778656}, {"X"=11.016666666666667, "Y"=341.2857142857143}, {"X"=11.025, "Y"=341.9186991869919}, {"X"=11.033333333333333, "Y"=341.35833333333335}, {"X"=11.041666666666666, "Y"=341.0517928286853}, {"X"=11.05, "Y"=341.31120331950206}, {"X"=11.058333333333334, "Y"=341.1260162601626}, {"X"=11.066666666666666, "Y"=340.96638655462186}, {"X"=11.075, "Y"=340.96638655462186}, {"X"=11.083333333333334, "Y"=340.6144578313253}, {"X"=11.091666666666667, "Y"=340.6144578313253}, {"X"=11.1, "Y"=340.0300429184549}, {"X"=11.108333333333333, "Y"=339.38260869565215}, {"X"=11.116666666666667, "Y"=339.6794871794872}, {"X"=11.125, "Y"=339.9113924050633}, {"X"=11.133333333333333, "Y"=339.36401673640165}, {"X"=11.141666666666667, "Y"=339.3648068669528}, {"X"=11.15, "Y"=339.3434782608696}, {"X"=11.158333333333333, "Y"=339.69456066945605}, {"X"=11.166666666666666, "Y"=339.28691983122366}, {"X"=11.175, "Y"=339.2459677419355}, {"X"=11.183333333333334, "Y"=339.55510204081634}, {"X"=11.191666666666666, "Y"=339.7967479674797}, {"X"=11.2, "Y"=339.4}, {"X"=11.208333333333334, "Y"=339.4}, {"X"=11.216666666666667, "Y"=340.14344262295083}, {"X"=11.225, "Y"=340.14344262295083}, {"X"=11.233333333333333, "Y"=340.10330578512395}, {"X"=11.241666666666667, "Y"=340.8339920948617}, {"X"=11.25, "Y"=341.0080971659919}, {"X"=11.258333333333333, "Y"=340.7890625}, {"X"=11.266666666666667, "Y"=340.7015503875969}, {"X"=11.275, "Y"=341.4}, {"X"=11.283333333333333, "Y"=341.6640316205534}, {"X"=11.291666666666666, "Y"=341.5595238095238}, {"X"=11.3, "Y"=341.7290076335878}, {"X"=11.308333333333334, "Y"=341.99609375}, {"X"=11.316666666666666, "Y"=341.60557768924303}, {"X"=11.325, "Y"=341.59274193548384}, {"X"=11.333333333333334, "Y"=342.0281124497992}, {"X"=11.341666666666667, "Y"=342.0281124497992}, {"X"=11.35, "Y"=341.4979079497908}, {"X"=11.358333333333333, "Y"=341.12048192771084}, {"X"=11.366666666666667, "Y"=341.32530120481925}, {"X"=11.375, "Y"=341.4763779527559}, {"X"=11.383333333333333, "Y"=341.2113821138211}, {"X"=11.391666666666667, "Y"=341.2113821138211}, {"X"=11.4, "Y"=340.7609561752988}, {"X"=11.408333333333333, "Y"=340.761316872428}, {"X"=11.416666666666666, "Y"=340.5528455284553}, {"X"=11.425, "Y"=340.7457627118644}, {"X"=11.433333333333334, "Y"=340.46153846153845}, {"X"=11.441666666666666, "Y"=340.43933054393307}, {"X"=11.45, "Y"=339.93305439330544}, {"X"=11.458333333333334, "Y"=340.0331950207469}, {"X"=11.466666666666667, "Y"=339.9670781893004}, {"X"=11.475, "Y"=339.7296137339056}, {"X"=11.483333333333333, "Y"=339.68220338983053}, {"X"=11.491666666666667, "Y"=339.8835341365462}, {"X"=11.5, "Y"=340.74583333333334}, {"X"=11.508333333333333, "Y"=341.25581395348837}, {"X"=11.516666666666667, "Y"=341.6640625}, {"X"=11.525, "Y"=341.3413654618474}, {"X"=11.533333333333333, "Y"=340.52542372881356}, {"X"=11.541666666666666, "Y"=340.12295081967216}, {"X"=11.55, "Y"=341.1607843137255}, {"X"=11.558333333333334, "Y"=341.77510040160644}, {"X"=11.566666666666666, "Y"=341.7560975609756}, {"X"=11.575, "Y"=340.796875}, {"X"=11.583333333333334, "Y"=340.655601659751}, {"X"=11.591666666666667, "Y"=340.92712550607285}, {"X"=11.6, "Y"=342.255905511811}, {"X"=11.608333333333333, "Y"=341.78823529411767}, {"X"=11.616666666666667, "Y"=340.559670781893}, {"X"=11.625, "Y"=340.62978723404257}, {"X"=11.633333333333333, "Y"=340.8833333333333}, {"X"=11.641666666666667, "Y"=341.64166666666665}, {"X"=11.65, "Y"=341.68595041322317}, {"X"=11.658333333333333, "Y"=341.05737704918033}, {"X"=11.666666666666666, "Y"=340.82278481012656}, {"X"=11.675, "Y"=341.4599156118143}, {"X"=11.683333333333334, "Y"=341.2764227642276}, {"X"=11.691666666666666, "Y"=341.5136186770428}, {"X"=11.7, "Y"=340.9596774193548}, {"X"=11.708333333333334, "Y"=340.4181034482759}, {"X"=11.716666666666667, "Y"=340.9237288135593}, {"X"=11.725, "Y"=341.336}, {"X"=11.733333333333333, "Y"=340.99196787148594}, {"X"=11.741666666666667, "Y"=341.49612403100775}, {"X"=11.75, "Y"=340.59055118110234}, {"X"=11.758333333333333, "Y"=340.7731092436975}, {"X"=11.766666666666667, "Y"=341.25}, {"X"=11.775, "Y"=341.428}, {"X"=11.783333333333333, "Y"=341.2510288065844}, {"X"=11.791666666666666, "Y"=341.077868852459}, {"X"=11.8, "Y"=341.0590717299578}, {"X"=11.808333333333334, "Y"=340.5514403292181}, {"X"=11.816666666666666, "Y"=340.780487804878}, {"X"=11.825, "Y"=341.828}, {"X"=11.833333333333334, "Y"=342.18039215686275}, {"X"=11.841666666666667, "Y"=342.5263157894737}, {"X"=11.85, "Y"=339.4475806451613}, {"X"=11.858333333333333, "Y"=340.01702127659576}]
  out "image":picture
  in  "threshold":cluster{u8, u8}(slide)={151, 255} scale=0.0..255.0
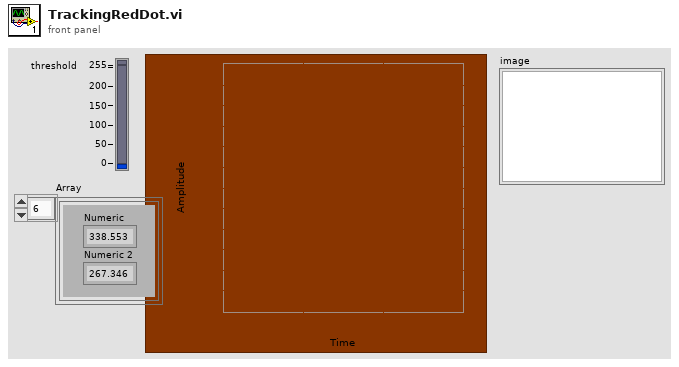
[diagram p1: front panel]
types:
  T1 = typedef "QT_Image.ctl" = cluster{"Width":i32, "Height":i32, "Depth":i32, "data":u8[], "Compressed data":u8[], "Color table":u32[], "Duration":i32, "Options":i32, "Timestamp":i32, "ID":i32, "Reserved":i32, "Dialogs":u32}
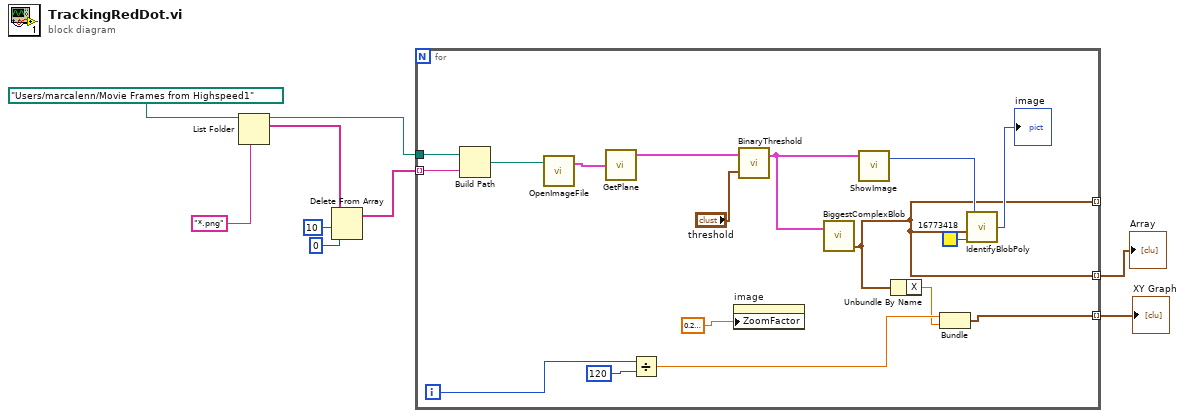
[diagram p0: block diagram]
diagram:
  n1 = List Folder(path=path "/Users/marcalenn/Movie Frames from Highspeed1", pattern="*.png") -> (path out=w8:path, filenames=w6:string[])  [unwired: 2 in, 2 out]
  n2 = Delete From Array(array=w6, length=10, index=0) -> (array with subset deleted=w5:string[])  [unwired: 1 out]
  n3 = for {
    tunnel: w8 -> [w23]
    tunnel: w5 -> [w22] mode=indexing
    tunnel: [w11] -> w2 mode=indexing
    tunnel: [w10] -> _ mode=indexing
    tunnel: [w10] -> w1 mode=indexing
    i -> [w15]
    n4 = Build Path(base path=w23, name or relative path=w22) -> (appended path=w18:path)
    n5 = call <userlib>:"OpenImageFile.vi"("selected path"=w18) -> ("Image Out"=w17:T1)  [unwired: 2 in]
    n6 = call <userlib>:"GetPlane.vi"("Image In"=w17) -> ("Red Plane Out"=w26:T1)  [unwired: 2 out]
    n7 = Divide(x=w15, y=120) -> (x/y=w13:dbl)
    n8 = property on="image" class="Pict"("ZoomFactor"=sgl 0.2 ("Zoom Factor")) -> ()  [unwired: 2 in, 2 out]
    n9 = call <userlib>:"BinaryThreshold.vi"("threshold"="threshold", "Image In"=w26) -> ("Image Out"=w24:T1)  [unwired: 1 in]
    n10 = call <userlib>:"BiggestComplexBlob.vi"("Image in"=w24) -> ("Centroid"=w10:cluster{"X":dbl, "Y":dbl})  [unwired: 1 in, 2 out]
    n11 = call <userlib>:"ShowImage.vi"("Image"=w24) -> ("image"=w20:picture)  [unwired: 2 in, 1 out]
    n12 = Unbundle By Name(w10) -> ("X"=w12:dbl)
    n13 = Bundle(w13, "X"=w12) -> (w11:cluster{dbl, "X":dbl})  [unwired: 1 in]
    n14 = call-poly <userlib>:"IdentifyBlobPoly.vi"("color"=u32 16773418, "Centroid"=w10, "picture"=w20) -> ("picture"=→"image":picture)  [unwired: 1 in]
  }
  "XY Graph" <- w2
  "Array" <- w1
